vi "cesium_controller.vi"() -> ()   [LabVIEW 2013]
doc: "This is the main code used to run experiments in the Cesium laboratory of Mark Saffman. It was written by Martin Lichtman from 2009 to 2012, with DDS drivers written by Alex Gill and Larry Isenhower.\n\nEach hardware section may be enabled and disabled separately. Experiments will finish when all hardware has completed, or when the \"experiment timeout\" is reached, whichever comes first."
uses:
  <vilib>/Utility/error.llb/DialogType.ctl
  <vilib>/Utility/file.llb/Read From Spreadsheet File (string).vi
  <vilib>/Utility/file.llb/Write To Spreadsheet File (string).vi
  Camera/Hamamatsu_C9100-13/Hamamatsu_C9100-13.lvclass
  Experiment/Experiment.lvclass
  DDS/DDS.lvclass
  gui_refnum.ctl
  Counter/counter_graph_refnums.ctl
  gui_execution_controls.ctl
  ExperimentVariables/Variable_Settings.ctl
  ExperimentVariables/ExperimentVariables.lvclass
  <instrlib>/niHSDIO/niHSDIO.llb/niHSDIO_ctl Trigger Script - trigID Values (Ring).ctl
  <instrlib>/niHSDIO/niHSDIO.llb/niHSDIO_ctl Trigger Source Values (Ring).ctl
  <instrlib>/niHSDIO/niHSDIO.llb/niHSDIO_ctl Trigger DigEdge - Edge Values (Ring).ctl
  <instrlib>/niHSDIO/niHSDIO.llb/niHSDIO_ctl Trigger DigLvl - Level Values (Ring).ctl
  HSDIO/HSDIO_settings.ctl
  HSDIO/HSDIO.lvclass
  DAQmx_pulse_out/settings.ctl
  DAQmx_pulse_out/DAQmx_pulse_out.lvclass
  <vilib>/ni845x/ni845x.llb/ni845xControl.ctl
  DDS drivers v3/DDS_box_device_reference.ctl
  DDS drivers v3/DDS RAM mode.ctl
  DDS drivers v3/DDS_box_cluster.ctl
  DDS drivers v3/Array_of_DDS_Boxes.ctl
  DDS/DDS_Settings_Cluster.ctl
  Camera/Hamamatsu_C9100-13/camera_setup.ctl
  Counter/Counter_Settings_Control.ctl
  Counter/Counter.lvclass
  filters/filters.ctl
  Analog_output/AO_settings.ctl
  Analog_output/Analog_Output.lvclass
  config_file_io/all_settings.ctl
  GPIB/HP83623A_RF_Generator/HP83623A_RF_Generator.lvclass
  GPIB/HP83623A_RF_Generator/HP83623A_array.ctl
  PI_piezo/PI_Piezo.lvclass
  PI_piezo/settings.ctl
  Camera/Andor/Andor_settings.ctl
  <vilib>/gmath/NI_Gmath.lvlib
  gui/measurement_graph.ctl
  GPIB/HP8662A_RF_Generator/HP8662A_RF_Generator.lvclass
  GPIB/RF_Generator_settings.ctl
  GPIB/GPIB.lvclass
  GPIB/RF_Generator_settings_array.ctl
  DDS drivers v3/DDS_profile.ctl
  DDS drivers v3/DDS_channel.ctl
  DDS drivers v3/array_of_DDS_profiles.ctl
  DDS drivers v3/array_of_DDS_channels.ctl
  GPIB/HP83712B_RF_Generator/HP83712B_RF_Generator.lvclass
  TTL_input/TTL_input_settings.ctl
  TTL_input/TTL_input.lvclass
  HSDIO/waveform.ctl
  Experiment/Globals.vi
  <vilib>/Utility/file.llb/Write To Spreadsheet File (DBL).vi
  PI_piezo/piezo_channel.ctl
  PI_piezo/piezo_controller.ctl
  GPIB/HP83623A_RF_Generator/HP83623A.ctl
  histogram.ctl
  PI_piezo/status.ctl
panel:
  out "laser unlocked":bool
  out "Paused after Measurement":bool
  in  "Continue":bool
  in  "Pause after Iteration":bool
  out "Paused after Iteration":bool
  in  "Save Settings":bool
  in  "Load Settings":bool
  out "Background Array":u16[][](array[numeric])
  in  "Pause after Measurement":bool
  in  "Quit Program":bool
  in  "Run Experiment":bool
  in  "Tab Control":T1(tab)
  out "Variables (Indicator)":string[][](table)=[["a", "0.000", "0", "9172.612"], ["b", "0.000", "0", "9192.632"], ["k6", "0.000", "0", "0.100"], ["d", "2.000", "10", "40.000"]]
  out "Total Iterations":u32=11
  out "Current Iteration":u32=10
  out "Current measurement":u32=99
  out "wait loops":u32=42 caption="loops while waiting for \nexperiment to complete"
  in  "Log":string="2013-06-14 18:41:57 Experiment ended\n\n2013-06-14 18:41:38 Saving log.\n\n2013-06-14 18:13:43 Experiment started\n\n2013-06-14 17:57:15 Experiment ended\n\n2013-06-14 17:56:56 Saving log.\n\n2013-06-14 17:43:06 Experiment started\n\n2013-06-14 17:24:56 Experiment ended\n\n2013-06-14 17:24:35 Saving log.\n\n2013-06-14 17:10:22 Experiment started\n\n2013-06-14 17:05:48 Experiment ended\n\n2013-06-14 17:05:28 Experiment started\n\n2013-06-14 16:54:16 Experiment ended\n\n2013-06-14 16:52:09 Experiment started\n\n2013-06-14 16:47:56 Experiment ended\n\n2013-06-14 16:45:44 Experiment started\n\n2013-06-14 16:45:42 Experiment ended\n\n2013-06-14 16:43:02 Experiment started\n\n2013-06-14 16:43:01 Experiment ended\n\n2013-06-14 16:42:47 Saving log.\n\n2013-06-14 16:34:29 Experiment started\n\n2013-06-14 16:31:17 Experiment ended\n\n2013-06-14 16:30:59 Saving log.\n\n2013-06-14 16:17:10 Experiment started\n\n2013-06-14 16:17:09 Experiment ended\n\n2013-06-14 16:17:02 Saving log.\n\n2013-06-14 16:16:34 Experiment started\n\n2013-06-14 16:06:13 Experiment ended\n\n2013-06-14 16:06:06 Saving log.\n\n2013-06-14 15:58:25 Experiment started\n\n2013-06-14 15:48:18 Experiment ended\n\n2013-06-14 15:47:53 Experiment started\n\n2013-06-14 15:47:47 Experiment ended\n\n2013-06-14 15:47:28 Experiment started\n\n2013-06-14 15:47:27 Experiment ended\n\n2013-06-14 15:47:11 Experiment started\n\n2013-06-14 15:47:07 Experiment ended\n\n2013-06-14 15:46:48 Experiment started\n\n2013-06-14 15:46:35 Experiment ended\n\n2013-06-14 15:46:15 Experiment started\n\n2013-06-14 15:46:11 Experiment ended\n\n2013-06-14 15:38:57 Experiment started\n\n2013-06-14 15:37:18 Experiment ended\n\n2013-06-14 15:36:58 Experiment started\n\n2013-06-14 15:36:56 Experiment ended\n\n2013-06-14 15:35:05 Experiment started\n\n2013-06-14 15:35:04 Experiment ended\n\n2013-06-14 15:34:46 Experiment started\n\n2013-06-14 15:30:55 Experiment ended\n\n2013-06-14 15:30:47 Saving log.\n\n2013-06-14 15:29:21 Experiment started\n\n2013-06-14 15:29:20 Experiment ended\n\n2013-06-14 15:28:00 Experiment started\n\n2013-06-14 15:27:15 Experiment ended\n\n2013-06-14 15:26:46 Experiment started\n\n2013-06-14 15:25:16 Experiment ended\n\n2013-06-14 15:24:42 Experiment started\n\n2013-06-14 15:23:44 Experiment ended\n\n2013-06-14 15:23:14 Experiment started\n\n2013-06-14 15:22:27 Experiment ended\n\n2013-06-14 15:22:05 Experiment started\n\n2013-06-14 15:21:52 Error cleared and continued by user\n\n2013-06-14 15:21:49 Error -1074115612 occurred at niHSDIO Write Script.vi\r\n\r\nPossible reason(s):\nDriver Status:  (Hex 0xBFFA4BE4) Keyword was expected, but not found in the script.\n\nLine Number: 54\nPosition in Line: 1\nBad Value: compressredGenerate\nPossible Keywords: end\n\nStatus Code: -200027\nCall chain:\nhandle_errors.vi cesium_controller.vi\r\n\n\n2013-06-14 15:21:49 Experiment ended\n\n2013-06-14 15:21:43 Saving log.\n\n2013-06-14 15:21:22 Experiment started\n\n2013-06-14 15:20:53 Experiment ended\n\n2013-06-14 15:20:29 Experiment started\n\n2013-06-14 15:19:36 Experiment ended\n\n2013-06-14 15:18:32 Experiment started\n\n2013-06-14 15:15:07 Experiment ended\n\n2013-06-14 15:14:57 Saving log.\n\n2013-06-14 15:09:28 Experiment started\n\n2013-06-14 15:08:32 Experiment ended\n\n2013-06-14 15:08:22 Saving log.\n\n2013-06-14 15:03:52 Experiment started\n\n2013-06-14 14:59:10 Experiment ended\n\n2013-06-14 14:58:58 Saving log.\n\n2013-06-14 14:52:07 Experiment started\n\n2013-06-14 14:51:15 Experiment ended\n\n2013-06-14 14:51:04 Saving log.\n\n2013-06-14 14:44:44 Experiment started\n\n2013-06-14 14:44:39 Experiment ended\n\n2013-06-14 14:44:25 Saving log.\n\n2013-06-14 14:33:47 Experiment started\n\n2013-06-14 14:32:54 Error cleared and continued by user\n\n2013-06-14 14:32:53 Error -23091 occurred at Inconsistency in variables or numbers\r\n\r\nPossible reason(s):\n\r\nAnalysis:  Inconsistency in variables or numbers.\nCall chain:\nhandle_errors.vi cesium_controller.vi\r\n\n\n2013-06-14 14:32:38 Error cleared and continued by user\n\n2013-06-14 14:32:32 Error -23091 occurred at Inconsistency in variables or numbers\r\n\r\nPossible reason(s):\n\r\nAnalysis:  Inconsistency in variables or numbers.\nCall chain:\nhandle_errors.vi cesium_controller.vi\r\n\n\n2013-06-14 14:31:17 Error cleared and continued by user\n\n2013-06-14 14:31:16 Error -23091 occurred at Inconsistency in variables or numbers\r\n\r\nPossible reason(s):\n\r\nAnalysis:  Inconsistency in variables or numbers.\nCall chain:\nhandle_errors.vi cesium_controller.vi\r\n\n\n2013-06-14 14:31:16 Error cleared and continued by user\n\n2013-06-14 14:31:12 Error -23091 occurred at Inconsistency in variables or numbers\r\n\r\nPossible reason(s):\n\r\nAnalysis:  Inconsistency in variables or numbers.\nCall chain:\nhandle_errors.vi cesium_controller.vi\r\n\n\n2013-06-14 14:30:06 Error cleared and continued by user\n\n2013-06-14 14:29:53 Error -23091 occurred at Inconsistency in variables or numbers\r\n\r\nPossible reason(s):\n\r\nAnalysis:  Inconsistency in variables or numbers.\nCall chain:\nhandle_errors.vi cesium_controller.vi\r\n\n\n2013-06-14 14:29:53 Experiment ended\n\n2013-06-14 14:29:47 Saving log.\n\n2013-06-14 14:29:43 Experiment started\n\n2013-06-14 14:26:56 Error cleared and continued by user\n\n2013-06-14 14:26:55 Error -23091 occurred at Inconsistency in variables or numbers\r\n\r\nPossible reason(s):\n\r\nAnalysis:  Inconsistency in variables or numbers.\nCall chain:\nhandle_errors.vi cesium_controller.vi\r\n\n\n2013-06-14 14:26:37 Error cleared and continued by user\n\n2013-06-14 14:26:28 Error -23091 occurred at Inconsistency in variables or numbers\r\n\r\nPossible reason(s):\n\r\nAnalysis:  Inconsistency in variables or numbers.\nCall chain:\nhandle_errors.vi cesium_controller.vi\r\n\n\n2013-06-14 14:24:46 Error cleared and continued by user\n\n2013-06-14 14:24:44 Error -23091 occurred at Inconsistency in variables or numbers\r\n\r\nPossible reason(s):\n\r\nAnalysis:  Inconsistency in variables or numbers.\nCall chain:\nhandle_errors.vi cesium_controller.vi\r\n\n\n2013-06-14 14:24:44 Experiment ended\n\n2013-06-14 14:24:38 Saving log.\n\n2013-06-14 14:24:36 Experiment started\n\n2013-06-14 14:24:18 Error cleared and continued by user\n\n2013-06-14 14:24:16 Error -23091 occurred at Inconsistency in variables or numbers\r\n\r\nPossible reason(s):\n\r\nAnalysis:  Inconsistency in variables or numbers.\nCall chain:\nhandle_errors.vi cesium_controller.vi\r\n\n\n2013-06-14 14:24:07 Error cleared and continued by user\n\n2013-06-14 14:24:04 Error -23091 occurred at Inconsistency in variables or numbers\r\n\r\nPossible reason(s):\n\r\nAnalysis:  Inconsistency in variables or numbers.\nCall chain:\nhandle_errors.vi cesium_controller.vi\r\n\n\n2013-06-14 14:14:57 Experiment ended\n\n2013-06-14 14:14:41 Saving log.\n\n2013-06-14 14:01:54 Experiment started\n\n2013-06-14 14:01:45 Experiment ended\n\n2013-06-14 14:01:28 Saving log.\n\n2013-06-14 13:47:44 Experiment started\n\n2013-06-14 13:41:39 Experiment ended\n\n2013-06-14 13:41:31 Saving log.\n\n2013-06-14 13:39:59 Experiment started\n\n2013-06-14 13:39:57 Experiment ended\n\n2013-06-14 13:39:50 Saving log.\n\n2013-06-14 13:38:17 Experiment started\n\n2013-06-14 13:25:54 Experiment ended\n\n2013-06-14 13:25:39 Saving log.\n\n2013-06-14 13:14:23 Experiment started\n\n2013-06-14 13:01:58 Experiment ended\n\n2013-06-14 13:01:39 Saving log.\n\n2013-06-14 12:46:16 Experiment started\n\n2013-06-14 12:36:06 Experiment ended\n\n2013-06-14 12:35:53 Saving log.\n\n2013-06-14 12:28:42 Experiment started\n\n2013-06-14 12:20:45 Experiment ended\n\n2013-06-14 12:20:37 Saving log.\n\n2013-06-14 12:19:04 Experiment started\n\n2013-06-14 12:14:08 Experiment ended\n\n2013-06-14 12:14:00 Saving log.\n\n2013-06-14 12:12:31 Experiment started\n\n2013-06-14 12:12:30 Experiment ended\n\n2013-06-14 12:00:34 Experiment started\n\n2013-06-14 11:57:46 Experiment ended\n\n2013-06-14 11:57:38 Saving log.\n\n2013-06-14 11:56:10 Experiment started\n\n2013-06-14 11:47:52 Experiment ended\n\n2013-06-14 11:47:44 Saving log.\n\n2013-06-14 11:46:18 Experiment started\n\n2013-06-14 10:06:01 Experiment ended\n\n2013-06-14 10:05:53 Saving log.\n\n2013-06-14 10:04:24 Experiment started\n\n2013-06-14 10:01:43 Experiment ended\n\n2013-06-14 10:01:02 Experiment started\n\n2013-06-14 10:00:58 Experiment ended\n\n2013-06-14 10:00:35 Experiment started\n\n2013-06-14 08:10:42 Experiment ended\n\n2013-06-14 08:10:20 Experiment started\n\n2013-06-14 08:09:56 Experiment ended\n\n2013-06-14 08:08:35 Experiment started\n\n2013-06-14 08:08:06 Experiment ended\n\n2013-06-14 08:07:44 Experiment started\n\n2013-06-14 07:58:21 Experiment ended\n\n2013-06-14 07:51:44 Experiment started\n\n2013-06-13 21:30:01 Experiment ended\n\n2013-06-13 21:29:35 Experiment started\n\n2013-06-13 21:29:31 Experiment ended\n\n2013-06-13 21:29:05 Experiment started\n\n2013-06-13 21:28:52 Experiment ended\n\n2013-06-13 21:28:29 Experiment started\n\n2013-06-13 21:28:26 Experiment ended\n\n2013-06-13 21:28:05 Experiment started\n\n2013-06-13 21:26:16 Experiment ended\n\n2013-06-13 21:25:49 Experiment started\n\n2013-06-13 21:25:39 Experiment ended\n\n2013-06-13 21:25:13 Experiment started\n\n2013-06-13 21:25:12 Experiment ended\n\n2013-06-13 21:24:51 Experiment started\n\n2013-06-13 21:24:48 Experiment ended\n\n2013-06-13 21:24:26 Experiment started\n\n2013-06-13 21:24:15 Experiment ended\n\n2013-06-13 21:23:50 Experiment started\n\n2013-06-13 21:23:37 Experiment ended\n\n2013-06-13 21:23:15 Experiment started\n\n2013-06-13 21:23:14 Experiment ended\n\n2013-06-13 21:22:51 Experiment started\n\n2013-06-13 21:22:42 Experiment ended\n\n2013-06-13 21:22:19 Experiment started\n\n2013-06-13 21:22:18 Experiment ended\n\n2013-06-13 21:21:56 Experiment started\n\n2013-06-13 21:21:53 Experiment ended\n\n2013-06-13 21:21:17 Experiment started\n\n2013-06-13 21:21:17 Experiment ended\n\n2013-06-13 21:20:56 Experiment started\n\n2013-06-13 21:20:56 Experiment ended\n\n2013-06-13 21:20:32 Experiment started\n\n2013-06-13 21:20:29 Experiment ended\n\n2013-06-13 21:17:58 Experiment started\n\n2013-06-13 21:17:48 Experiment ended\n\n2013-06-13 21:04:43 Experiment started\n\n2013-06-13 21:04:41 Experiment ended\n\n2013-06-13 20:50:48 Experiment started\n\n2013-06-13 20:50:35 Experiment ended\n\n2013-06-13 20:50:02 Experiment started\n\n2013-06-13 20:49:42 Experiment ended\n\n2013-06-13 20:48:06 Experiment started\n\n2013-06-13 20:47:30 Experiment ended\n\n2013-06-13 20:45:37 Experiment started\n\n2013-06-13 20:45:31 Experiment ended\n\n2013-06-13 20:31:50 Experiment started\n\n2013-06-13 20:29:58 Experiment ended\n\n2013-06-13 20:27:00 Experiment started\n\n2013-06-13 20:26:57 Experiment ended\n\n2013-06-13 20:11:15 Experiment started\n\n2013-06-13 20:11:13 Experiment ended\n\n2013-06-13 20:09:50 Experiment started\n\n2013-06-13 20:09:33 Experiment ended\n\n2013-06-13 20:03:38 Experiment started\n\n2013-06-13 20:03:25 Experiment ended\n\n2013-06-13 20:03:19 Saving log.\n\n2013-06-13 20:01:48 Experiment started\n\n2013-06-13 20:01:48 Experiment ended\n\n2013-06-13 19:57:41 Experiment started\n\n2013-06-13 19:57:40 Experiment ended\n\n2013-06-13 19:53:03 Experiment started\n\n2013-06-13 19:52:47 Experiment ended\n\n2013-06-13 19:52:01 Experiment started\n\n2013-06-13 19:51:26 Experiment ended\n\n2013-06-13 19:51:00 Experiment started\n\n2013-06-13 19:49:32 Experiment ended\n\n2013-06-13 19:46:50 Experiment started\n\n2013-06-13 19:46:42 Experiment ended\n\n2013-06-13 19:46:17 Experiment started\n\n2013-06-13 19:46:11 Experiment ended\n\n2013-06-13 19:45:40 Experiment started\n\n2013-06-13 19:45:39 Experiment ended\n\n2013-06-13 19:45:16 Experiment started\n\n2013-06-13 19:45:04 Experiment ended\n\n2013-06-13 19:44:37 Experiment started\n\n2013-06-13 19:44:36 Experiment ended\n\n2013-06-13 19:44:07 Experiment started\n\n2013-06-13 19:44:02 Experiment ended\n\n2013-06-13 19:43:37 Experiment started\n\n2013-06-13 19:43:33 Experiment ended\n\n2013-06-13 19:39:17 Experiment started\n\n2013-06-13 19:39:07 Experiment ended\n\n2013-06-13 19:38:47 Experiment started\n\n2013-06-13 19:38:45 Experiment ended\n\n2013-06-13 19:38:24 Experiment started\n\n2013-06-13 19:38:23 Experiment ended\n\n2013-06-13 19:37:59 Experiment started\n\n2013-06-13 19:37:26 Experiment ended\n\n2013-06-13 19:36:47 Experiment started\n\n2013-06-13 19:36:39 Experiment ended\n\n2013-06-13 19:36:17 Experiment started\n\n2013-06-13 19:36:13 Experiment ended\n\n2013-06-13 19:35:50 Experiment started\n\n2013-06-13 19:35:47 Experiment ended\n\n2013-06-13 19:35:21 Experiment started\n\n2013-06-13 19:35:18 Experiment ended\n\n2013-06-13 19:34:55 Experiment started\n\n2013-06-13 19:34:50 Experiment ended\n\n2013-06-13 19:34:28 Experiment started\n\n2013-06-13 19:34:20 Experiment ended\n\n2013-06-13 19:33:51 Experiment started\n\n2013-06-13 19:33:46 Experiment ended\n\n2013-06-13 19:33:17 Experiment started\n\n2013-06-13 19:32:33 Experiment ended\n\n2013-06-13 19:32:05 Experiment started\n\n2013-06-13 19:31:47 Experiment ended\n\n2013-06-13 19:29:25 Experiment started\n\n2013-06-13 19:29:24 Experiment ended\n\n2013-06-13 19:28:58 Experiment started\n\n2013-06-13 19:28:56 Experiment ended\n\n2013-06-13 19:11:37 Experiment started\n\n2013-06-13 19:11:28 Experiment ended\n\n2013-06-13 19:10:59 Experiment started\n\n2013-06-13 19:10:58 Experiment ended\n\n2013-06-13 19:10:51 Saving log.\n\n2013-06-13 19:10:42 Experiment started\n\n2013-06-13 19:06:42 Experiment ended\n\n2013-06-13 19:06:12 Experiment started\n\n2013-06-13 19:05:06 Experiment ended\n\n2013-06-13 19:05:00 Saving log.\n\n2013-06-13 19:04:43 Experiment started\n\n2013-06-13 18:59:49 Experiment ended\n\n2013-06-13 18:59:18 Experiment started\n\n2013-06-13 18:58:51 Experiment ended\n\n2013-06-13 18:57:59 Experiment started\n\n2013-06-13 18:57:35 Experiment ended\n\n2013-06-13 18:57:04 Experiment started\n\n2013-06-13 18:53:16 Experiment ended\n\n2013-06-13 18:53:07 Saving log.\n\n2013-06-13 18:51:24 Experiment started\n\n2013-06-13 18:50:48 Experiment ended\n\n2013-06-13 18:48:35 Experiment started\n\n2013-06-13 18:48:30 Experiment ended\n\n2013-06-13 18:48:22 Saving log.\n\n2013-06-13 18:46:48 Experiment started\n\n2013-06-13 17:36:18 Experiment ended\n\n2013-06-13 17:36:11 Saving log.\n\n2013-06-13 17:34:42 Experiment started\n\n2013-06-13 17:21:41 Experiment ended\n\n2013-06-13 17:21:32 Saving log.\n\n2013-06-13 17:18:38 Experiment started\n\n2013-06-13 17:18:06 Experiment ended\n\n2013-06-13 17:17:26 Experiment started\n\n2013-06-13 17:14:33 Experiment ended\n\n2013-06-13 17:12:16 Experiment started\n\n2013-06-13 17:12:03 Experiment ended\n\n2013-06-13 17:05:54 Experiment started\n\n2013-06-13 17:05:34 Experiment ended\n\n2013-06-13 16:56:19 Experiment started\n\n2013-06-13 16:54:33 Experiment ended\n\n2013-06-13 16:52:53 Experiment started\n\n2013-06-13 16:18:42 Experiment ended\n\n2013-06-13 16:16:57 Experiment started\n\n2013-06-13 15:33:32 Experiment ended\n\n2013-06-13 15:28:31 Experiment started\n\n2013-06-13 15:28:05 Experiment ended\n\n2013-06-13 15:27:40 Experiment started\n\n2013-06-13 15:27:21 Experiment ended\n\n2013-06-13 15:26:36 Experiment started\n\n2013-06-13 15:20:15 Experiment ended\n\n2013-06-13 15:19:58 Experiment started\n\n2013-06-13 15:00:57 Experiment ended\n\n2013-06-13 15:00:29 Saving log.\n\n2013-06-13 14:46:45 Experiment started\n\n2013-06-13 14:44:33 Experiment ended\n\n2013-06-13 14:44:04 Saving log.\n\n2013-06-13 14:30:24 Experiment started\n\n2013-06-13 14:26:48 Experiment ended\n\n2013-06-13 14:26:19 Saving log.\n\n2013-06-13 14:11:24 Experiment started\n\n2013-06-13 14:10:02 Experiment ended\n\n2013-06-13 14:09:32 Experiment started\n\n2013-06-13 14:09:07 Experiment ended\n\n2013-06-13 14:08:38 Experiment started\n\n2013-06-13 14:08:16 Experiment ended\n\n2013-06-13 14:05:43 Experiment started\n\n2013-06-13 14:05:28 Experiment ended\n\n2013-06-13 13:44:43 Experiment started\n\n2013-06-13 13:44:40 Experiment ended\n\n2013-06-13 13:33:41 Experiment started\n\n2013-06-13 13:33:36 Experiment ended\n\n2013-06-13 13:20:13 Experiment started\n\n2013-06-13 13:20:07 Experiment ended\n\n2013-06-13 13:18:37 Experiment started\n\n2013-06-13 13:09:49 Experiment ended\n\n2013-06-13 13:09:21 Saving log.\n\n2013-06-13 12:53:17 Experiment started\n\n2013-06-13 12:53:06 Experiment ended\n\n2013-06-13 12:52:59 Saving log.\n\n2013-06-13 12:51:30 Experiment started\n\n2013-06-13 12:45:06 Experiment ended\n\n2013-06-13 12:44:42 Saving log.\n\n2013-06-13 12:28:03 Experiment started\n\n2013-06-13 12:27:00 Experiment ended\n\n2013-06-13 12:26:33 Saving log.\n\n2013-06-13 12:12:01 Experiment started\n\n2013-06-13 11:48:49 Experiment ended\n\n2013-06-13 11:48:23 Saving log.\n\n2013-06-13 11:24:55 Experiment started\n\n2013-06-13 11:24:49 Experiment ended\n\n2013-06-13 11:24:25 Saving log.\n\n2013-06-13 11:04:09 Experiment started\n\n2013-06-13 11:00:29 Experiment ended\n\n2013-06-13 10:58:28 Experiment started\n\n2013-06-13 10:57:29 Experiment ended\n\n2013-06-13 10:57:10 Experiment started\n\n2013-06-13 10:55:38 Experiment ended\n\n2013-06-13 10:55:12 Saving log.\n\n2013-06-13 10:38:00 Experiment started\n\n2013-06-13 10:32:10 Experiment ended\n\n2013-06-13 10:31:44 Saving log.\n\n2013-06-13 10:14:40 Experiment started\n\n2013-06-13 10:13:05 Experiment ended\n\n2013-06-13 10:11:33 Experiment started\n\n2013-06-13 10:09:51 Experiment ended\n\n2013-06-13 10:09:22 Saving log.\n\n2013-06-13 09:50:30 Experiment started\n\n2013-06-13 09:48:31 Experiment ended\n\n2013-06-13 09:48:05 Saving log.\n\n2013-06-13 09:28:50 Experiment started\n\n2013-06-13 09:26:19 Experiment ended\n\n2013-06-13 09:25:52 Saving log.\n\n2013-06-13 09:01:32 Experiment started\n\n2013-06-13 09:01:28 Experiment ended\n\n2013-06-13 09:01:21 Saving log.\n\n2013-06-13 09:01:10 Experiment started\n\n2013-06-13 09:00:30 Experiment ended\n\n2013-06-13 09:00:03 Experiment started\n\n2013-06-13 08:56:26 Experiment ended\n\n2013-06-13 08:56:04 Experiment started\n\n2013-06-13 08:55:34 Experiment ended\n\n2013-06-13 08:55:09 Experiment started\n\n2013-06-13 08:53:19 Experiment ended\n\n2013-06-13 08:52:21 Experiment started\n\n2013-06-13 08:52:07 Experiment ended\n\n2013-06-13 08:50:25 Experiment started\n\n2013-06-13 08:49:44 Experiment ended\n\n2013-06-13 08:49:19 Saving log.\n\n2013-06-13 08:28:57 Experiment started\n\n2013-06-13 08:09:55 Experiment ended\n\n2013-06-13 08:09:36 Saving log.\n\n2013-06-13 07:59:34 Experiment started\n\n2013-06-13 07:57:57 Experiment ended\n\n2013-06-13 07:57:44 Saving log.\n\n2013-06-13 07:50:13 Experiment started\n\n2013-06-13 07:48:57 Experiment ended\n\n2013-06-13 07:48:42 Saving log.\n\n2013-06-13 07:41:10 Experiment started\n\n2013-06-13 07:40:55 Experiment ended\n\n2013-06-13 07:39:57 Experiment started\n\n2013-06-13 07:38:18 Experiment ended\n\n2013-06-13 07:38:05 Saving log.\n\n2013-06-13 07:30:34 Experiment started\n\n2013-06-13 07:30:18 Experiment ended\n\n2013-06-13 07:30:04 Saving log.\n\n2013-06-13 07:22:34 Experiment started\n\n2013-06-13 07:22:24 Experiment ended\n\n2013-06-13 07:22:17 Saving log.\n\n2013-06-13 07:21:33 Experiment started\n\n2013-06-13 07:17:18 Experiment ended\n\n2013-06-13 07:17:12 Saving log.\n\n2013-06-13 07:15:55 Experiment started\n\n2013-06-13 07:14:54 Experiment ended\n\n2013-06-13 07:14:48 Saving log.\n\n2013-06-13 07:13:28 Experiment started\n\n2013-06-13 07:10:19 Experiment ended\n\n2013-06-13 07:10:11 Saving log.\n\n2013-06-13 07:07:40 Experiment started\n\n2013-06-13 07:07:38 Experiment ended\n\n2013-06-13 07:07:31 Saving log.\n\n2013-06-13 07:05:59 Experiment started\n\n2013-06-13 07:02:16 Load settings was cancelled, file did not exist, or error.\n\n2013-06-12 21:24:07 Experiment ended\n\n2013-06-12 21:23:13 Experiment started\n\n2013-06-12 21:22:56 Experiment ended\n\n2013-06-12 21:21:22 Experiment started\n\n2013-06-12 21:21:13 Experiment ended\n\n2013-06-12 21:04:14 Experiment started\n\n2013-06-12 21:03:42 Experiment ended\n\n2013-06-12 21:03:16 Experiment started\n\n2013-06-12 21:03:08 Experiment ended\n\n2013-06-12 21:02:54 Experiment started\n\n2013-06-12 21:02:32 Experiment ended\n\n2013-06-12 21:02:00 Experiment started\n\n2013-06-12 21:00:24 Experiment ended\n\n2013-06-12 20:59:48 Experiment started\n\n2013-06-12 20:57:52 Experiment ended\n\n2013-06-12 20:56:43 Experiment started\n\n2013-06-12 20:55:55 Experiment ended\n\n2013-06-12 20:55:24 Experiment started\n\n2013-06-12 20:55:12 Experiment ended\n\n2013-06-12 20:54:45 Experiment started\n\n2013-06-12 20:46:38 Experiment ended\n\n2013-06-12 20:44:34 Experiment started\n\n2013-06-12 20:41:51 Experiment started\n\n2013-06-12 20:39:43 Experiment ended\n\n2013-06-12 20:39:10 Experiment started\n\n2013-06-12 20:39:06 Experiment ended\n\n2013-06-12 20:38:38 Experiment started\n\n2013-06-12 20:38:35 Experiment ended\n\n2013-06-12 20:38:14 Experiment started\n\n2013-06-12 18:40:17 Experiment ended\n\n2013-06-12 18:40:10 Saving log.\n\n2013-06-12 18:39:04 Experiment started\n\n2013-06-12 18:37:07 Experiment ended\n\n2013-06-12 18:36:36 Saving log.\n\n2013-06-12 18:23:01 Experiment started\n\n2013-06-12 18:17:45 Experiment ended\n\n2013-06-12 18:17:12 Saving log.\n\n2013-06-12 17:52:48 Experiment started\n\n2013-06-12 17:51:07 Experiment ended\n\n2013-06-12 17:50:52 Experiment started\n\n2013-06-12 17:50:07 Experiment ended\n\n2013-06-12 17:49:15 Experiment started\n\n2013-06-12 17:28:45 Experiment ended\n\n2013-06-12 16:56:47 Experiment started\n\n2013-06-12 16:56:01 Experiment ended\n\n2013-06-12 16:55:43 Experiment started\n\n2013-06-12 15:58:27 Experiment ended\n\n2013-06-12 15:58:09 Saving log.\n\n2013-06-12 15:48:07 Experiment started\n\n2013-06-12 15:47:03 Experiment ended\n\n2013-06-12 15:46:44 Experiment started\n\n2013-06-12 15:44:24 Experiment ended\n\n2013-06-12 15:44:06 Saving log.\n\n2013-06-12 15:36:44 Experiment started\n\n2013-06-12 15:36:42 Experiment ended\n\n2013-06-12 15:36:32 Saving log.\n\n2013-06-12 15:33:24 Experiment started\n\n2013-06-12 15:33:21 Experiment ended\n\n2013-06-12 15:33:12 Saving log.\n\n2013-06-12 15:30:30 Experiment started\n\n2013-06-12 15:30:19 Experiment ended\n\n2013-06-12 15:30:09 Saving log.\n\n2013-06-12 15:26:11 Experiment started\n\n2013-06-12 15:25:56 Experiment ended\n\n2013-06-12 15:25:37 Saving log.\n\n2013-06-12 15:14:32 Experiment started\n\n2013-06-12 15:13:58 Experiment ended\n\n2013-06-12 15:13:34 Saving log.\n\n2013-06-12 14:56:25 Experiment started\n\n2013-06-12 14:39:36 Experiment ended\n\n2013-06-12 14:39:03 Saving log.\n\n2013-06-12 14:25:31 Experiment started\n\n2013-06-12 14:20:53 Experiment ended\n\n2013-06-12 14:20:34 Saving log.\n\n2013-06-12 14:13:07 Experiment started\n\n2013-06-12 14:11:20 Experiment ended\n\n2013-06-12 14:11:02 Saving log.\n\n2013-06-12 14:02:48 Experiment started\n\n2013-06-12 13:57:55 Error cleared and continued by user\n\n2013-06-12 13:57:53 Error -2628 occurred at Invoke Node in NI_XML.lvlib:Load XML File.vi->load_settings.vi->cesium_controller.vi\r\n\r\nPossible reason(s):\n\r\nLabVIEW:  An error occurred while parsing the document.\nCall chain:\nhandle_errors.vi load_settings.vi cesium_controller.vi\r\n\n\n2013-06-12 13:51:07 Experiment ended\n\n2013-06-12 13:50:35 Saving log.\n\n2013-06-12 13:35:28 Experiment started\n\n2013-06-12 13:31:33 Experiment ended\n\n2013-06-12 13:30:57 Saving log.\n\n2013-06-12 13:17:26 Experiment started\n\n2013-06-12 13:04:39 Experiment ended\n\n2013-06-12 13:04:05 Saving log.\n\n2013-06-12 12:50:22 Experiment started\n\n2013-06-12 12:49:56 Experiment ended\n\n2013-06-12 12:49:23 Saving log.\n\n2013-06-12 12:33:30 Experiment started\n\n2013-06-12 12:27:18 Experiment ended\n\n2013-06-12 12:27:12 Saving log.\n\n2013-06-12 12:09:24 Experiment started\n\n2013-06-12 12:04:44 Experiment ended\n\n2013-06-12 12:04:37 Saving log.\n\n2013-06-12 11:59:37 Experiment started\n\n2013-06-12 11:58:49 Experiment ended\n\n2013-06-12 11:58:43 Saving log.\n\n2013-06-12 11:58:30 Experiment started\n\n2013-06-12 11:54:23 Experiment ended\n\n2013-06-12 11:53:56 Saving log.\n\n2013-06-12 11:32:26 Experiment started\n\n2013-06-12 11:27:41 Experiment ended\n\n2013-06-12 11:27:10 Saving log.\n\n2013-06-12 10:58:10 Experiment started\n\n2013-06-12 10:54:42 Experiment ended\n\n2013-06-12 10:54:14 Saving log.\n\n2013-06-12 10:33:44 Experiment started\n\n2013-06-12 10:28:48 Experiment ended\n\n2013-06-12 10:28:31 Saving log.\n\n2013-06-12 10:21:01 Experiment started\n\n2013-06-12 10:19:37 Experiment ended\n\n2013-06-12 10:19:18 Saving log.\n\n2013-06-12 10:11:42 Experiment started\n\n2013-06-12 10:10:16 Experiment ended\n\n2013-06-12 10:10:00 Saving log.\n\n2013-06-12 10:02:30 Experiment started\n\n2013-06-12 10:01:00 Experiment ended\n\n2013-06-12 10:00:44 Saving log.\n\n2013-06-12 09:53:15 Experiment started\n\n2013-06-12 09:43:56 Experiment ended\n\n2013-06-12 09:43:32 Saving log.\n\n2013-06-12 09:28:54 Experiment started\n\n2013-06-12 09:26:40 Experiment ended\n\n2013-06-12 09:26:21 Experiment started\n\n2013-06-12 09:26:01 Experiment ended\n\n2013-06-12 09:25:52 Saving log.\n\n2013-06-12 09:12:58 Experiment started\n\n2013-06-12 09:06:39 Experiment ended\n\n2013-06-12 09:06:24 Saving log.\n\n2013-06-12 08:56:46 Experiment started\n\n2013-06-12 08:53:04 Experiment ended\n\n2013-06-12 08:52:53 Saving log.\n\n2013-06-12 08:45:57 Experiment started\n\n2013-06-12 08:45:56 Experiment ended\n\n2013-06-12 08:45:49 Saving log.\n\n2013-06-12 08:45:03 Experiment started\n\n2013-06-12 08:44:08 Experiment ended\n\n2013-06-12 08:43:53 Experiment started\n\n2013-06-12 08:42:06 Experiment ended\n\n2013-06-12 08:41:35 Saving log.\n\n2013-06-12 08:22:35 Experiment started\n\n2013-06-12 08:22:34 Experiment ended\n\n2013-06-12 08:22:27 Saving log.\n\n2013-06-12 08:21:01 Experiment started\n\n2013-06-12 08:20:02 Experiment ended\n\n2013-06-12 08:19:56 Saving log.\n\n2013-06-12 08:17:24 Experiment started\n\n2013-06-12 08:15:35 Experiment ended\n\n2013-06-12 08:15:05 Saving log.\n\n2013-06-12 07:57:52 Experiment started\n\n2013-06-12 07:54:55 Experiment ended\n\n2013-06-12 07:54:40 Saving log.\n\n2013-06-12 07:45:16 Experiment started\n\n2013-06-12 07:41:54 Experiment ended\n\n2013-06-12 07:41:45 Saving log.\n\n2013-06-12 07:40:28 Experiment started\n\n2013-06-12 07:38:54 Experiment ended\n\n2013-06-12 07:38:44 Saving log.\n\n2013-06-12 07:35:24 Experiment started\n\n2013-06-12 07:33:47 Experiment ended\n\n2013-06-12 07:33:40 Saving log.\n\n2013-06-12 07:30:22 Experiment started\n\n2013-06-12 07:27:18 Experiment ended\n\n2013-06-12 07:27:08 Saving log.\n\n2013-06-12 07:22:53 Experiment started\n\n2013-06-12 07:13:35 Experiment ended\n\n2013-06-12 07:13:24 Saving log.\n\n2013-06-12 07:08:21 Experiment started\n\n2013-06-12 07:07:25 Experiment ended\n\n2013-06-12 07:07:18 Saving log.\n\n2013-06-12 07:06:02 Experiment started\n\n2013-06-12 07:05:36 Experiment ended\n\n2013-06-12 07:05:28 Saving log.\n\n2013-06-12 07:03:39 Experiment started\n\n2013-06-12 07:02:58 Error cleared and continued by user\n\n2013-06-12 07:02:56 Error -2628 occurred at Invoke Node in NI_XML.lvlib:Load XML File.vi->load_settings.vi->cesium_controller.vi\r\n\r\nPossible reason(s):\n\r\nLabVIEW:  An error occurred while parsing the document.\nCall chain:\nhandle_errors.vi load_settings.vi cesium_controller.vi\r\n\n\n2013-06-11 18:27:29 Experiment ended\n\n2013-06-11 18:27:20 Saving log.\n\n2013-06-11 18:21:51 Experiment started\n\n2013-06-11 17:15:11 Experiment ended\n\n2013-06-11 17:10:07 Experiment started\n\n2013-06-11 17:09:54 Experiment ended\n\n2013-06-11 17:09:45 Saving log.\n\n2013-06-11 17:06:26 Experiment started\n\n2013-06-11 16:57:53 Experiment ended\n\n2013-06-11 16:57:44 Saving log.\n\n2013-06-11 16:54:29 Experiment started\n\n2013-06-11 16:50:04 Experiment ended\n\n2013-06-11 16:49:34 Saving log.\n\n2013-06-11 16:30:57 Experiment started\n\n2013-06-11 16:30:04 Experiment ended\n\n2013-06-11 16:29:56 Saving log.\n\n2013-06-11 16:28:31 Experiment started\n\n2013-06-11 16:26:03 Experiment ended\n\n2013-06-11 16:25:36 Saving log.\n\n2013-06-11 16:06:48 Experiment started\n\n2013-06-11 15:59:31 Experiment ended\n\n2013-06-11 15:59:09 Experiment started\n\n2013-06-11 15:51:43 Experiment ended\n\n2013-06-11 15:51:24 Experiment started\n\n2013-06-11 15:44:00 Experiment ended\n\n2013-06-11 15:43:34 Saving log.\n\n2013-06-11 15:26:32 Experiment started\n\n2013-06-11 15:24:33 Experiment ended\n\n2013-06-11 15:19:21 Experiment started\n\n2013-06-11 15:17:58 Experiment ended\n\n2013-06-11 15:17:08 Saving log.\n\n2013-06-11 14:38:23 Experiment started\n\n2013-06-11 14:26:45 Experiment ended\n\n2013-06-11 14:25:52 Saving log.\n\n2013-06-11 13:48:31 Experiment started\n\n2013-06-11 13:44:59 Experiment ended\n\n2013-06-11 13:44:19 Saving log.\n\n2013-06-11 12:08:53 Experiment started\n\n2013-06-11 12:03:13 Experiment ended\n\n2013-06-11 12:02:34 Saving log.\n\n2013-06-11 11:16:39 Experiment started\n\n2013-06-11 11:16:15 Experiment ended\n\n2013-06-11 11:15:08 Experiment started\n\n2013-06-11 11:14:30 Experiment ended\n\n2013-06-11 11:12:21 Experiment started\n\n2013-06-11 11:11:55 Experiment ended\n\n2013-06-11 11:09:44 Experiment started\n\n2013-06-11 10:58:37 Experiment ended\n\n2013-06-11 10:57:58 Saving log.\n\n2013-06-11 10:12:05 Experiment started\n\n2013-06-11 10:04:16 Experiment ended\n\n2013-06-11 10:03:58 Experiment started\n\n2013-06-11 09:29:35 Experiment ended\n\n2013-06-11 09:29:09 Saving log.\n\n2013-06-11 09:04:24 Experiment started\n\n2013-06-11 08:59:24 Experiment ended\n\n2013-06-11 08:59:07 Saving log.\n\n2013-06-11 08:45:44 Experiment started\n\n2013-06-11 08:42:05 Experiment ended\n\n2013-06-11 08:41:49 Saving log.\n\n2013-06-11 08:28:21 Experiment started\n\n2013-06-11 08:27:42 Experiment ended\n\n2013-06-11 08:27:34 Saving log.\n\n2013-06-11 08:24:48 Experiment started\n\n2013-06-11 08:20:43 Experiment ended\n\n2013-06-11 08:20:29 Saving log.\n\n2013-06-11 08:09:58 Experiment started\n\n2013-06-11 08:07:56 Experiment ended\n\n2013-06-11 08:07:40 Saving log.\n\n2013-06-11 07:56:15 Experiment started\n\n2013-06-11 07:56:00 Error cleared and continued by user\n\n2013-06-11 07:55:58 Error -7 occurred at Data Receive (DLL) Timeout Error\nGCS Error: Timeout error\r\n\r\nThis error code is undefined. Undefined errors might occur for a number of reasons. For example, no one has provided a description for the code, or you might have wired a number that is not an error code to the error code input. \n\nAdditionally, undefined error codes might occur because the error relates to a third-party object, such as the operating system or ActiveX. For these third-party errors, you might be able to obtain a description of the error by searching the Web for the error code (-7) or for its hexadecimal representation (0xFFFFFFF9).\nCall chain:\nhandle_errors.vi cesium_controller.vi\r\n\n\n2013-06-11 07:55:58 Experiment ended\n\n2013-06-11 07:55:52 Saving log.\n\n2013-06-11 07:49:45 Experiment started\n\n2013-06-11 07:47:51 Experiment ended\n\n2013-06-11 07:47:39 Saving log.\n\n2013-06-11 07:37:38 Experiment started\n\n2013-06-11 07:37:26 Experiment ended\n\n2013-06-11 07:37:04 Saving log.\n\n2013-06-11 07:20:58 Experiment started\n\n2013-06-11 07:15:43 Experiment ended\n\n2013-06-11 07:15:35 Saving log.\n\n2013-06-11 07:11:37 Experiment started\n\n2013-06-11 07:03:16 Experiment ended\n\n2013-06-11 07:02:16 Experiment started\n\n2013-06-10 19:32:46 Experiment ended\n\n2013-06-10 19:32:23 Saving log.\n\n2013-06-10 19:12:39 Experiment started\n\n2013-06-10 19:12:29 Experiment ended\n\n2013-06-10 19:12:02 Saving log.\n\n2013-06-10 18:51:10 Experiment started\n\n2013-06-10 18:50:18 Experiment ended\n\n2013-06-10 18:49:14 Experiment started\n\n2013-06-10 18:48:28 Experiment ended\n\n2013-06-10 18:48:21 Saving log.\n\n2013-06-10 18:47:39 Experiment started\n\n2013-06-10 18:46:22 Experiment ended\n\n2013-06-10 18:45:19 Experiment started\n\n2013-06-10 18:15:25 Experiment ended\n\n2013-06-10 18:14:55 Saving log.\n\n2013-06-10 17:55:30 Experiment started\n\n2013-06-10 17:55:28 Experiment ended\n\n2013-06-10 17:55:07 Saving log.\n\n2013-06-10 17:41:48 Experiment started\n\n2013-06-10 17:41:40 Experiment ended\n\n2013-06-10 17:41:17 Saving log.\n\n2013-06-10 17:27:51 Experiment started\n\n2013-06-10 17:21:51 Experiment ended\n\n2013-06-10 17:21:17 Saving log.\n\n2013-06-10 16:05:28 Experiment started\n\n2013-06-10 16:01:18 Error cleared and continued by user\n\n2013-06-10 16:01:16 Error -2628 occurred at Invoke Node in NI_XML.lvlib:Load XML File.vi->load_settings.vi->cesium_controller.vi\r\n\r\nPossible reason(s):\n\r\nLabVIEW:  An error occurred while parsing the document.\nCall chain:\nhandle_errors.vi load_settings.vi cesium_controller.vi\r\n\n\n2013-06-10 15:59:07 Error cleared and continued by user\n\n2013-06-10 15:59:03 Error -2628 occurred at Invoke Node in NI_XML.lvlib:Load XML File.vi->load_settings.vi->cesium_controller.vi\r\n\r\nPossible reason(s):\n\r\nLabVIEW:  An error occurred while parsing the document.\nCall chain:\nhandle_errors.vi load_settings.vi cesium_controller.vi\r\n\n\n2013-06-10 14:46:29 Experiment ended\n\n2013-06-10 14:45:58 Saving log.\n\n2013-06-10 13:57:13 Experiment started\n\n2013-06-10 13:15:53 Experiment ended\n\n2013-06-10 13:15:37 Saving log.\n\n2013-06-10 13:02:06 Experiment started\n\n2013-06-10 13:01:24 Experiment ended\n\n2013-06-10 12:59:02 Experiment started\n\n2013-06-10 12:57:49 Experiment ended\n\n2013-06-10 12:57:31 Saving log.\n\n2013-06-10 12:44:05 Experiment started\n\n2013-06-10 12:43:16 Experiment ended\n\n2013-06-10 12:43:08 Saving log.\n\n2013-06-10 12:41:21 Experiment started\n\n2013-06-10 12:41:05 Experiment ended\n\n2013-06-10 12:40:53 Saving log.\n\n2013-06-10 12:31:10 Experiment started\n\n2013-06-10 12:31:07 Experiment ended\n\n2013-06-10 12:31:00 Saving log.\n\n2013-06-10 12:29:05 Experiment started\n\n2013-06-10 12:28:42 Experiment ended\n\n2013-06-10 12:26:52 Experiment started\n\n2013-06-10 12:26:51 Experiment ended\n\n2013-06-10 12:24:53 Experiment started\n\n2013-06-10 12:24:15 Experiment ended\n\n2013-06-10 12:21:52 Experiment started\n\n2013-06-10 12:18:07 Experiment ended\n\n2013-06-10 12:15:45 Experiment started\n\n2013-06-10 12:13:06 Experiment ended\n\n2013-06-10 12:10:42 Experiment started\n\n2013-06-10 12:09:49 Experiment ended\n\n2013-06-10 12:09:40 Saving log.\n\n2013-06-10 12:04:37 Experiment started\n\n2013-06-10 12:00:08 Experiment ended\n\n2013-06-10 11:59:50 Saving log.\n\n2013-06-10 11:44:18 Experiment started\n\n2013-06-10 11:34:57 Halted by user.\n\n2013-06-10 11:34:54 Error -2628 occurred at Invoke Node in NI_XML.lvlib:Load XML File.vi->load_settings.vi->cesium_controller.vi\r\n\r\nPossible reason(s):\n\r\nLabVIEW:  An error occurred while parsing the document.\nCall chain:\nhandle_errors.vi load_settings.vi cesium_controller.vi\r\n\n\n2013-06-10 11:30:35 Experiment ended\n\n2013-06-10 11:30:03 Saving log.\n\n2013-06-10 11:00:52 Experiment started\n\n2013-06-10 10:58:13 Experiment ended\n\n2013-06-10 10:57:50 Saving log.\n\n2013-06-10 10:43:02 Experiment started\n\n2013-06-10 10:42:08 Experiment ended\n\n2013-06-10 10:41:46 Saving log.\n\n2013-06-10 10:27:35 Experiment started\n\n2013-06-10 10:26:11 Experiment ended\n\n2013-06-10 10:25:50 Saving log.\n\n2013-06-10 10:13:27 Experiment started\n\n2013-06-10 10:13:15 Error cleared and continued by user\n\n2013-06-10 10:13:13 Error -23091 occurred at Inconsistency in variables or numbers\r\n\r\nPossible reason(s):\n\r\nAnalysis:  Inconsistency in variables or numbers.\nCall chain:\nhandle_errors.vi cesium_controller.vi\r\n\n\n2013-06-10 10:08:28 Experiment ended\n\n2013-06-10 10:08:04 Saving log.\n\n2013-06-10 09:54:00 Experiment started\n\n2013-06-10 09:51:08 Experiment ended\n\n2013-06-10 09:50:49 Saving log.\n\n2013-06-10 09:38:30 Experiment started\n\n2013-06-10 09:34:48 Experiment ended\n\n2013-06-10 09:34:31 Saving log.\n\n2013-06-10 09:21:16 Experiment started\n\n2013-06-10 09:20:32 Experiment ended\n\n2013-06-10 09:20:22 Saving log.\n\n2013-06-10 09:12:40 Experiment started\n\n2013-06-10 09:07:07 Experiment ended\n\n2013-06-10 09:06:39 Saving log.\n\n2013-06-10 08:48:21 Experiment started\n\n2013-06-10 08:42:06 Experiment ended\n\n2013-06-10 08:41:39 Saving log.\n\n2013-06-10 08:22:02 Experiment started\n\n2013-06-10 08:19:04 Experiment ended\n\n2013-06-10 08:18:46 Saving log.\n\n2013-06-10 08:05:02 Experiment started\n\n2013-06-10 08:03:04 Experiment ended\n\n2013-06-10 08:02:32 Saving log.\n\n2013-06-10 07:37:13 Experiment started\n\n2013-06-10 07:34:12 Experiment ended\n\n2013-06-10 07:33:56 Saving log.\n\n2013-06-10 07:22:57 Experiment started\n\n2013-06-10 07:15:47 Experiment ended\n\n2013-06-10 07:15:40 Saving log.\n\n2013-06-10 07:15:25 Experiment started\n\n2013-06-07 18:06:57 Experiment ended\n\n2013-06-07 18:06:02 Saving log.\n\n2013-06-07 16:44:59 Experiment started\n\n2013-06-07 16:44:36 Experiment ended\n\n2013-06-07 16:43:59 Saving log.\n\n2013-06-07 16:05:19 Experiment started\n\n2013-06-07 15:55:37 Experiment ended\n\n2013-06-07 15:55:11 Saving log.\n\n2013-06-07 15:35:43 Experiment started\n\n2013-06-07 15:33:18 Experiment ended\n\n2013-06-07 15:32:51 Saving log.\n\n2013-06-07 15:15:18 Experiment started\n\n2013-06-07 14:57:08 Experiment ended\n\n2013-06-07 14:56:46 Experiment started\n\n2013-06-07 14:56:45 Experiment ended\n\n2013-06-07 14:56:23 Experiment started\n\n2013-06-07 14:54:31 Experiment ended\n\n2013-06-07 14:54:04 Experiment started\n\n2013-06-07 14:54:00 Experiment ended\n\n2013-06-07 14:53:42 Experiment started\n\n2013-06-07 14:49:10 Experiment ended\n\n2013-06-07 14:48:19 Saving log.\n\n2013-06-07 14:03:12 Experiment started\n\n2013-06-07 13:59:27 Experiment ended\n\n2013-06-07 13:58:30 Saving log.\n\n2013-06-07 13:14:59 Experiment started\n\n2013-06-07 13:10:20 Experiment ended\n\n2013-06-07 13:09:50 Saving log.\n\n2013-06-07 12:50:29 Experiment started\n\n2013-06-07 12:45:10 Experiment ended\n\n2013-06-07 12:44:38 Saving log.\n\n2013-06-07 12:14:24 Experiment started\n\n2013-06-07 12:14:02 Experiment ended\n\n2013-06-07 12:11:07 Experiment started\n\n2013-06-07 12:02:24 Experiment ended\n\n2013-06-07 12:01:32 Saving log.\n\n2013-06-07 11:17:57 Experiment started\n\n2013-06-07 11:16:03 Experiment ended\n\n2013-06-07 11:15:44 Experiment started\n\n2013-06-07 11:04:03 Experiment ended\n\n2013-06-07 11:03:56 Saving log.\n\n2013-06-07 11:03:45 Experiment started\n\n2013-06-07 11:01:34 Experiment ended\n\n2013-06-07 11:01:17 Saving log.\n\n2013-06-07 10:47:31 Experiment started\n\n2013-06-07 10:41:22 Experiment ended\n\n2013-06-07 10:41:14 Saving log.\n\n2013-06-07 10:39:28 Experiment started\n\n2013-06-07 10:39:19 Experiment ended\n\n2013-06-07 10:38:53 Saving log.\n\n2013-06-07 10:14:28 Experiment started\n\n2013-06-07 10:11:24 Experiment ended\n\n2013-06-07 10:10:54 Saving log.\n\n2013-06-07 09:45:59 Experiment started\n\n2013-06-07 09:38:25 Experiment ended\n\n2013-06-07 09:37:55 Saving log.\n\n2013-06-07 09:14:13 Experiment started\n\n2013-06-07 09:02:14 Experiment ended\n\n2013-06-07 09:01:44 Saving log.\n\n2013-06-07 08:39:32 Experiment started\n\n2013-06-07 08:36:55 Experiment ended\n\n2013-06-07 08:36:28 Saving log.\n\n2013-06-07 08:16:57 Experiment started\n\n2013-06-07 08:14:30 Experiment ended\n\n2013-06-07 08:14:13 Saving log.\n\n2013-06-07 08:02:58 Experiment started\n\n2013-06-07 08:02:18 Experiment ended\n\n2013-06-07 08:00:56 Experiment started\n\n2013-06-07 08:00:50 Experiment ended\n\n2013-06-07 07:58:54 Experiment started\n\n2013-06-07 07:57:13 Experiment ended\n\n2013-06-07 07:57:00 Saving log.\n\n2013-06-07 07:47:56 Experiment started\n\n2013-06-07 07:47:30 Experiment ended\n\n2013-06-07 07:47:20 Saving log.\n\n2013-06-07 07:41:56 Experiment started\n\n2013-06-07 07:40:08 Experiment ended\n\n2013-06-07 07:39:57 Saving log.\n\n2013-06-07 07:31:04 Experiment started\n\n2013-06-07 07:29:26 Experiment ended\n\n2013-06-07 07:28:56 Saving log.\n\n2013-06-07 07:08:55 Experiment started\n\n2013-06-07 07:05:22 Experiment ended\n\n2013-06-07 07:04:48 Experiment started\n\n2013-06-06 18:29:00 Experiment ended\n\n2013-06-06 18:28:27 Saving log.\n\n2013-06-06 18:09:12 Experiment started\n\n2013-06-06 18:08:54 Experiment ended\n\n2013-06-06 18:08:30 Experiment started\n\n2013-06-06 18:07:55 Experiment ended\n\n2013-06-06 18:06:54 Experiment started\n\n2013-06-06 18:06:30 Experiment ended\n\n2013-06-06 18:06:02 Saving log.\n\n2013-06-06 17:47:44 Experiment started\n\n2013-06-06 17:44:41 Experiment ended\n\n2013-06-06 17:44:10 Saving log.\n\n2013-06-06 17:02:31 Experiment started\n\n2013-06-06 17:02:30 Experiment ended\n\n2013-06-06 17:02:10 Experiment started\n\n2013-06-06 16:43:26 Experiment ended\n\n2013-06-06 16:42:51 Experiment started\n\n2013-06-06 16:39:49 Experiment ended\n\n2013-06-06 16:39:17 Saving log.\n\n2013-06-06 16:09:29 Experiment started\n\n2013-06-06 16:09:03 Experiment ended\n\n2013-06-06 16:08:54 Saving log.\n\n2013-06-06 16:07:11 Experiment started\n\n2013-06-06 14:52:12 Experiment ended\n\n2013-06-06 14:51:40 Saving log.\n\n2013-06-06 14:31:02 Experiment started\n\n2013-06-06 14:27:57 Experiment ended\n\n2013-06-06 14:27:29 Saving log.\n\n2013-06-06 14:06:37 Experiment started\n\n2013-06-06 14:05:04 Experiment ended\n\n2013-06-06 14:04:33 Saving log.\n\n2013-06-06 13:43:19 Experiment started\n\n2013-06-06 13:37:37 Experiment ended\n\n2013-06-06 13:35:47 Saving log.\n\n2013-06-06 12:04:00 Experiment started\n\n2013-06-06 12:03:53 Experiment ended\n\n2013-06-06 12:03:37 Saving log.\n\n2013-06-06 11:49:26 Experiment started\n\n2013-06-06 11:49:03 Experiment ended\n\n2013-06-06 11:48:54 Saving log.\n\n2013-06-06 11:44:51 Experiment started\n\n2013-06-06 11:44:43 Experiment ended\n\n2013-06-06 11:44:35 Saving log.\n\n2013-06-06 11:44:11 Experiment started\n\n2013-06-06 11:42:13 Experiment ended\n\n2013-06-06 11:41:44 Experiment started\n\n2013-06-06 11:40:21 Experiment ended\n\n2013-06-06 11:40:12 Saving log.\n\n2013-06-06 11:38:30 Experiment started\n\n2013-06-06 11:35:16 Experiment ended\n\n2013-06-06 11:33:21 Experiment started\n\n2013-06-06 11:31:51 Experiment ended\n\n2013-06-06 11:31:26 Experiment started\n\n2013-06-06 10:55:13 Experiment ended\n\n2013-06-06 10:55:05 Saving log.\n\n2013-06-06 10:53:12 Experiment started\n\n2013-06-06 10:52:49 Experiment ended\n\n2013-06-06 10:52:41 Saving log.\n\n2013-06-06 10:50:52 Experiment started\n\n2013-06-06 10:50:43 Experiment ended\n\n2013-06-06 10:50:34 Saving log.\n\n2013-06-06 10:48:00 Experiment started\n\n2013-06-06 10:47:33 Experiment ended\n\n2013-06-06 10:47:25 Saving log.\n\n2013-06-06 10:45:17 Experiment started\n\n2013-06-06 10:41:43 Experiment ended\n\n2013-06-06 10:41:18 Saving log.\n\n2013-06-06 10:27:19 Experiment started\n\n2013-06-06 10:25:29 Experiment ended\n\n2013-06-06 10:25:21 Saving log.\n\n2013-06-06 10:24:46 Experiment started\n\n2013-06-06 10:24:11 Experiment ended\n\n2013-06-06 10:23:59 Saving log.\n\n2013-06-06 10:16:33 Experiment started\n\n2013-06-06 10:16:07 Experiment ended\n\n2013-06-06 10:15:55 Saving log.\n\n2013-06-06 10:04:04 Experiment started\n\n2013-06-06 10:03:55 Experiment ended\n\n2013-06-06 10:03:37 Saving log.\n\n2013-06-06 09:50:59 Experiment started\n\n2013-06-06 09:49:33 Experiment ended\n\n2013-06-06 09:49:14 Saving log.\n\n2013-06-06 09:39:21 Experiment started\n\n2013-06-06 09:37:22 Experiment ended\n\n2013-06-06 09:37:04 Saving log.\n\n2013-06-06 09:27:05 Experiment started\n\n2013-06-06 09:27:03 Experiment ended\n\n2013-06-06 09:26:53 Saving log.\n\n2013-06-06 09:23:01 Experiment started\n\n2013-06-06 09:22:31 Experiment ended\n\n2013-06-06 09:21:50 Experiment started\n\n2013-06-06 09:16:03 Experiment ended\n\n2013-06-06 09:15:39 Experiment started\n\n2013-06-06 09:15:29 Experiment ended\n\n2013-06-06 09:15:11 Saving log.\n\n2013-06-06 09:05:36 Experiment started\n\n2013-06-06 09:05:21 Experiment ended\n\n2013-06-06 09:05:09 Saving log.\n\n2013-06-06 08:59:46 Experiment started\n\n2013-06-06 08:59:31 Experiment ended\n\n2013-06-06 08:59:20 Saving log.\n\n2013-06-06 08:53:30 Experiment started\n\n2013-06-06 08:53:29 Experiment ended\n\n2013-06-06 08:53:12 Saving log.\n\n2013-06-06 08:43:19 Experiment started\n\n2013-06-06 08:42:49 Experiment ended\n\n2013-06-06 08:42:16 Experiment started\n\n2013-06-06 08:42:15 Experiment ended\n\n2013-06-06 08:41:56 Experiment started\n\n2013-06-06 08:41:38 Experiment ended\n\n2013-06-06 08:41:11 Experiment started\n\n2013-06-06 08:38:39 Experiment ended\n\n2013-06-06 08:38:19 Experiment started\n\n2013-06-06 08:37:43 Experiment ended\n\n2013-06-06 08:37:18 Experiment started\n\n2013-06-06 08:20:36 Experiment ended\n\n2013-06-06 08:12:50 Experiment started\n\n2013-06-06 08:04:51 Experiment ended\n\n2013-06-06 08:04:42 Saving log.\n\n2013-06-06 08:03:14 Experiment started\n\n2013-06-06 07:54:32 Experiment ended\n\n2013-06-06 07:54:25 Saving log.\n\n2013-06-06 07:53:00 Experiment started\n\n2013-06-06 07:48:05 Experiment ended\n\n2013-06-06 07:47:58 Saving log.\n\n2013-06-06 07:46:30 Experiment started\n\n2013-06-06 07:45:50 Error parsing <Variables><IndependentVariables>.  Line may be incomplete:\n\td\t20.000000\t34.000000\t8\n\n2013-06-05 19:36:49 Experiment ended\n\n2013-06-05 19:36:16 Saving log.\n\n2013-06-05 19:15:00 Experiment started\n\n2013-06-05 19:14:55 Experiment ended\n\n2013-06-05 19:14:24 Saving log.\n\n2013-06-05 18:51:37 Experiment started\n\n2013-06-05 18:49:35 Experiment ended\n\n2013-06-05 18:49:06 Saving log.\n\n2013-06-05 18:30:53 Experiment started\n\n2013-06-05 18:17:48 Experiment ended\n\n2013-06-05 18:17:18 Experiment started\n\n2013-06-05 18:10:15 Experiment ended\n\n2013-06-05 18:09:58 Experiment started\n\n2013-06-05 16:33:49 Experiment ended\n\n2013-06-05 16:32:52 Saving log.\n\n2013-06-05 15:50:04 Experiment started\n\n2013-06-05 15:34:59 Experiment ended\n\n2013-06-05 15:34:00 Saving log.\n\n2013-06-05 14:54:03 Experiment started\n\n2013-06-05 14:47:54 Experiment ended\n\n2013-06-05 14:46:08 Saving log.\n\n2013-06-05 13:12:38 Experiment started\n\n2013-06-05 13:12:36 Experiment ended\n\n2013-06-05 13:12:28 Saving log.\n\n2013-06-05 13:11:51 Experiment started\n\n2013-06-05 12:10:10 Experiment ended\n\n2013-06-05 12:09:41 Saving log.\n\n2013-06-05 11:53:31 Experiment started\n\n2013-06-05 11:45:16 Experiment ended\n\n2013-06-05 11:44:57 Experiment started\n\n2013-06-05 11:44:49 Experiment ended\n\n2013-06-05 11:44:30 Experiment started\n\n2013-06-05 11:44:29 Experiment ended\n\n2013-06-05 11:44:08 Experiment started\n\n2013-06-05 11:43:47 Experiment ended\n\n2013-06-05 11:42:00 Experiment started\n\n2013-06-05 11:35:40 Experiment ended\n\n2013-06-05 11:35:09 Saving log.\n\n2013-06-05 11:16:25 Experiment started\n\n2013-06-05 11:16:20 Experiment ended\n\n2013-06-05 11:16:13 Saving log.\n\n2013-06-05 11:15:43 Experiment started\n\n2013-06-05 11:13:39 Experiment ended\n\n2013-06-05 11:13:13 Experiment started\n\n2013-06-05 11:08:07 Experiment ended\n\n2013-06-05 11:07:49 Saving log.\n\n2013-06-05 10:57:49 Experiment started\n\n2013-06-05 10:52:26 Experiment ended\n\n2013-06-05 10:49:19 Experiment started\n\n2013-06-05 10:48:51 Experiment ended\n\n2013-06-05 10:48:24 Experiment started\n\n2013-06-05 10:47:52 Experiment ended\n\n2013-06-05 10:47:18 Experiment started\n\n2013-06-05 10:47:06 Experiment ended\n\n2013-06-05 10:46:08 Experiment started\n\n2013-06-05 10:39:49 Experiment ended\n\n2013-06-05 10:38:16 Experiment started\n\n2013-06-05 10:36:32 Experiment ended\n\n2013-06-05 10:36:14 Saving log.\n\n2013-06-05 10:26:10 Experiment started\n\n2013-06-05 10:23:22 Experiment ended\n\n2013-06-05 10:22:38 Experiment started\n\n2013-06-05 10:17:10 Experiment ended\n\n2013-06-05 10:16:53 Saving log.\n\n2013-06-05 10:06:07 Experiment started\n\n2013-06-05 09:53:52 Experiment ended\n\n2013-06-05 09:53:01 Experiment started\n\n2013-06-05 09:52:49 Experiment ended\n\n2013-06-05 09:42:44 Experiment started\n\n2013-06-05 09:41:04 Experiment ended\n\n2013-06-05 09:40:23 Experiment started\n\n2013-06-05 09:39:38 Experiment ended\n\n2013-06-05 09:39:20 Saving log.\n\n2013-06-05 09:29:12 Experiment started\n\n2013-06-05 09:24:20 Experiment ended\n\n2013-06-05 09:24:13 Saving log.\n\n2013-06-05 09:22:00 Experiment started\n\n2013-06-05 09:10:33 Experiment ended\n\n2013-06-05 09:09:54 Experiment started\n\n2013-06-05 09:02:41 Experiment ended\n\n2013-06-05 09:02:23 Saving log.\n\n2013-06-05 08:52:18 Experiment started\n\n2013-06-05 08:52:12 Experiment ended\n\n2013-06-05 08:51:57 Saving log.\n\n2013-06-05 08:43:05 Experiment started\n\n2013-06-05 08:36:10 Experiment ended\n\n2013-06-05 08:35:52 Saving log.\n\n2013-06-05 08:25:51 Experiment started\n\n2013-06-05 08:16:42 Experiment ended\n\n2013-06-05 08:16:18 Saving log.\n\n2013-06-05 08:05:48 Experiment started\n\n2013-06-05 08:04:56 Experiment ended\n\n2013-06-05 08:04:31 Saving log.\n\n2013-06-05 07:52:59 Experiment started\n\n2013-06-05 07:52:49 Experiment ended\n\n2013-06-05 07:52:41 Saving log.\n\n2013-06-05 07:52:09 Experiment started\n\n2013-06-05 07:50:41 Experiment ended\n\n2013-06-05 07:50:11 Experiment started\n\n2013-06-05 07:50:11 Experiment ended\n\n2013-06-05 07:47:43 Experiment started\n\n2013-06-05 07:47:29 Experiment ended\n\n2013-06-05 07:47:17 Saving log.\n\n2013-06-05 07:44:34 Experiment started\n\n2013-06-05 07:42:27 Experiment ended\n\n2013-06-05 07:42:17 Saving log.\n\n2013-06-05 07:39:21 Experiment started\n\n2013-06-05 07:38:12 Experiment ended\n\n2013-06-05 07:38:03 Saving log.\n\n2013-06-05 07:34:57 Experiment started\n\n2013-06-05 07:33:36 Experiment ended\n\n2013-06-05 07:33:29 Saving log.\n\n2013-06-05 07:30:50 Experiment started\n\n2013-06-05 07:30:46 Experiment ended\n\n2013-06-05 07:30:39 Saving log.\n\n2013-06-05 07:30:26 Experiment started\n\n2013-06-05 07:26:18 Experiment ended\n\n2013-06-05 07:25:18 Experiment started\n\n2013-06-05 07:24:54 Experiment ended\n\n2013-06-05 07:23:35 Experiment started\n\n2013-06-05 07:23:17 Experiment ended\n\n2013-06-05 07:22:42 Experiment started\n\n2013-06-05 07:22:40 Experiment ended\n\n2013-06-05 07:22:14 Experiment started\n\n2013-06-05 07:21:37 Experiment ended\n\n2013-06-05 07:21:09 Experiment started\n\n2013-06-05 07:21:08 Experiment ended\n\n2013-06-05 07:20:41 Experiment started\n\n2013-06-05 07:20:32 Experiment ended\n\n2013-06-05 07:19:58 Experiment started\n\n2013-06-05 07:19:53 Experiment ended\n\n2013-06-05 07:19:33 Experiment started\n\n2013-06-05 07:17:06 Experiment ended\n\n2013-06-05 07:16:47 Experiment started\n\n2013-06-04 17:03:18 Experiment ended\n\n2013-06-04 17:01:28 Saving log.\n\n2013-06-04 15:53:14 Experiment started\n\n2013-06-04 15:47:59 Experiment ended\n\n2013-06-04 15:47:06 Experiment started\n\n2013-06-04 15:46:36 Experiment ended\n\n2013-06-04 15:45:31 Experiment started\n\n2013-06-04 15:45:29 Experiment ended\n\n2013-06-04 15:40:17 Experiment started\n\n2013-06-04 15:35:43 Experiment started\n\n2013-06-04 15:35:42 Experiment ended\n\n2013-06-04 15:34:03 Experiment started\n\n2013-06-04 15:33:16 Experiment ended\n\n2013-06-04 15:32:40 Experiment started\n\n2013-06-04 15:32:24 Experiment ended\n\n2013-06-04 15:30:10 Experiment started\n\n2013-06-04 15:25:13 Experiment ended\n\n2013-06-04 15:23:32 Experiment started\n\n2013-06-04 15:05:09 Experiment ended\n\n2013-06-04 15:04:30 Experiment started\n\n2013-06-04 14:54:43 Experiment ended\n\n2013-06-04 14:52:41 Saving log.\n\n2013-06-04 13:45:30 Experiment started\n\n2013-06-04 13:45:10 Experiment ended\n\n2013-06-04 13:45:03 Saving log.\n\n2013-06-04 13:43:58 Experiment started\n\n2013-06-04 13:22:06 Experiment ended\n\n2013-06-04 13:21:49 Experiment started\n\n2013-06-04 12:55:49 Experiment ended\n\n2013-06-04 12:55:30 Experiment started\n\n2013-06-04 12:11:43 Experiment ended\n\n2013-06-04 12:11:21 Experiment started\n\n2013-06-04 12:11:19 Experiment ended\n\n2013-06-04 12:11:00 Experiment started\n\n2013-06-04 12:10:51 Experiment ended\n\n2013-06-04 12:10:29 Experiment started\n\n2013-06-04 12:10:22 Experiment ended\n\n2013-06-04 12:07:22 Experiment started\n\n2013-06-04 12:06:36 Experiment ended\n\n2013-06-04 12:04:35 Experiment started\n\n2013-06-04 12:00:30 Experiment ended\n\n2013-06-04 12:00:07 Experiment started\n\n2013-06-04 12:00:06 Experiment ended\n\n2013-06-04 11:59:42 Experiment started\n\n2013-06-04 11:59:41 Experiment ended\n\n2013-06-04 11:59:21 Experiment started\n\n2013-06-04 11:59:21 Experiment ended\n\n2013-06-04 11:58:57 Experiment started\n\n2013-06-04 11:58:55 Experiment ended\n\n2013-06-04 11:58:37 Experiment started\n\n2013-06-04 11:58:35 Experiment ended\n\n2013-06-04 11:58:16 Experiment started\n\n2013-06-04 11:58:15 Experiment ended\n\n2013-06-04 11:57:05 Experiment started\n\n2013-06-04 11:57:02 Experiment ended\n\n2013-06-04 11:56:45 Experiment started\n\n2013-06-04 11:56:29 Experiment ended\n\n2013-06-04 11:56:07 Experiment started\n\n2013-06-04 11:50:40 Experiment ended\n\n2013-06-04 11:50:08 Saving log.\n\n2013-06-04 11:31:23 Experiment started\n\n2013-06-04 11:30:27 Experiment ended\n\n2013-06-04 11:30:12 Saving log.\n\n2013-06-04 11:21:38 Experiment started\n\n2013-06-04 11:20:53 Experiment ended\n\n2013-06-04 11:20:39 Saving log.\n\n2013-06-04 11:12:04 Experiment started\n\n2013-06-04 11:08:57 Experiment ended\n\n2013-06-04 11:08:24 Saving log.\n\n2013-06-04 10:54:02 Experiment started\n\n2013-06-04 10:51:59 Experiment ended\n\n2013-06-04 10:51:36 Saving log.\n\n2013-06-04 10:38:04 Experiment started\n\n2013-06-04 10:37:59 Experiment ended\n\n2013-06-04 10:37:48 Saving log.\n\n2013-06-04 10:33:17 Experiment started\n\n2013-06-04 10:24:45 Experiment ended\n\n2013-06-04 10:24:12 Saving log.\n\n2013-06-04 10:05:49 Experiment started\n\n2013-06-04 09:52:07 Experiment ended\n\n2013-06-04 09:51:48 Saving log.\n\n2013-06-04 09:41:34 Experiment started\n\n2013-06-04 09:21:53 Experiment ended\n\n2013-06-04 09:21:35 Saving log.\n\n2013-06-04 09:13:43 Experiment started\n\n2013-06-04 09:13:21 Experiment ended\n\n2013-06-04 09:13:03 Saving log.\n\n2013-06-04 09:05:14 Experiment started\n\n2013-06-04 09:04:51 Experiment ended\n\n2013-06-04 09:02:06 Experiment started\n\n2013-06-04 08:54:32 Experiment ended\n\n2013-06-04 08:54:13 Experiment started\n\n2013-06-04 08:46:19 Experiment ended\n\n2013-06-04 08:45:03 Experiment started\n\n2013-06-04 08:44:57 Experiment ended\n\n2013-06-04 08:43:28 Experiment started\n\n2013-06-04 08:41:55 Experiment ended\n\n2013-06-04 08:41:37 Saving log.\n\n2013-06-04 08:33:22 Experiment started\n\n2013-06-04 08:27:57 Experiment ended\n\n2013-06-04 08:27:39 Saving log.\n\n2013-06-04 08:19:45 Experiment started\n\n2013-06-04 08:19:44 Experiment ended\n\n2013-06-04 08:18:49 Experiment started\n\n2013-06-04 08:18:29 Experiment ended\n\n2013-06-04 08:17:40 Experiment started\n\n2013-06-04 08:17:15 Experiment ended\n\n2013-06-04 08:16:43 Saving log.\n\n2013-06-04 08:01:51 Experiment started\n\n2013-06-04 08:01:11 Experiment ended\n\n2013-06-04 08:00:58 Saving log.\n\n2013-06-04 07:55:22 Experiment started\n\n2013-06-04 07:54:37 Error cleared and continued by user\n\n2013-06-04 07:54:34 Error -7 occurred at Data Receive (DLL) Timeout Error\nGCS Error: Timeout error\r\n\r\nThis error code is undefined. Undefined errors might occur for a number of reasons. For example, no one has provided a description for the code, or you might have wired a number that is not an error code to the error code input. \n\nAdditionally, undefined error codes might occur because the error relates to a third-party object, such as the operating system or ActiveX. For these third-party errors, you might be able to obtain a description of the error by searching the Web for the error code (-7) or for its hexadecimal representation (0xFFFFFFF9).\nCall chain:\nhandle_errors.vi cesium_controller.vi\r\n\n\n2013-06-04 07:54:34 Experiment ended\n\n2013-06-04 07:54:28 Saving log.\n\n2013-06-04 07:47:31 Experiment started\n\n2013-06-04 07:37:31 Experiment ended\n\n2013-06-04 07:37:22 Saving log.\n\n2013-06-04 07:36:00 Experiment started\n\n2013-06-04 07:34:45 Experiment ended\n\n2013-06-04 07:34:36 Saving log.\n\n2013-06-04 07:32:37 Experiment started\n\n2013-06-03 17:45:39 Experiment ended\n\n2013-06-03 17:45:05 Saving log.\n\n2013-06-03 15:56:07 Experiment started\n\n2013-06-03 15:55:36 Experiment ended\n\n2013-06-03 15:55:13 Saving log.\n\n2013-06-03 15:42:27 Experiment started\n\n2013-06-03 15:41:47 Experiment ended\n\n2013-06-03 15:41:28 Saving log.\n\n2013-06-03 15:30:19 Experiment started\n\n2013-06-03 15:29:54 Experiment ended\n\n2013-06-03 15:29:42 Saving log.\n\n2013-06-03 15:23:27 Experiment started\n\n2013-06-03 15:23:26 Experiment ended\n\n2013-06-03 15:23:17 Saving log.\n\n2013-06-03 15:22:25 Experiment started\n\n2013-06-03 15:22:25 Experiment ended\n\n2013-06-03 15:22:17 Saving log.\n\n2013-06-03 15:20:15 Experiment started\n\n2013-06-03 15:18:39 Experiment ended\n\n2013-06-03 15:18:13 Saving log.\n\n2013-06-03 15:02:15 Experiment started\n\n2013-06-03 15:02:09 Experiment ended\n\n2013-06-03 15:01:43 Saving log.\n\n2013-06-03 14:46:04 Experiment started\n\n2013-06-03 14:45:32 Experiment ended\n\n2013-06-03 14:45:08 Saving log.\n\n2013-06-03 14:30:18 Experiment started\n\n2013-06-03 14:30:07 Experiment ended\n\n2013-06-03 14:29:59 Saving log.\n\n2013-06-03 14:29:46 Experiment started\n\n2013-06-03 14:23:22 Experiment ended\n\n2013-06-03 14:23:00 Experiment started\n\n2013-06-03 14:22:21 Experiment ended\n\n2013-06-03 14:20:35 Experiment started\n\n2013-06-03 14:04:57 Experiment ended\n\n2013-06-03 13:52:56 Experiment started\n\n2013-06-03 13:43:36 Experiment ended\n\n2013-06-03 13:43:06 Saving log.\n\n2013-06-03 13:24:29 Experiment started\n\n2013-06-03 13:21:21 Experiment ended\n\n2013-06-03 13:21:02 Saving log.\n\n2013-06-03 13:07:51 Experiment started\n\n2013-06-03 13:04:58 Experiment ended\n\n2013-06-03 13:04:40 Experiment started\n\n2013-06-03 13:03:55 Experiment ended\n\n2013-06-03 13:03:48 Saving log.\n\n2013-06-03 13:03:34 Experiment started\n\n2013-06-03 12:52:41 Experiment ended\n\n2013-06-03 12:52:09 Saving log.\n\n2013-06-03 12:30:30 Experiment started\n\n2013-06-03 12:23:48 Experiment ended\n\n2013-06-03 12:23:38 Saving log.\n\n2013-06-03 12:14:12 Experiment started\n\n2013-06-03 12:14:12 Experiment ended\n\n2013-06-03 12:13:59 Saving log.\n\n2013-06-03 12:03:35 Experiment started\n\n2013-06-03 11:45:06 Experiment ended\n\n2013-06-03 11:44:48 Experiment started\n\n2013-06-03 11:40:26 Experiment ended\n\n2013-06-03 11:40:11 Experiment started\n\n2013-06-03 10:45:48 Experiment ended\n\n2013-06-03 10:45:40 Saving log.\n\n2013-06-03 10:43:05 Experiment started\n\n2013-06-03 10:05:04 Experiment ended\n\n2013-06-03 10:04:57 Saving log.\n\n2013-06-03 10:02:03 Experiment started\n\n2013-06-03 09:58:34 Experiment ended\n\n2013-06-03 09:58:26 Saving log.\n\n2013-06-03 09:56:30 Experiment started\n\n2013-06-03 09:56:28 Experiment ended\n\n2013-06-03 09:56:21 Saving log.\n\n2013-06-03 09:54:26 Experiment started\n\n2013-06-03 09:45:56 Experiment ended\n\n2013-06-03 09:45:34 Saving log.\n\n2013-06-03 09:33:06 Experiment started\n\n2013-06-03 09:27:26 Experiment ended\n\n2013-06-03 09:27:06 Saving log.\n\n2013-06-03 09:15:58 Experiment started\n\n2013-06-03 09:15:28 Experiment ended\n\n2013-06-03 09:15:16 Saving log.\n\n2013-06-03 09:08:07 Experiment started\n\n2013-06-03 09:06:43 Experiment ended\n\n2013-06-03 09:06:26 Saving log.\n\n2013-06-03 08:56:05 Experiment started\n\n2013-06-03 08:44:17 Experiment ended\n\n2013-06-03 08:43:58 Saving log.\n\n2013-06-03 08:31:52 Experiment started\n\n2013-06-03 08:31:36 Experiment ended\n\n2013-06-03 08:31:25 Saving log.\n\n2013-06-03 08:25:37 Experiment started\n\n2013-06-03 08:17:38 Experiment ended\n\n2013-06-03 08:17:20 Saving log.\n\n2013-06-03 08:05:29 Experiment started\n\n2013-06-03 08:03:15 Experiment ended\n\n2013-06-03 08:03:07 Saving log.\n\n2013-06-03 08:01:12 Experiment started\n\n2013-06-03 07:53:59 Experiment ended\n\n2013-06-03 07:53:51 Saving log.\n\n2013-06-03 07:52:08 Experiment started\n\n2013-06-03 07:46:58 Experiment ended\n\n2013-06-03 07:46:51 Saving log.\n\n2013-06-03 07:45:05 Experiment started\n\n2013-06-03 07:45:01 Experiment ended\n\n2013-06-03 07:44:36 Experiment started\n\n2013-06-03 07:44:18 Experiment ended\n\n2013-06-03 07:43:55 Experiment started\n\n2013-06-03 07:43:28 Experiment ended\n\n2013-06-03 07:26:21 Experiment started\n\n2013-06-03 07:25:05 Experiment ended\n\n2013-06-03 07:22:39 Experiment started\n\n2013-06-03 07:19:59 Experiment ended\n\n2013-06-03 07:18:03 Experiment started\n\n2013-06-02 16:42:12 Experiment ended\n\n2013-06-02 16:40:28 Experiment started\n\n2013-06-02 16:37:53 Experiment ended\n\n2013-06-02 16:37:35 Saving log.\n\n2013-06-02 16:27:19 Experiment started\n\n2013-06-02 16:27:13 Experiment ended\n\n2013-06-02 16:26:56 Saving log.\n\n2013-06-02 16:16:37 Experiment started\n\n2013-06-02 16:11:11 Experiment ended\n\n2013-06-02 16:10:52 Saving log.\n\n2013-06-02 16:00:40 Experiment started\n\n2013-06-02 15:55:28 Experiment ended\n\n2013-06-02 15:55:10 Saving log.\n\n2013-06-02 15:44:46 Experiment started\n\n2013-06-02 15:39:21 Experiment ended\n\n2013-06-02 15:39:03 Saving log.\n\n2013-06-02 15:28:39 Experiment started\n\n2013-06-02 15:21:29 Experiment ended\n\n2013-06-02 15:21:11 Saving log.\n\n2013-06-02 15:09:48 Experiment started\n\n2013-06-02 15:09:46 Experiment ended\n\n2013-06-02 15:09:35 Saving log.\n\n2013-06-02 15:05:12 Experiment started\n\n2013-06-02 15:01:42 Experiment ended\n\n2013-06-02 15:01:23 Saving log.\n\n2013-06-02 14:51:03 Experiment started\n\n2013-06-02 14:50:29 Experiment ended\n\n2013-06-02 14:50:15 Saving log.\n\n2013-06-02 14:41:39 Experiment started\n\n2013-06-02 14:31:24 Experiment ended\n\n2013-06-02 14:30:51 Saving log.\n\n2013-06-02 14:12:06 Experiment started\n\n2013-06-02 14:08:35 Experiment ended\n\n2013-06-02 14:08:02 Saving log.\n\n2013-06-02 13:49:08 Experiment started\n\n2013-06-02 13:48:46 Experiment ended\n\n2013-06-02 13:48:24 Experiment started\n\n2013-06-02 13:47:53 Experiment ended\n\n2013-06-02 13:47:31 Experiment started\n\n2013-06-02 13:45:47 Experiment ended\n\n2013-06-02 13:45:12 Saving log.\n\n2013-06-02 13:27:00 Experiment started\n\n2013-06-02 13:26:34 Experiment ended\n\n2013-06-02 13:22:56 Experiment started\n\n2013-06-02 13:21:43 Experiment ended\n\n2013-06-02 13:21:36 Saving log.\n\n2013-06-02 13:21:06 Experiment started\n\n2013-06-02 13:20:36 Experiment ended\n\n2013-06-02 13:20:21 Saving log.\n\n2013-06-02 13:11:27 Experiment started\n\n2013-06-02 13:10:58 Experiment ended\n\n2013-06-02 13:10:38 Saving log.\n\n2013-06-02 12:58:09 Experiment started\n\n2013-06-02 12:56:35 Experiment ended\n\n2013-06-02 12:56:27 Saving log.\n\n2013-06-02 12:54:39 Experiment started\n\n2013-06-02 12:50:05 Experiment ended\n\n2013-06-02 12:49:58 Saving log.\n\n2013-06-02 12:49:03 Experiment started\n\n2013-06-02 12:48:54 Experiment ended\n\n2013-06-02 12:48:46 Saving log.\n\n2013-06-02 12:48:26 Experiment started\n\n2013-06-02 12:33:23 Experiment ended\n\n2013-06-02 12:33:14 Saving log.\n\n2013-06-02 12:31:32 Experiment started\n\n2013-06-02 12:26:35 Experiment ended\n\n2013-06-02 12:26:28 Saving log.\n\n2013-06-02 12:24:35 Experiment started\n\n2013-06-02 12:24:05 Experiment ended\n\n2013-06-02 12:23:25 Experiment started\n\n2013-06-02 11:55:01 Experiment ended\n\n2013-05-31 18:01:01 Experiment started\n\n2013-05-31 18:01:00 Experiment ended\n\n2013-05-31 17:52:35 Experiment started\n\n2013-05-31 17:52:19 Experiment ended\n\n2013-05-31 17:44:01 Experiment started\n\n2013-05-31 17:42:22 Experiment ended\n\n2013-05-31 17:34:12 Experiment started\n\n2013-05-31 17:34:12 Experiment ended\n\n2013-05-31 17:33:06 Experiment started\n\n2013-05-31 17:30:49 Experiment ended\n\n2013-05-31 17:29:29 Experiment started\n\n2013-05-31 17:29:27 Experiment ended\n\n2013-05-31 17:28:49 Experiment started\n\n2013-05-31 17:28:21 Experiment ended\n\n2013-05-31 17:27:56 Experiment started\n\n2013-05-31 17:27:36 Experiment ended\n\n2013-05-31 17:27:12 Experiment started\n\n2013-05-31 17:26:38 Experiment ended\n\n2013-05-31 17:25:38 Experiment started\n\n2013-05-31 17:23:11 Experiment ended\n\n2013-05-31 17:22:04 Experiment started\n\n2013-05-31 17:21:59 Halted by user.\n\n2013-05-31 17:21:57 Error -1074397163 occurred at IMAQ Serial Write.vi\r\n\r\nPossible reason(s):\n\r\nNI-IMAQ:  The passed in interface or session is invalid.\nCall chain:\nhandle_errors.vi Hamamatsu_serial.vi Hamamatsu_C9100-13.lvclass:initialize.vi run_experiment.vi cesium_controller.vi\r\n\n\n2013-05-31 17:21:56 Experiment started\n\n2013-05-31 17:19:42 Experiment ended\n\n2013-05-31 17:19:30 Experiment started\n\n2013-05-31 17:19:22 Experiment ended\n\n2013-05-31 17:19:08 Experiment started\n\n2013-05-31 17:09:26 Experiment ended\n\n2013-05-31 17:09:25 Saving log.\n\n2013-05-31 17:09:09 Experiment started\n\n"
  in  "Variable Actions":T2
  in  "Variable Settings":T3={"Measurements per Iteration"=100, "Local Data Path"=path "C:/Users/QC/Documents/Cesium_project/LabVIEW Projects/data", "Experiment description suffix for filename (no spaces please)"="_blue_align_ROI32_roughscan_axis2", "Network Data Path"=path "Z:/", "Copy data to network"=TRUE, "Measurement Timeout (ms)"=60000, "Independent Variables"=[{"Description"="raman frequency", "Name (a,a0...a9)"="a", "min"=9172.612, "max"=9172.612, "# steps"=1}, {"Description"="microwave frequency", "Name (a,a0...a9)"="b", "min"=9192.6319, "max"=9192.6319, "# steps"=1}, {"Description"="459 single site OP time", "Name (a,a0...a9)"="k6", "min"=0.1, "max"=0.1, "# steps"=1}, {"Description"="piezo axis 1", "Name (a,a0...a9)"="d", "min"=0.0, "max"=100.0, "# steps"=11}], "Dependent Variables"=[{"Description"="MOT loading time", "Name (a,a0...a9)"="d0", "Equation"="200", "Result"=200.0}, {"Description"="MOT frequency", "Name (a,a0...a9)"="d1", "Equation"="108", "Result"=108.0}, {"Description"="MOT power", "Name (a,a0...a9)"="d2", "Equation"="0", "Result"=0.0}, {"Description"="Hyperfine time", "Name (a,a0...a9)"="d3", "Equation"="d0", "Result"=200.0}, {"Description"="hyperfine frequency", "Name (a,a0...a9)"="d4", "Equation"="278.5", "Result"=278.5}, {"Description"="hyperfine power", "Name (a,a0...a9)"="d5", "Equation"="0", "Result"=0.0}, {"Description"="Trap drop time before loading", "Name (a,a0...a9)"="d6", "Equation"="10", "Result"=10.0}, {"Description"="2D Mot Time", "Name (a,a0...a9)"="d7", "Equation"="d0-12.5", "Result"=187.5}, {"Description"="Trap Off Time", "Name (a,a0...a9)"="d8", "Equation"="d0-50", "Result"=150.0}, {"Description"="trap on time during loading", "Name (a,a0...a9)"="d9", "Equation"="d0-d8-d6-10", "Result"=30.0}, {"Description"="MOT Gradient field setting", "Name (a,a0...a9)"="e0", "Equation"="4.5", "Result"=4.5}, {"Description"="MOT x2/5 shim setting", "Name (a,a0...a9)"="e1", "Equation"=".35", "Result"=0.35}, {"Description"="MOT x3/6 shim setting", "Name (a,a0...a9)"="e2", "Equation"=".55", "Result"=0.55}, {"Description"="MOT vertical shim setting", "Name (a,a0...a9)"="e3", "Equation"="-1.6", "Result"=-1.6}, {"Description"="MOT bias field setting", "Name (a,a0...a9)"="e4", "Equation"="1.3", "Result"=1.3}, {"Description"="PGC 1 time", "Name (a,a0...a9)"="f0", "Equation"="5", "Result"=5.0}, {"Description"="PGC 1 frequency", "Name (a,a0...a9)"="f1", "Equation"="87", "Result"=87.0}, {"Description"="PGC 1 power", "Name (a,a0...a9)"="f2", "Equation"="-2", "Result"=-2.0}, {"Description"="PGC hyperfine time", "Name (a,a0...a9)"="f3", "Equation"="f0", "Result"=5.0}, {"Description"="PGC 1 hyperfine frequency", "Name (a,a0...a9)"="f4", "Equation"="278.5", "Result"=278.5}, {"Description"="PGC 1 hyperfine power", "Name (a,a0...a9)"="f5", "Equation"="0", "Result"=0.0}, {"Description"="MOT to PGC B field delay", "Name (a,a0...a9)"="f6", "Equation"=".6", "Result"=0.6}, {"Description"="780 trap delay for PGC 1", "Name (a,a0...a9)"="f7", "Equation"="4", "Result"=4.0}, {"Description"="PGC 1 gradient field", "Name (a,a0...a9)"="g0", "Equation"="0", "Result"=0.0}, {"Description"="PGC 1 x2/5 shim setting", "Name (a,a0...a9)"="g1", "Equation"="e1", "Result"=0.35}, {"Description"="PGC 1 x3/6 shim setting", "Name (a,a0...a9)"="g2", "Equation"="e2", "Result"=0.55}, {"Description"="PGC 1 vertical shim setting", "Name (a,a0...a9)"="g3", "Equation"="1.6", "Result"=1.6}, {"Description"="PGC 1 bias field setting", "Name (a,a0...a9)"="g4", "Equation"="1.3", "Result"=1.3}, {"Description"="MOT drop time", "Name (a,a0...a9)"="f8", "Equation"="100", "Result"=100.0}, {"Description"="Readout time", "Name (a,a0...a9)"="i0", "Equation"="50", "Result"=50.0}, {"Description"="Readout frequency", "Name (a,a0...a9)"="i1", "Equation"="91", "Result"=91.0}, {"Description"="Readout Power", "Name (a,a0...a9)"="i2", "Equation"="-5", "Result"=-5.0}, {"Description"="Readout hyperfine frequency", "Name (a,a0...a9)"="i4", "Equation"="278.5", "Result"=278.5}, {"Description"="Readout hyperfine power", "Name (a,a0...a9)"="i5", "Equation"="0", "Result"=0.0}, {"Description"="Pre Readout Time", "Name (a,a0...a9)"="i6", "Equation"="0", "Result"=0.0}, {"Description"="Readout gradient field", "Name (a,a0...a9)"="h0", "Equation"="0", "Result"=0.0}, {"Description"="Readout x2/5 shim setting", "Name (a,a0...a9)"="h1", "Equation"="0", "Result"=0.0}, {"Description"="Readout x3/6 shim setting", "Name (a,a0...a9)"="h2", "Equation"="-.45", "Result"=-0.45}, {"Description"="Readout vertical shim setting", "Name (a,a0...a9)"="h3", "Equation"="-1.7138", "Result"=-1.7138}, {"Description"="Readout bias field setting", "Name (a,a0...a9)"="h4", "Equation"="1.3", "Result"=1.3}, {"Description"="PGC 2 time", "Name (a,a0...a9)"="j0", "Equation"="10", "Result"=10.0}, {"Description"="PGC 2 frequency", "Name (a,a0...a9)"="j1", "Equation"="81", "Result"=81.0}, {"Description"="PGC 2 power", "Name (a,a0...a9)"="j2", "Equation"="-6", "Result"=-6.0}, {"Description"="PGC 2 hyperfine frequency", "Name (a,a0...a9)"="j4", "Equation"="278.5", "Result"=278.5}, {"Description"="PGC 2 hyperfine power", "Name (a,a0...a9)"="j5", "Equation"="0", "Result"=0.0}, {"Description"="Readout to PGC 2 B field delay", "Name (a,a0...a9)"="j6", "Equation"=".001", "Result"=0.001}, {"Description"="Optical Pumping time", "Name (a,a0...a9)"="k0", "Equation"="0", "Result"=0.0}, {"Description"="Optical pumping frequency", "Name (a,a0...a9)"="k1", "Equation"="81", "Result"=81.0}, {"Description"="OP hyperfine time", "Name (a,a0...a9)"="k2", "Equation"="k0", "Result"=0.0}, {"Description"="2nd OP time", "Name (a,a0...a9)"="o4", "Equation"="0", "Result"=0.0}, {"Description"="OP hyperfine frequency", "Name (a,a0...a9)"="k3", "Equation"="278.5", "Result"=278.5}, {"Description"="OP hyperfine Power", "Name (a,a0...a9)"="k4", "Equation"="0", "Result"=0.0}, {"Description"="894 Depumping time", "Name (a,a0...a9)"="k5", "Equation"="10", "Result"=10.0}, {"Description"="459 single site OP time", "Name (a,a0...a9)"="k6", "Equation"="0", "Result"=0.0}, {"Description"="PGC to bias B field delay", "Name (a,a0...a9)"="k7", "Equation"=".1", "Result"=0.1}, {"Description"="delay before excitation pulse", "Name (a,a0...a9)"="k8", "Equation"=".5", "Result"=0.5}, {"Description"="delay before blowaway", "Name (a,a0...a9)"="k9", "Equation"=".5", "Result"=0.5}, {"Description"="459 Raman pulse time", "Name (a,a0...a9)"="l0", "Equation"="0", "Result"=0.0}, {"Description"="Rydberg A 459 time", "Name (a,a0...a9)"="l1", "Equation"="0", "Result"=0.0}, {"Description"="Rydberg B 459 time", "Name (a,a0...a9)"="l2", "Equation"="0", "Result"=0.0}, {"Description"="Rydberg A 1038 time", "Name (a,a0...a9)"="l3", "Equation"="l1", "Result"=0.0}, {"Description"="Rydberg B 1038 time", "Name (a,a0...a9)"="l4", "Equation"="l2", "Result"=0.0}, {"Description"="Rydberg B Frequency", "Name (a,a0...a9)"="f", "Equation"="756.2", "Result"=756.2}, {"Description"="Microwave Raman time", "Name (a,a0...a9)"="l5", "Equation"="0", "Result"=0.0}, {"Description"="459 scanner 1 frequency 1", "Name (a,a0...a9)"="m0", "Equation"="150", "Result"=150.0}, {"Description"="459 scanner 2 frequency 2", "Name (a,a0...a9)"="m1", "Equation"="150", "Result"=150.0}, {"Description"="1038 scanner frequency 1", "Name (a,a0...a9)"="m2", "Equation"="144", "Result"=144.0}, {"Description"="1038 scanner frequency 2", "Name (a,a0...a9)"="m3", "Equation"="153", "Result"=153.0}, {"Description"="459 scanner delay/extra time", "Name (a,a0...a9)"="m4", "Equation"=".001", "Result"=0.001}, {"Description"="1038 scanner delay/extra time", "Name (a,a0...a9)"="m5", "Equation"=".001", "Result"=0.001}, {"Description"="459 scanner 1 freq 2", "Name (a,a0...a9)"="m6", "Equation"="157.3", "Result"=157.3}, {"Description"="459 scanner 2 freq 2", "Name (a,a0...a9)"="m7", "Equation"="155.7", "Result"=155.7}, {"Description"="Raman pulse at freq 2", "Name (a,a0...a9)"="m8", "Equation"="0", "Result"=0.0}, {"Description"="Ramsey gap time", "Name (a,a0...a9)"="n9", "Equation"="0", "Result"=0.0}, {"Description"="Ramsey Total Time", "Name (a,a0...a9)"="m9", "Equation"="k8+2*m4+2*l0+n9", "Result"=0.502}, {"Description"="Raman waveform total time", "Name (a,a0...a9)"="l6", "Equation"="k8+2*m4+2*l0+2*m4+m4+m8+m4", "Result"=0.506}, {"Description"="Microwave waveform total time", "Name (a,a0...a9)"="l7", "Equation"="k8+l5", "Result"=0.5}, {"Description"="Rydberg A waveform total time", "Name (a,a0...a9)"="l8", "Equation"="k8+(2*m4+l1+l2)+o4", "Result"=0.502}, {"Description"="Rydberg B waveform total time", "Name (a,a0...a9)"="l9", "Equation"="k8+(m5+l4+m5)*step(-((m4+l2+m4)/(m5+l4+m5))+1)+(m4+l2+m4)*step(((m4+l2+m4)/(m5+l4+m5))-1)", "Result"=0.504}, {"Description"="Exp gradient setting", "Name (a,a0...a9)"="n0", "Equation"="0", "Result"=0.0}, {"Description"="Exp x2/5 shim setting", "Name (a,a0...a9)"="n1", "Equation"="-.2-.15", "Result"=-0.35}, {"Description"="Exp x3/6 shim setting", "Name (a,a0...a9)"="n2", "Equation"="-.2-.13", "Result"=-0.33}, {"Description"="Exp vertical shim setting", "Name (a,a0...a9)"="n3", "Equation"="-1.75", "Result"=-1.75}, {"Description"="Exp bias shim setting", "Name (a,a0...a9)"="n4", "Equation"="-5.65", "Result"=-5.65}, {"Description"="Raman X pi/2 time", "Name (a,a0...a9)"="q1", "Equation"="0", "Result"=0.0}, {"Description"="Raman X 3pi/2 time", "Name (a,a0...a9)"="q2", "Equation"="0", "Result"=0.0}, {"Description"="Raman Z pi/2 time", "Name (a,a0...a9)"="q3", "Equation"="0", "Result"=0.0}, {"Description"="Raman Z 3pi/2 time", "Name (a,a0...a9)"="q4", "Equation"="0", "Result"=0.0}, {"Description"="Raman X pi time", "Name (a,a0...a9)"="q5", "Equation"="0", "Result"=0.0}, {"Description"="Raman Z pi time", "Name (a,a0...a9)"="q6", "Equation"="0", "Result"=0.0}, {"Description"="Random Benchmark total time", "Name (a,a0...a9)"="q7", "Equation"="0", "Result"=0.0}, {"Description"="Blowaway time", "Name (a,a0...a9)"="o0", "Equation"="0", "Result"=0.0}, {"Description"="Blowaway frequency", "Name (a,a0...a9)"="o1", "Equation"="220", "Result"=220.0}, {"Description"="trap realease time", "Name (a,a0...a9)"="o3", "Equation"="0", "Result"=0.0}, {"Description"="max of Raman pulses", "Name (a,a0...a9)"="n6", "Equation"="(l6)*step(-((l7)/(l6))+1)+(l7)*step(((l7)/(l6))-1)", "Result"=0.506}, {"Description"="max of Raman or Ramsey", "Name (a,a0...a9)"="n8", "Equation"="(n6)*step(-((m9)/(n6))+1)+(m9)*step(((m9)/(n6))-1)", "Result"=0.506}, {"Description"="max of Raman or randomized Benchmark", "Name (a,a0...a9)"="q8", "Equation"="(n8)*step(-((q7)/(n8))+1)+(q7)*step(((q7)/(n8))-1)", "Result"=0.506}, {"Description"="max of Rydberg pulses", "Name (a,a0...a9)"="n7", "Equation"="(l9)*step(-((l8)/(l9))+1)+(l8)*step(((l8)/(l9))-1)", "Result"=0.504}, {"Description"="Bias field on time", "Name (a,a0...a9)"="n5", "Equation"="k7+k0+k5+o0+k6+((n7)*step(-((q8)/(n7))+1)+(q8)*step(((q8)/(n7))-1))", "Result"=10.706}, {"Description"="delay between camera shots", "Name (a,a0...a9)"="o2", "Equation"="35", "Result"=35.0}, {"Description"="DDS profile delay", "Name (a,a0...a9)"="t1", "Equation"=".00005", "Result"=5e-05}, {"Description"="685 gradient field", "Name (a,a0...a9)"="p0", "Equation"="0", "Result"=0.0}, {"Description"="685 x2/5 shim setting", "Name (a,a0...a9)"="p1", "Equation"="-.45-.1", "Result"=-0.55}, {"Description"="685 x3/6 shim setting", "Name (a,a0...a9)"="p2", "Equation"=".45+.1", "Result"=0.55}, {"Description"="685 vertical shim setting", "Name (a,a0...a9)"="p3", "Equation"="-1.55", "Result"=-1.55}, {"Description"="685 bias shim setting", "Name (a,a0...a9)"="p4", "Equation"="1.65", "Result"=1.65}, {"Description"="685 time", "Name (a,a0...a9)"="p5", "Equation"="0", "Result"=0.0}, {"Description"="685 frequency", "Name (a,a0...a9)"="p6", "Equation"="194", "Result"=194.0}, {"Description"="685 power", "Name (a,a0...a9)"="p7", "Equation"="0", "Result"=0.0}, {"Description"="speed of light", "Name (a,a0...a9)"="c0", "Equation"="299792458", "Result"=299792458.0}, {"Description"="pi", "Name (a,a0...a9)"="c1", "Equation"="3.141592654", "Result"=3.141592654}, {"Description"="epsilon0", "Name (a,a0...a9)"="c2", "Equation"="1/(4*c1*10^(-7)*c0^2)", "Result"=8.854187816464273e-12}, {"Description"="kB (SI)", "Name (a,a0...a9)"="c3", "Equation"="1.38065*10^(-23)", "Result"=1.3806499999999997e-23}, {"Description"="6s1/2 hyperfine splitting", "Name (a,a0...a9)"="c4", "Equation"="9.19263*10^9", "Result"=9192630000.0}, {"Description"="7p1/2 hyperfine splitting", "Name (a,a0...a9)"="c5", "Equation"="377.4*10^6", "Result"=377400000.0}, {"Description"="6p3/2 gamma", "Name (a,a0...a9)"="c6", "Equation"="2*c1*5.1*10^6", "Result"=32044245.070799995}, {"Description"="7p1/2 gamma", "Name (a,a0...a9)"="c7", "Equation"="2*c1*1*10^6", "Result"=6283185.308}, {"Description"="alpha780 (cgs)", "Name (a,a0...a9)"="c8", "Equation"="-247. * 10^(-24)", "Result"=-2.4699999999999998e-22}, {"Description"="alpha 780 (SI)", "Name (a,a0...a9)"="c9", "Equation"="c8*4*c1*c2*10^(-6)", "Result"=-2.748245638452437e-38}, {"Description"="saturation intensity (W/m^2)", "Name (a,a0...a9)"="a0", "Equation"="27", "Result"=27.0}, {"Description"="mot beam waist 1 (mm)", "Name (a,a0...a9)"="a1", "Equation"="2.5", "Result"=2.5}, {"Description"="mot beam waist 2 (mm)", "Name (a,a0...a9)"="a2", "Equation"="2.5", "Result"=2.5}, {"Description"="mot beam waist 3 (mm)", "Name (a,a0...a9)"="a3", "Equation"="1.54", "Result"=1.54}, {"Description"="readout beam power 1 (uW)*", "Name (a,a0...a9)"="a4", "Equation"="1600", "Result"=1600.0}, {"Description"="readout  beam power 2 (uW)*", "Name (a,a0...a9)"="a5", "Equation"="1600", "Result"=1600.0}, {"Description"="readout beam power 3 (uW)*", "Name (a,a0...a9)"="a6", "Equation"="714", "Result"=714.0}, {"Description"="readout detuning (MHz)*", "Name (a,a0...a9)"="a7", "Equation"="10", "Result"=10.0}, {"Description"="numerical aperture of jenoptiq", "Name (a,a0...a9)"="a9", "Equation"=".4", "Result"=0.4}, {"Description"="transmission efficiency", "Name (a,a0...a9)"="b0", "Equation"=".8", "Result"=0.8}, {"Description"="quantum efficiency", "Name (a,a0...a9)"="b1", "Equation"=".7", "Result"=0.7}, {"Description"="conversion factor for camera (electrons/count)", "Name (a,a0...a9)"="b2", "Equation"="5.8", "Result"=5.8}, {"Description"="analog gain*", "Name (a,a0...a9)"="b3", "Equation"="4", "Result"=4.0}, {"Description"="EM sensitivity (as entered on camera page)*", "Name (a,a0...a9)"="b4", "Equation"="175", "Result"=175.0}, {"Description"="EM gain", "Name (a,a0...a9)"="b5", "Equation"="10^(((log(1000)-log(4))/250)*b4+log(4))", "Result"=190.8174102657344}, {"Description"="average background pixel value", "Name (a,a0...a9)"="b6", "Equation"="10914*(i0/.100)", "Result"=5457000.0}, {"Description"="roi area*", "Name (a,a0...a9)"="b7", "Equation"="9", "Result"=9.0}, {"Description"="imaging system mag", "Name (a,a0...a9)"="b8", "Equation"="25.5", "Result"=25.5}, {"Description"="camera pixel size (um)", "Name (a,a0...a9)"="b9", "Equation"="16", "Result"=16.0}, {"Description"="number of array spots (n)", "Name (a,a0...a9)"="z0", "Equation"="64", "Result"=64.0}, {"Description"="array trap spacing (d microns)", "Name (a,a0...a9)"="z1", "Equation"="3.8", "Result"=3.8}, {"Description"="array beam waist (w0 microns)", "Name (a,a0...a9)"="z2", "Equation"="1.73", "Result"=1.73}, {"Description"="780 power out of the fiber (W)*", "Name (a,a0...a9)"="z3", "Equation"="5", "Result"=5.0}, {"Description"="780 transmission to atoms", "Name (a,a0...a9)"="z4", "Equation"=".6", "Result"=0.6}, {"Description"="459 horizontal waist", "Name (a,a0...a9)"="v0", "Equation"="2*10^(-6)", "Result"=2e-06}, {"Description"="459 vertical waist", "Name (a,a0...a9)"="v1", "Equation"="2*10^(-6)", "Result"=2e-06}, {"Description"="459 scanner transmission", "Name (a,a0...a9)"="v2", "Equation"=".10", "Result"=0.1}, {"Description"="Total Raman Power at fiber", "Name (a,a0...a9)"="v3", "Equation"=".77*10^(-3)", "Result"=0.0007700000000000001}, {"Description"="Raman Detuning (Hz)", "Name (a,a0...a9)"="v4", "Equation"="20*10^9", "Result"=20000000000.0}, {"Description"="1038 horizontal waist", "Name (a,a0...a9)"="w0", "Equation"="2.0*10^(-6)", "Result"=2e-06}, {"Description"="1038 vertical waist", "Name (a,a0...a9)"="w1", "Equation"="2.4*10^(-6)", "Result"=2.4e-06}, {"Description"="1038 scanner transmission", "Name (a,a0...a9)"="w2", "Equation"=".3", "Result"=0.3}, {"Description"="Rydberg A 459 Power at fiber", "Name (a,a0...a9)"="w3", "Equation"="22*10^(-6)", "Result"=2.2e-05}, {"Description"="Rydberg B 459 Power at fiber", "Name (a,a0...a9)"="w4", "Equation"="40*10^(-6)", "Result"=3.9999999999999996e-05}, {"Description"="Rydberg 1038 Power at fiber", "Name (a,a0...a9)"="w5", "Equation"="75*10^(-3)", "Result"=0.075}, {"Description"="Rydberg level", "Name (a,a0...a9)"="w6", "Equation"="61", "Result"=61.0}, {"Description"="Rydberg detuning (Hz)", "Name (a,a0...a9)"="w7", "Equation"="3*10^9", "Result"=3000000000.0}, {"Description"="readout detuning", "Name (a,a0...a9)"="x0", "Equation"="a7*2*c1*10^6", "Result"=62831853.08}, {"Description"="readout beam intensity 1", "Name (a,a0...a9)"="x1", "Equation"="2*a4*10^(-6)/(c1*a1^2*10^(-6))", "Result"=162.97466170482073}, {"Description"="readout beam intensity 2", "Name (a,a0...a9)"="x2", "Equation"="2*a5*10^(-6)/(c1*a2^2*10^(-6))", "Result"=162.97466170482073}, {"Description"="readout beam intensity 3", "Name (a,a0...a9)"="x3", "Equation"="2*a6*10^(-6)/(c1*a3^2*10^(-6))", "Result"=191.66238716946435}, {"Description"="total intensity", "Name (a,a0...a9)"="x4", "Equation"="2*x1+2*x2+2*x3", "Result"=1035.2234211582117}, {"Description"="total saturation parameter", "Name (a,a0...a9)"="x5", "Equation"="x4/a0", "Result"=38.34160819104488}, {"Description"="fractional solid angle", "Name (a,a0...a9)"="y0", "Equation"=".5*(1-sqrt(1-a9^2))", "Result"=0.041742430504416006}, {"Description"="scattering rate", "Name (a,a0...a9)"="y1", "Equation"="(c6/2)*x5/(1+(4*x0^2)/(c6^2)+x5)", "Result"=11226434.194877073}, {"Description"="detected scattering rate for single atom", "Name (a,a0...a9)"="y2", "Equation"="y1*y0*b0*b1", "Result"=262426.44354755123}, {"Description"="detected photon number during exposure time", "Name (a,a0...a9)"="y3", "Equation"="y2*i0", "Result"=13121322.177377561}, {"Description"="Expected Output Signal - Dark Signal", "Name (a,a0...a9)"="y4", "Equation"="y3*b3*b5*b1/b2", "Result"=1208719794.4859817}, {"Description"="Expected Output Signal", "Name (a,a0...a9)"="y5", "Equation"="y4+b6*b7", "Result"=1257832794.4859817}, {"Description"="pixel size after mag (um)", "Name (a,a0...a9)"="y6", "Equation"="b9/b8", "Result"=0.6274509803921569}, {"Description"="lattice period (in pixels)", "Name (a,a0...a9)"="y7", "Equation"="z1/y6", "Result"=6.0562499999999995}, {"Description"="array ratio (s=d/w)", "Name (a,a0...a9)"="z5", "Equation"="z1/z2", "Result"=2.1965317919075145}, {"Description"="total power at atoms (W) ", "Name (a,a0...a9)"="z6", "Equation"="z3*z4", "Result"=3.0}, {"Description"="peak intensity in one spot (P0)", "Name (a,a0...a9)"="z7", "Equation"="(2.*z6/z0)/(c1*z2^2 * 10^(-12))", "Result"=9970781458.062038}, {"Description"="trap depth (mK)", "Name (a,a0...a9)"="z8", "Equation"="-(0.001*2*c1*c8/(c3*c0))*z7*2*exp(-z5^2/2)*(1-2*exp(-z5^2/2))", "Result"=0.5499019000745253}, {"Description"="Raman Rabi Freq (Hz)", "Name (a,a0...a9)"="v5", "Equation"="v3/2*v2/(2*c1*v0*v1)*((-1.305*10^9)/(v4-c5)-7.83*10^8/v4)", "Result"=-161849.25770417508}, {"Description"="Raman Stark Shift (Hz)", "Name (a,a0...a9)"="v6", "Equation"="v3/2*v2/(2*c1*v0*v1)*(4.1*10^9/(2*c1*(v4-c5-c4))-4.1*10^9/(2*c1*(v4-c5+c4)+2.46*10^9/(2*c1*(v4-c4))-2.46*10^9/(2*c1*(v4+c4))))", "Result"=61149.01761903057}, {"Description"="Rydberg A flopping to nD3/2 (Hz)", "Name (a,a0...a9)"="w8", "Equation"="1/(2*c1*w6^(3/2))*sqrt(w3*w2*w5*w2/(v0*v1*w0*w1))*(9.692*10^10/(w7)+5.815*10^10/(w7+c5))", "Result"=1454970.4388004513}, {"Description"="Rydberg B flopping to nD3/2 (Hz)", "Name (a,a0...a9)"="w9", "Equation"="1/(2*c1*w6^(3/2))*sqrt(w4*w2*w5*w2/(v0*v1*w0*w1))*(9.692*10^10/(w7)+5.815*10^10/(w7+c5))", "Result"=1961881.7394546943}, {"Description"="Trap modulation time", "Name (a,a0...a9)"="o5", "Equation"="0", "Result"=0.0}], "Run Test Mode"=FALSE} {"Independent Variables"."# steps" min=1 step=1; "Measurements per Iteration" min=1 step=1}
  in  "HSDIO Settings":T4={"Enable HSDIO Pulses"=FALSE, "Resource Name"="PXI1Slot6", "Clock Rate"=20000000.0, "Array of Script Triggers"=[], "Channels Control"=[["Hex 3D MOT b0", "1", "0", "", "", "", "", "", "", "", "", "", "", "", "", "", "", "", "", ""], ["Hex 3D MOT b0", "1", "0", "", "", "", "", "", "", "", "", "", "", "", "", "", "", "", "", ""], ["repumper bit0", "1", "0", "", "", "", "", "", "", "", "", "", "", "", "", "", "", "", "", ""], ["Trap Array beam switch", "1", "0", "", "", "", "", "", "", "", "", "", "", "", "", "", "", "", "", ""], ["2D MOT switch", "1", "0", "", "", "", "", "", "", "", "", "", "", "", "", "", "", "", "", ""], ["Hamamatsu CCD trigger", "1", "0", "", "", "", "", "", "", "", "", "", "", "", "", "", "", "", "", ""], ["Luca CCD trigger", "1", "0", "", "", "", "", "", "", "", "", "", "", "", "", "", "", "", "", ""], ["broken", "", "", "", "", "", "", "", "", "", "", "", "", "", "", "", "", "", "", ""], ["repumper bit1", "1", "0", "", "", "", "", "", "", "", "", "", "", "", "", "", "", "", "", ""], ["blow away", "1", "0", "", "", "", "", "", "", "", "", "", "", "", "", "", "", "", "", ""], ["trap shutter", "1", "0", "", "", "", "", "", "", "", "", "", "", "", "", "", "", "", "", ""], ["1038 switch", "1", "0", "", "", "", "", "", "", "", "", "", "", "", "", "", "", "", "", ""], ["", "", "", "", "", "", "", "", "", "", "", "", "", "", "", "", "", "", "", ""], ["", "", "", "", "", "", "", "", "", "", "", "", "", "", "", "", "", "", "", ""], ["", "", "", "", "", "", "", "", "", "", "", "", "", "", "", "", "", "", "", ""], ["", "", "", "", "", "", "", "", "", "", "", "", "", "", "", "", "", "", "", ""], ["", "", "", "", "", "", "", "", "", "", "", "", "", "", "", "", "", "", "", ""], ["", "", "", "", "", "", "", "", "", "", "", "", "", "", "", "", "", "", "", ""], ["", "", "", "", "", "", "", "", "", "", "", "", "", "", "", "", "", "", "", ""], ["", "", "", "", "", "", "", "", "", "", "", "", "", "", "", "", "", "", "", ""], ["", "", "", "", "", "", "", "", "", "", "", "", "", "", "", "", "", "", "", ""], ["", "", "", "", "", "", "", "", "", "", "", "", "", "", "", "", "", "", "", ""], ["", "", "", "", "", "", "", "", "", "", "", "", "", "", "", "", "", "", "", ""], ["", "", "", "", "", "", "", "", "", "", "", "", "", "", "", "", "", "", "", ""], ["", "", "", "", "", "", "", "", "", "", "", "", "", "", "", "", "", "", "", ""], ["", "", "", "", "", "", "", "", "", "", "", "", "", "", "", "", "", "", "", ""], ["", "", "", "", "", "", "", "", "", "", "", "", "", "", "", "", "", "", "", ""], ["", "", "", "", "", "", "", "", "", "", "", "", "", "", "", "", "", "", "", ""], ["", "", "", "", "", "", "", "", "", "", "", "", "", "", "", "", "", "", "", ""], ["", "", "", "", "", "", "", "", "", "", "", "", "", "", "", "", "", "", "", ""], ["", "", "", "", "", "", "", "", "", "", "", "", "", "", "", "", "", "", "", ""]], "Pulse Generation Script"="script script1\n     Generate RedTrap_compress_temp\nend script", "Start Trigger"={"Wait for start trigger?"=FALSE, "source (PFI 0)"="PFI0", "edge (rising)"=12}, "Hardware alignment quantum\n(in samples)"=1, "Inital State"="", "Idle State"="", "Active Channels"="", "Array of Waveforms"=[]} {"Hardware alignment quantum\n(in samples)" min=1 step=1; "Array of Script Triggers"."level" items=["High Level"=34, "Low Level"=35]; "Array of Script Triggers"."edge" items=["Rising Edge"=12, "Falling Edge"=13]; "Start Trigger"."edge (rising)" items=["Rising Edge"=12, "Falling Edge"=13]; "Clock Rate" min=0.0 max=200000000.0 format="%.2p"}
  out "HSDIO Status":T10={"Channel List"="0,1,2,3,4,5,6,8,9,10,11,12,14,15,16,17,18,19,20,21,22,23,24,25,26,27,28,29", "Loaded Waveforms"=["w00000002", "w00000000", "w00000008", "w00000010", "w00000018", "w00000019", "w00000011", "w00000014", "w00000016", "w00000031", "w00000033", "w00040014", "w00040016", "w00000012", "w00040010", "w00000214", "w00000216", "w02000216", "w10090A16"], "A waveform was padded"=FALSE, "final script this iteration"="script script1\r\nGenerate w00000002\r\nGenerate w00000000\r\nWait 599998\nGenerate w00000008\r\nWait 2999999\nGenerate w00000000\r\nWait 149999\nGenerate w00000010\r\nWait 49999\nGenerate w00000018\r\nWait 199998\nGenerate w00000018\r\n\r\nGenerate w00000019\r\nGenerate w00000019\r\nWait 79998\nGenerate w00000011\r\nWait 19998\nGenerate w00000011\r\n\r\nGenerate w00000014\r\nGenerate w00000016\r\nWait 1999997\nGenerate w00000016\r\n\r\nGenerate w00000000\r\n\r\nGenerate w00000031\r\nGenerate w00000033\r\nWait 999997\nGenerate w00000033\r\n\r\nGenerate w00040014\r\nGenerate w00040016\r\nGenerate w00000016\r\nWait 17\nGenerate w00000012\r\nGenerate w00000010\r\nGenerate w00040010\r\nWait 199996\nGenerate w00040010\r\n\r\nGenerate w00000014\r\nGenerate w00040014\r\nWait 199997\nGenerate w00040014\r\n\r\nGenerate w00000214\r\nGenerate w00000216\r\nWait 94998\nGenerate w00000016\r\nWait 119998\nGenerate w00000016\r\n\r\nGenerate w00000216\r\nWait 1998\nGenerate w00000216\r\n\r\nGenerate w02000216\r\nWait 179998\nGenerate w02000216\r\n\r\nGenerate w10090A16\r\nWait 1998\nGenerate w10090A16\r\n\r\nGenerate w00000016\r\nWait 699998\nGenerate w00000016\r\n\r\nGenerate w00000031\r\nGenerate w00000033\r\nWait 999997\nGenerate w00000033\r\n\r\ngenerate w00000000\r\nend script\r\n"}
  in  "HSDIO Actions":T11
  in  "DAQmx Pulse Actions":T12
  in  "DAQmx Pulse Settings":T13={"Enable DAQmx Pulses"=FALSE, "DAQmx Physical Channels"="PXI1Slot2/port0", "Clock Rate"=10000000.0, "units/sec (ms=1000)"=1000.0, "Start Trigger"={"Wait for start trigger?"=FALSE, "source"="/Dev1/PFI0", "edge"=10280}, "Timing Sequence Control"=[["camera/repump", "1", "0", "", "", "", "", "", "", "", "", "", "", "", "", "", "", "", "", "", "1000", "1000", "1000", "1000"], ["probe", "1", "0", "", "", "", "", "", "", "", "", "", "", "", "", "", "", "", "", "", "", "", "", ""], ["bias field", "1", "0", "", "", "", "", "", "", "", "", "", "", "", "", "", "", "", "", "", "", "", "", ""], ["switch 1 MOT to PGC freq shift", "1", "0", "", "", "", "", "", "", "", "", "", "", "", "", "", "", "", "", "", "", "", "", ""], ["B field", "1", "0", "", "", "", "", "", "", "", "", "", "", "", "", "", "", "", "", "", "", "", "", ""], ["trigger PD1", "1", "0", "", "", "", "", "", "", "", "", "", "", "", "", "", "", "", "", "", "", "", "", ""], ["rf switch 2 cooling laser on/off", "1", "0", "", "", "", "", "", "", "", "", "", "", "", "", "", "", "", "", "", "", "", "", ""], ["Bob switch", "1", "0", "", "", "", "", "", "", "", "", "", "", "", "", "", "", "", "", "", "", "", "", ""], ["switch 3 894nm", "1", "0", "", "", "", "", "", "", "", "", "", "", "", "", "", "", "", "", "", "", "", "", ""], ["clock trigger", "1", "0", "", "", "", "", "", "", "", "", "", "", "", "", "", "", "", "", "", "", "", "", ""], ["Raman", "1", "0", "", "", "", "", "", "", "", "", "", "", "", "", "", "", "", "", "", "", "", "", ""], ["684 shutter", "1", "0", "", "", "", "", "", "", "", "", "", "", "", "", "", "", "", "", "", "", "", "", ""], ["repumper switch 2", "1", "0", "", "", "", "", "", "", "", "", "", "", "", "", "", "", "", "", "", "", "", "", ""], ["further PGC", "1", "0", "", "", "", "", "", "", "", "", "", "", "", "", "", "", "", "", "", "", "", "", ""], ["pumping laser switch 2", "1", "0", "", "", "", "", "", "", "", "", "", "", "", "", "", "", "", "", "", "", "", "", ""], ["Raman 2", "1", "0", "", "", "", "", "", "", "", "", "", "", "", "", "", "", "", "", "", "", "", "", ""], ["MOT beam on/off switch 2", "1", "0", "", "", "", "", "", "", "", "", "", "", "", "", "", "", "", "", "", "", "", "", ""], ["push beam switch 2", "1", "0", "", "", "", "", "", "", "", "", "", "", "", "", "", "", "", "", "", "", "", "", ""], ["532 AOM", "1", "0", "", "", "", "", "", "", "", "", "", "", "", "", "", "", "", "", "", "", "", "", ""], ["Andor Luca Trigger", "1", "0", "", "", "", "", "", "", "", "", "", "", "", "", "", "", "", "", "", "", "", "", ""], ["trigger PD2", "1", "0", "", "", "", "", "", "", "", "", "", "", "", "", "", "", "", "", "", "", "", "", ""], ["1038 switch", "1", "0", "", "", "", "", "", "", "", "", "", "", "", "", "", "", "", "", "", "", "", "", ""], ["459 switch", "1", "0", "", "", "", "", "", "", "", "", "", "", "", "", "", "", "", "", "", "", "", "", ""], ["", "", "", "", "", "", "", "", "", "", "", "", "", "", "", "", "", "", "", "", "", "", "", ""], ["", "", "", "", "", "", "", "", "", "", "", "", "", "", "", "", "", "", "", "", "", "", "", ""], ["", "", "", "", "", "", "", "", "", "", "", "", "", "", "", "", "", "", "", "", "", "", "", ""], ["", "", "", "", "", "", "", "", "", "", "", "", "", "", "", "", "", "", "", "", "", "", "", ""], ["", "", "", "", "", "", "", "", "", "", "", "", "", "", "", "", "", "", "", "", "", "", "", ""], ["", "", "", "", "", "", "", "", "", "", "", "", "", "", "", "", "", "", "", "", "", "", "", ""], ["", "", "", "", "", "", "", "", "", "", "", "", "", "", "", "", "", "", "", "", "", "", "", ""], ["", "", "", "", "", "", "", "", "", "", "", "", "", "", "", "", "", "", "", "", "", "", "", ""], ["0", "", "", "", "", "", "", "", "", "", "", "", "", "", "", "", "", "", "", "", "", "", "", ""]]} {"Start Trigger"."edge" items=["Rising"=10280, "Falling"=10171]; "Clock Rate" min=0.0 max=200000000.0 format="%.2p"}
  in  "DDS Actions":T14
  out "DDS Initialized":bool
  in  "DDS Settings":T15={"Enable DDS"=TRUE, "Array of DDS Boxes"=[]} {"Array of DDS Boxes"."Array of DDS Channels (4)"."Channel Parameters"."Ref Clock Rate [kHz]" min=0.0}
  in  "box #":i32=2 min=0 step=1
  out "CFR3":u8[][](array[numeric])=[[31, 63, 192, 0], [31, 63, 192, 0], [31, 63, 192, 0], [31, 63, 192, 0]]
  out "CFR2":u8[][](array[numeric])=[[1, 64, 8, 32], [1, 64, 8, 32], [1, 64, 8, 32], [1, 64, 8, 32]]
  out "CFR1":u8[][](array[numeric])=[[0, 0, 0, 2], [0, 0, 0, 2], [0, 0, 0, 2], [0, 0, 0, 242]]
  in  "Check DDS":bool
  in  "HP83712B Synthesized Signal Generator Array":T25
  in  "Load HP83712B Settings":bool
  in  "Load HP83623A Settings":bool
  in  "Load HP8662A Settings":bool
  in  "HP8662A Synthesized Signal Generator Array":T25
  in  "HP83623A Generator Settings Array":T27
  in  "Andor setup":T29={"Andor Path"=path "C:/Users/QC/Documents/Cesium_project/Andor_picutres_temp", "Copy any Andor files"=FALSE, "Wait time before copying Andor files (ms)"=0}
  in  "Recent Image Display Maximum":u16=9000 caption="Display Maximum"
  in  "Recent Image Display Minimum":u16=2000 caption="Display Minimum"
  in  "Recent Image Dynamic scaling":bool=TRUE caption="Dynamic scaling"
  in  "Image Display Maximum":u16=9000 caption="Display Maximum"
  in  "Image Display Minimum":u16=4000 caption="Display Minimum"
  in  "Image Dynamic scaling":bool=TRUE caption="Dynamic scaling"
  out "Set?":bool
  in  "Set Current Average Image as Background":bool
  out "Image Array for whole experiment":T30[][][](array[plugin-control]) caption="(Iterations, Measurements, Shots. Scaling above.)"
  in  "Hamamatsu Setup":T31={"Analog Gain (0-5)"=4, "Exposure Time"=0.01, "EM Gain (0-255)"=0, "Trigger Polarity"="ATP P", "External Trigger Mode"="EMD E", "Scan Speed"="SSP H", "External Trigger Source"="ESC B", "Scan Mode"="SMD N", "Super Pixel Binning\n(if enabled in Scan Mode)"="SPX 1", "Camera Sub-array acquisition region\n(if enabled in scan mode)"={"Left"=0, "Top"=0, "Width"=0, "Height"=0}, "Use camera?"=FALSE, "# image buffers"=100, "shots per measurement"=100, "Force images to U16"=FALSE, "Low Light Sensitivity"="LLS 0", "cooling"="CSW F", "fan"="FAN F", "Frame Grabber acquisition region"={"Left"=0, "Top"=0, "Right"=0, "Bottom"=0}} {"Frame Grabber acquisition region"."Bottom" max=512 step=1; "Frame Grabber acquisition region"."Right" max=512 step=1; "Frame Grabber acquisition region"."Top" max=512 step=1; "Frame Grabber acquisition region"."Left" max=512 step=1; "shots per measurement" min=0 step=1; "# image buffers" min=0 step=1; "Camera Sub-array acquisition region\n(if enabled in scan mode)"."Height" min=16 max=512 step=16; "Camera Sub-array acquisition region\n(if enabled in scan mode)"."Width" min=16 max=512 step=16; "Camera Sub-array acquisition region\n(if enabled in scan mode)"."Top" max=496 step=16; "Camera Sub-array acquisition region\n(if enabled in scan mode)"."Left" max=496 step=16; "Analog Gain (0-5)" max=5 step=1}
  out "Average of All Images from experiment":T30(plugin-control) caption="Average of All Images (dynamically scaled)"
  out "Histogram of ROI Sum over All Images for last ROI":T32
  in  "# intervals (mutli-shot)":i32=50
  out "Camera Temperature":dbl=-80.0 format="%_5g"
  out "Image Array for most recent measurement":T30[](array[plugin-control])=["LL Ring num 98", "LL Ring num 99"] caption="(By shot.  Scaling above.)"
  out "Array of ROI sums":dbl[][][][](array[numeric])
  out "Image 3":T30(plugin-control)
  out "Large Image Viewer":T30(plugin-control)
  in  "Background image Dynamic scaling":bool caption="Dynamic scaling"
  in  "Background Image Display Maximum":u16 caption="Display Maximum"
  in  "Background Image Display Minimum":u16 caption="Display Minimum"
  out "Backgound Subtracted Average Image":T30(plugin-control) caption="(dynamic scaling)"
  out "Background Subtracted Image Array":T30[][][](array[plugin-control])=[[["tmp %d0 0 0 0"], ["tmp %d0 0 1 0"]], [["tmp %d0 1 0 0"], ["tmp %d0 1 1 0"]]] caption="(Cycles, Iterations, Measurements, Shots, scaling above)"
  in  "Run Background Subtraction":bool
  out "Background Image":T30(plugin-control) caption="(dynamic scaling)"
  in  "Iteration Graph Settings":T33={"Plot Regions"="32", "Plot Shots"="0,1"}
  out "Iteration Graph":dbl[][](graph)
  out "Counters Chart 3":u32[][](graph)
  out "counter data":u32[][](array[numeric])
  out "Counters Chart":u32[][](graph)
  in  "Counter Settings":T34 {"Array of Counter Settings"."Binwidth (ms)" format="%0.2f"}
  out "current counter totals":u32[](array[numeric])
  out "Counters Chart 2":u32[](graph)
  out "Counters Chart 4":u32[][](graph)
  in  "Filter Cluster":T35
  out "AO Equations are valid":bool=TRUE
  in  "Analog Output Actions":cluster{"Graph Analog Output":bool}
  in  "Analog Output Parameters":T36={"Enable Analog Out?"=FALSE, "Physical Channel"="PXI1Slot2/ao0:2", "Minimum Value"=-10.0, "Maximum Value"=10.0, "Samples per second"=0.0, "Total AO Time (seconds)"=0.0, "Start Trigger"={"Wait for start trigger?"=FALSE, "source"="/Dev1/PFI0", "edge"=10280}, "Analog Output Waveforms (channel, time)"=[]} {"Start Trigger"."edge" items=["Rising"=10280, "Falling"=10171]; "Maximum Value" format="%0.2f"; "Minimum Value" format="%0.2f"}
  out "Waveform Graph":waveform(dbl)[](graph)=[{"t0"=timestamp(0 s since 1904-01-01), "dt"=5e-06, "Y"=array[132542 elements]}, {"t0"=timestamp(0 s since 1904-01-01), "dt"=5e-06, "Y"=array[132542 elements]}, {"t0"=timestamp(0 s since 1904-01-01), "dt"=5e-06, "Y"=array[132542 elements]}, {"t0"=timestamp(0 s since 1904-01-01), "dt"=5e-06, "Y"=array[132542 elements]}, {"t0"=timestamp(0 s since 1904-01-01), "dt"=5e-06, "Y"=array[132542 elements]}, {"t0"=timestamp(0 s since 1904-01-01), "dt"=5e-06, "Y"=array[132542 elements]}, {"t0"=timestamp(0 s since 1904-01-01), "dt"=5e-06, "Y"=array[132542 elements]}, {"t0"=timestamp(0 s since 1904-01-01), "dt"=5e-06, "Y"=array[132542 elements]}]
  in  "PI Piezo Settings":T37
  in  "Pi Piezo Actions":cluster{"Connect":bool, "Set Position":bool}
  out "PI Piezo Status":T40=[{"Identification"="PI-E816 V3.25", "SN out"="", [{"Axis"="B", "Servo"=TRUE, "Position"=45.4887}, {"Axis"="C", "Servo"=TRUE, "Position"=43.7483}, {"Axis"="D", "Servo"=TRUE, "Position"=50.868}, {"Axis"="E", "Servo"=FALSE, "Position"=1.7353}, {"Axis"="F", "Servo"=FALSE, "Position"=1.1544}, {"Axis"="G", "Servo"=FALSE, "Position"=7.6067}, {"Axis"="H", "Servo"=TRUE, "Position"=25.0983}, {"Axis"="I", "Servo"=TRUE, "Position"=70.0382}, {"Axis"="J", "Servo"=TRUE, "Position"=28.3592}]}]
  in  "Notes":string="The retention problem was with the 2d shutter turning on between shots which was messing up the retention. i fixed this and we are back to perfect retention, or nearly.\n\nAligned the 1038 to ROI 32.\n\nGetting the blue aligned to ROI32 by scanning the piezo axes and blowing away using the single site pumper.    doing a rough scan first since i have no idea where the alignment might be currently ( the array was moved around quite a lot to get it working again)" caption="(please no &)"
  in  "Save Notes to File":bool
  in  "Load Notes from File":bool
  out "Measurement Chart":dbl[][](graph)
  in  "Measurement Chart Settings":T41
  out "TTL inputs":bool[](array[boolean])
  in  "TTL input":T42
  out "Experiment is Running":bool
  out "Error LED":bool caption="Error"
  in  "stop":bool
  # "Parameters will be evaluated once at the beginning of the experiment from top to bottom, \nso any parameter may depend on all those above it.\nVariables will be evaluated each iteration.\nParameters and Variables may be used in various other experiment settings, as noted.\nSee LabView Help -> Formula Node and Expression Node Functions for a list of available functions."
  # "Regions of Interest -->"
  # "Shots\n   |\n  V"
  # "Counters -->"
  # "Counter\n    bins\n       |\n      V"
  # "TTL low = locked, TTL high = unlocked"
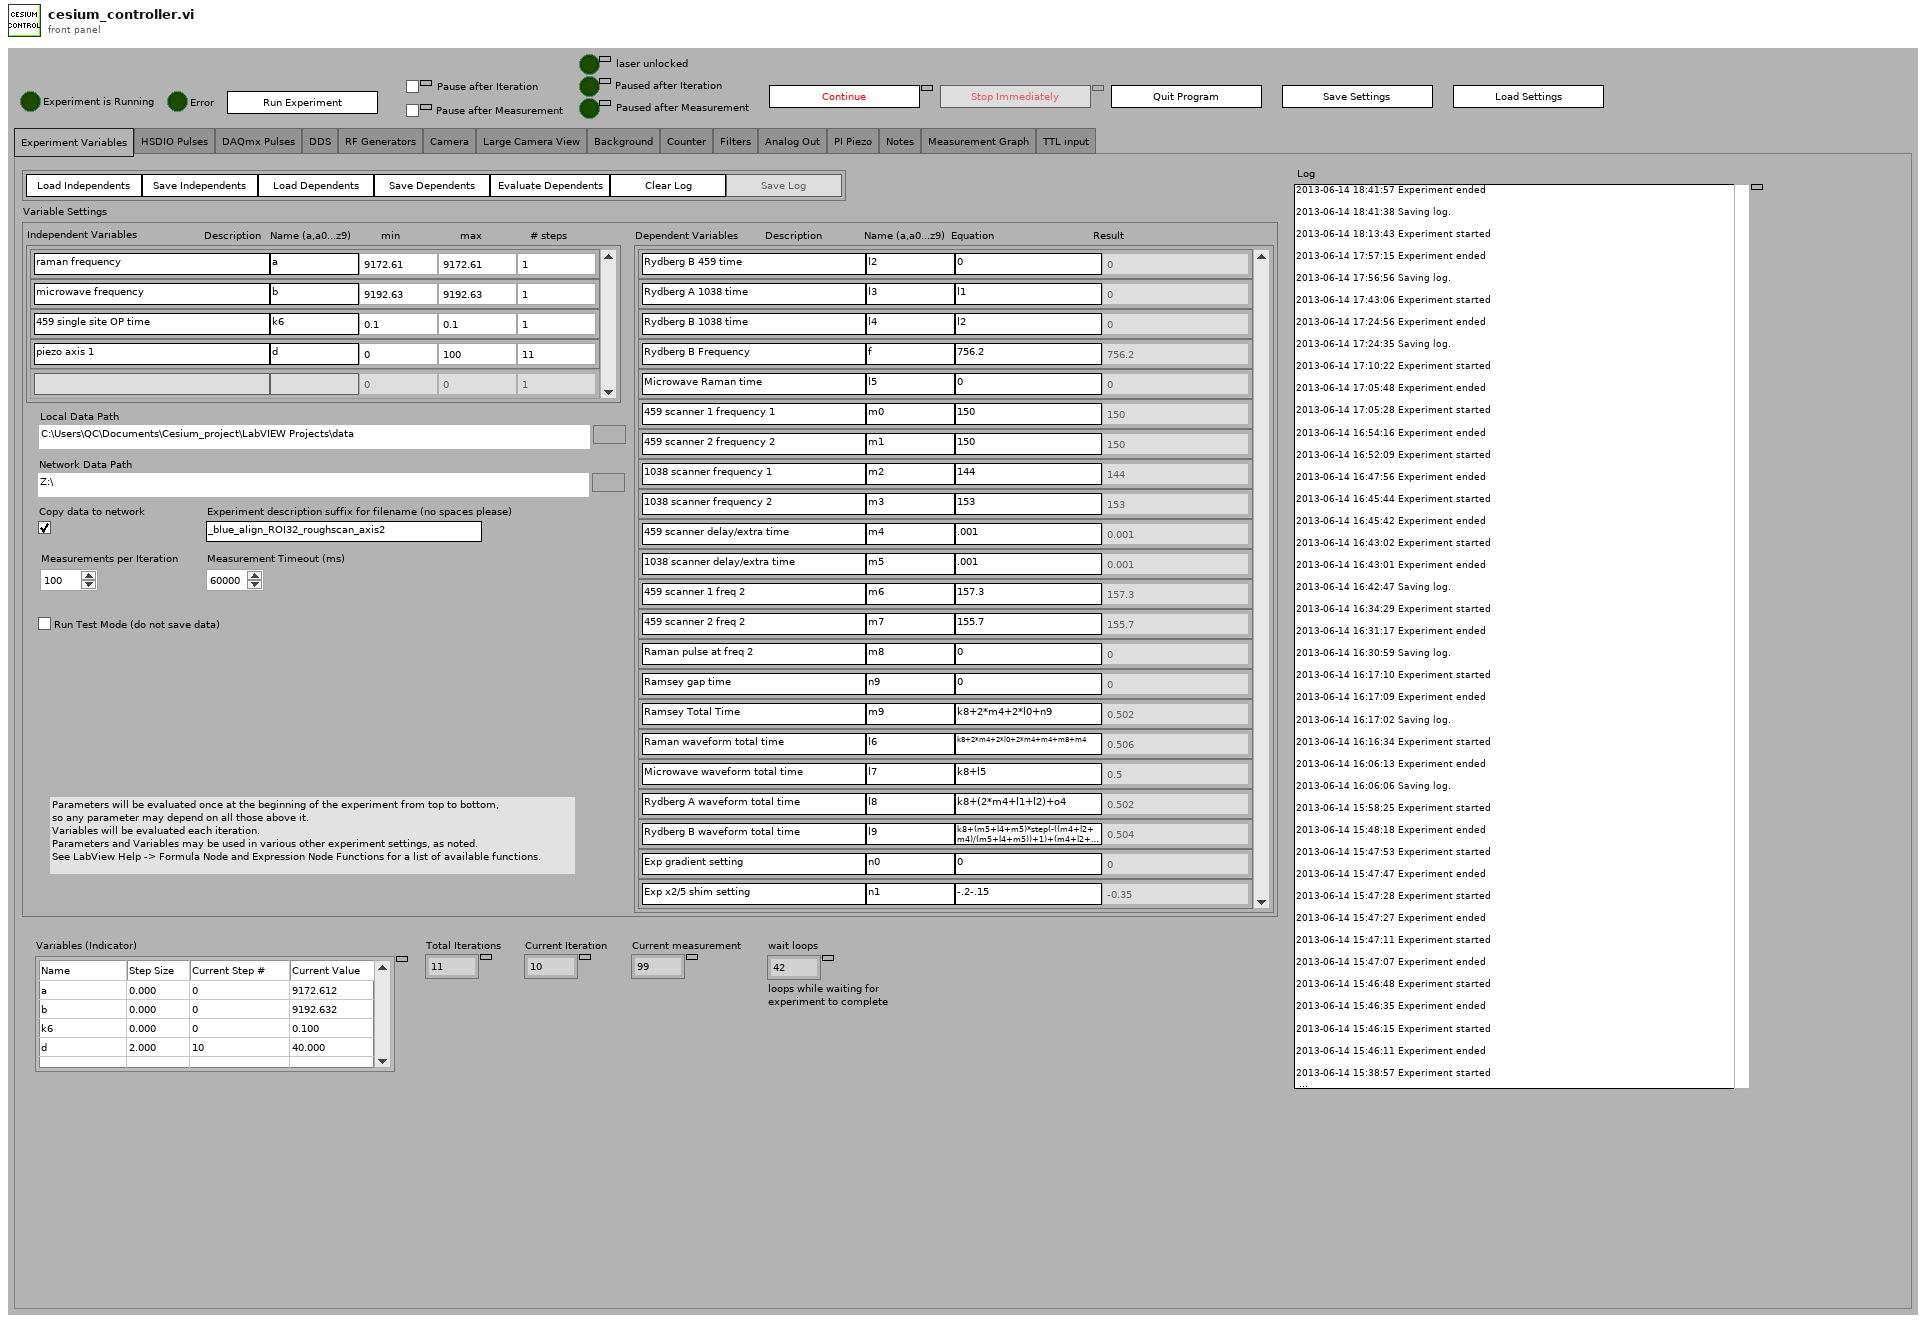
[diagram p1: front panel]
types:
  T1 = enum32{"Experiment Variables", "HSDIO Pulses", "DAQmx Pulses", "DDS", "RF Generators", "Camera", "Large Camera View", "Background", "Counter", "Filters", "Analog Out", "PI Piezo", "Notes", "Measurement Graph", "TTL input"}
  T2 = cluster{"Load Independents":bool, "Save Independents":bool, "Load Dependents":bool, "Save Dependents":bool, "Evaluate Dependents":bool, "Clear Log":bool, "Save Log":bool}
  T3 = typedef "ExperimentVariables.lvclass/Variable_Settings.ctl" = cluster{"Measurements per Iteration":i32, "Local Data Path":path, "Experiment description suffix for filename (no spaces please)":string, "Network Data Path":path, "Copy data to network":bool, "Measurement Timeout (ms)":u32, "Independent Variables":cluster{"Description":string, "Name (a,a0...a9)":string, "min":dbl, "max":dbl, "# steps":u32}[], "Dependent Variables":cluster{"Description":string, "Name (a,a0...a9)":string, "Equation":string, "Result":dbl}[], "Run Test Mode":bool}
  T4 = typedef "HSDIO.lvclass/HSDIO_settings.ctl" = cluster{"Enable HSDIO Pulses":bool, "Resource Name":refnum<k15>, "Clock Rate":dbl, "Array of Script Triggers":cluster{"trigger id (script trigger 0)":T5, "source (PFI 0)":T6, "Trigger Type":enum32{"Edge", "Level"}, "edge":T7, "level":T8}[], "Channels Control":string[][], "Pulse Generation Script":string, "Start Trigger":cluster{"Wait for start trigger?":bool, "source (PFI 0)":T6, "edge (rising)":T7}, "Hardware alignment quantum\n(in samples)":u16, "Inital State":string, "Idle State":string, "Active Channels":string, "Array of Waveforms":T9[]}
  T5 = typedef "niHSDIO_ctl Trigger Script - trigID Values (Ring).ctl" = string
  T6 = typedef "niHSDIO_ctl Trigger Source Values (Ring).ctl" = string
  T7 = typedef "niHSDIO_ctl Trigger DigEdge - Edge Values (Ring).ctl" = i32
  T8 = typedef "niHSDIO_ctl Trigger DigLvl - Level Values (Ring).ctl" = i32
  T9 = typedef "HSDIO.lvclass/waveform.ctl" = cluster{"name":string, "transitions":u32[], "states":u8[][]}
  T10 = cluster{"Channel List":string, "Loaded Waveforms":string[], "A waveform was padded":bool, "final script this iteration":string}
  T11 = cluster{"Load Channels Control":bool, "Save Channels Control":bool, "Load Script":bool, "Save Script":bool, "Open NI Script Editor":bool, "Edit a Waveform":bool}
  T12 = cluster{"Load Waveform from File":bool, "Save Waveform to File":bool, "Load Channels from File":bool, "Save Channels to File":bool}
  T13 = typedef "DAQmx_pulse_out.lvclass/settings.ctl" = cluster{"Enable DAQmx Pulses":bool, "DAQmx Physical Channels":tag, "Clock Rate":dbl, "units/sec (ms=1000)":dbl, "Start Trigger":cluster{"Wait for start trigger?":bool, "source":tag, "edge":i32}, "Timing Sequence Control":string[][]}
  T14 = cluster{"Initialize DDS Boxes":bool, "Load DDS":bool}
  T15 = typedef "DDS_Settings_Cluster.ctl" = cluster{"Enable DDS":bool, "Array of DDS Boxes":T16}
  T16 = typedef "Array_of_DDS_Boxes.ctl" = T17[]
  T17 = typedef "DDS_box_cluster.ctl" = cluster{"DDS box device reference":T18, "Array of DDS Channels (4)":T20, "Enable":bool, "Description":string}
  T18 = typedef "DDS_box_device_reference.ctl" = cluster{"NI USB-8451 device reference":T19, "DIO port":u8, "Serial Clock Rate [kHz]":u16}
  T19 = typedef "ni845xControl.ctl" = refnum<k21>
  T20 = typedef "DDS.lvclass/array_of_DDS_channels.ctl" = T21[]
  T21 = typedef "DDS.lvclass/DDS_channel.ctl" = cluster{"Power":bool, "Channel Parameters":cluster{"Ref Clock Rate [kHz]":dbl, "Full Scale Output\nPower [dBm]":dbl}, "RAM Enable":bool, "RAM Dest Type":u8, "RAM Default":cluster{"Frequency [MHz]":dbl, "Amplitude [dBm]":dbl, "Phase Offset [rad]":dbl}, "Array of DDS Profiles (8)":T22, "Description":string}
  T22 = typedef "DDS.lvclass/array_of_DDS_profiles.ctl" = T23[]
  T23 = typedef "DDS_profile.ctl" = cluster{"Single Tone":cluster{"Frequency [MHz]":dbl, "Amplitude [dBm]":dbl, "Phase Offset [rad]":dbl}, "RAM Mode ":T24, "Zero-crossing":bool, "No Dwell High":bool, "Function/Static":bool, "RAM Function Settings":string[], "RAM Static Array":dbl[], "Description":string}
  T24 = typedef "DDS RAM mode.ctl" = enum16{"Direct Switch", "Ramp Up", "Bidirectional Ramp", "Continuous Bidirectional Ramp", "Continuous Recirculate", "Direct Switch 2", "Direct Switch 3", "Direct Switch 4"}
  T25 = typedef "GPIB.lvclass/RF_Generator_settings_array.ctl" = T26[]
  T26 = typedef "GPIB.lvclass/RF_Generator_settings.ctl" = cluster{"Enable":bool, "Description":string, "GPIB channel #":u8, "Frequency (MHz)":dbl, "Power (dBm)":dbl}
  T27 = typedef "HP83623A_RF_Generator.lvclass/HP83623A_array.ctl" = T28[]
  T28 = typedef "HP83623A.ctl" = cluster{"Frequency (Hz)":dbl, "Power (dBm)":dbl, "Enabled":bool, "initialized":bool, "RF Output On/Off":bool, "External Trigger?":bool, "VISA Session":refnum<visa-resource-name>, "Generator Name":string}
  T29 = typedef "Andor_settings.ctl" = cluster{"Andor Path":path, "Copy any Andor files":bool, "Wait time before copying Andor files (ms)":u16}
  T30 = typedef "IMAQ Image.ctl" = refnum<image>
  T31 = typedef "Hamamatsu_C9100-13.lvclass/camera_setup.ctl" = cluster{"Analog Gain (0-5)":u8, "Exposure Time":dbl, "EM Gain (0-255)":u8, "Trigger Polarity":string, "External Trigger Mode":string, "Scan Speed":string, "External Trigger Source":string, "Scan Mode":string, "Super Pixel Binning\n(if enabled in Scan Mode)":string, "Camera Sub-array acquisition region\n(if enabled in scan mode)":cluster{"Left":u16, "Top":u16, "Width":u16, "Height":u16}, "Use camera?":bool, "# image buffers":i32, "shots per measurement":i32, "Force images to U16":bool, "Low Light Sensitivity":string, "cooling":string, "fan":string, "Frame Grabber acquisition region":cluster{"Left":i32, "Top":i32, "Right":i32, "Bottom":i32}}
  T32 = typedef "histogram.ctl" = cluster{"X Values":dbl[], "Histogram: h(x)":i32[]}[]
  T33 = cluster{"Plot Regions":string, "Plot Shots":string}
  T34 = typedef "Counter.lvclass/Counter_Settings_Control.ctl" = cluster{"Enable Counters":bool, "Array of Counter Settings":cluster{"Counter Channel":tag, "Time-Bin Clock Channel":tag, "Binwidth (ms)":dbl}[]}
  T35 = typedef "filters.ctl" = cluster{"Counter Filter thresholds":u32[][], "Data Filters\nROI Minimum Thresholds":u64[][]}
  T36 = typedef "Analog_Output.lvclass/AO_settings.ctl" = cluster{"Enable Analog Out?":bool, "Physical Channel":tag, "Minimum Value":dbl, "Maximum Value":dbl, "Samples per second":dbl, "Total AO Time (seconds)":dbl, "Start Trigger":cluster{"Wait for start trigger?":bool, "source":tag, "edge":i32}, "Analog Output Waveforms (channel, time)":dbl[][]}
  T37 = typedef "PI_Piezo.lvclass/settings.ctl" = cluster{"Enable":bool, "Array of Piezo Controllers":T38[]}
  T38 = typedef "PI_Piezo.lvclass/piezo_controller.ctl" = cluster{"Enable":bool, "Serial No.":string, "Array of Piezo Channels":T39[]}
  T39 = typedef "PI_Piezo.lvclass/piezo_channel.ctl" = cluster{"Servo":bool, "Set Position":dbl}
  T40 = typedef "PI_Piezo.lvclass/status.ctl" = cluster{"Identification":string, "SN out":string, cluster{"Axis":string, "Servo":bool, "Position":dbl}[]}[]
  T41 = typedef "measurement_graph.ctl" = cluster{"Which regions to plot (comma separated)":string, "Which shot to plot":u8}
  T42 = typedef "TTL_input.lvclass/TTL_input_settings.ctl" = cluster{"Enable":bool, "lines":tag}
  T43 = typedef "gui_execution_controls.ctl" = cluster{"stop":refnum<vi>, "Pause after Measurement":refnum<vi>, "Paused":refnum<vi>, "Pause after Iteration":refnum<vi>}
  T44 = typedef "counter_graph_refnums.ctl" = cluster{"Counter Data Refnum":refnum<vi>, "Counters Chart 3 Refnum":refnum<vi>, "Counters Chart Refnum":refnum<vi>, "current counter totals Refnum":refnum<vi>, "Counters Chart 2 Refnum":refnum<vi>, "Counters Chart 4 Refnum":refnum<vi>}
  T45 = typedef "gui_refnum.ctl" = cluster{"current counter totals":refnum<vi>, "Initialize DDS Boxes":refnum<vi>, "Array of DDS Boxes":refnum<vi>, "Error LED":refnum<vi>, "Experiment is Running":refnum<vi>, "DDS Initialized":refnum<vi>, "Run Experiment":refnum<vi>, "Quit Program":refnum<vi>, "Histogram of ROI Sum over All Images for last ROI":refnum<vi>, "Counters Chart":refnum<vi>, "Image Array for whole experiment":refnum<vi>, "Counter Refnums":T44, "Stop/Pause refnum cluster":T43, "Image Array for most recent measurement":refnum<vi>, "Iteration Graph":refnum<vi>, "PI Piezo Status":refnum<vi>, "Measurement Chart ref":refnum<vi>}
  T46 = enum16{"reset", "experiment start", "experiment end", "quit"}
  T47 = typedef "DialogType.ctl" = u16
  T48 = enum8{"Enabled", "Disabled", "Disabled and Grayed Out"}
  T49 = cluster{"Description":string, "Name (a,a0...a9)":string, "min":dbl, "max":dbl, "# steps":u32}
  T50 = cluster{"Description":string, "Name (a,a0...a9)":string, "Equation":string, "Result":dbl}
  T51 = typedef "all_settings.ctl" = cluster{"Variable Settings":T3, "HSDIO Settings":T4, "DAQmx Pulse Settings":T13, "DDS Settings":T15, "Camera settings":T31, "Counter Settings":T34, "Filter Cluster":T35, "Analog Output Parameters":T36, "Notes":string, "HP83623A Generator Settings Array":T27, "Iteration Graph Settings":cluster{"Plot Regions":string, "Plot Shots":string}, "PI Piezo Settings":T37, "Andor settings":T29, "Measurement Chart Settings":T41, "HP8662A Synthesized Signal Generator Array":T25, "HP83712B Synthesized CW Generator Array":T25, "TTL input":T42}
  T52 = cluster{"Wait for start trigger?":bool, "source (PFI 0)":T6, "edge (rising)":T7}
  T53 = cluster{"Description":string, "Name (a,a0...a9)":string, "min":dbl, "max":dbl, "# steps":u32}[]
  T54 = cluster{"Description":string, "Name (a,a0...a9)":string, "Equation":string, "Result":dbl}[]
  T55 = cluster{"Wait for start trigger?":bool, "source":tag, "edge":i32}
  T56 = typedef "Image Type" = u32
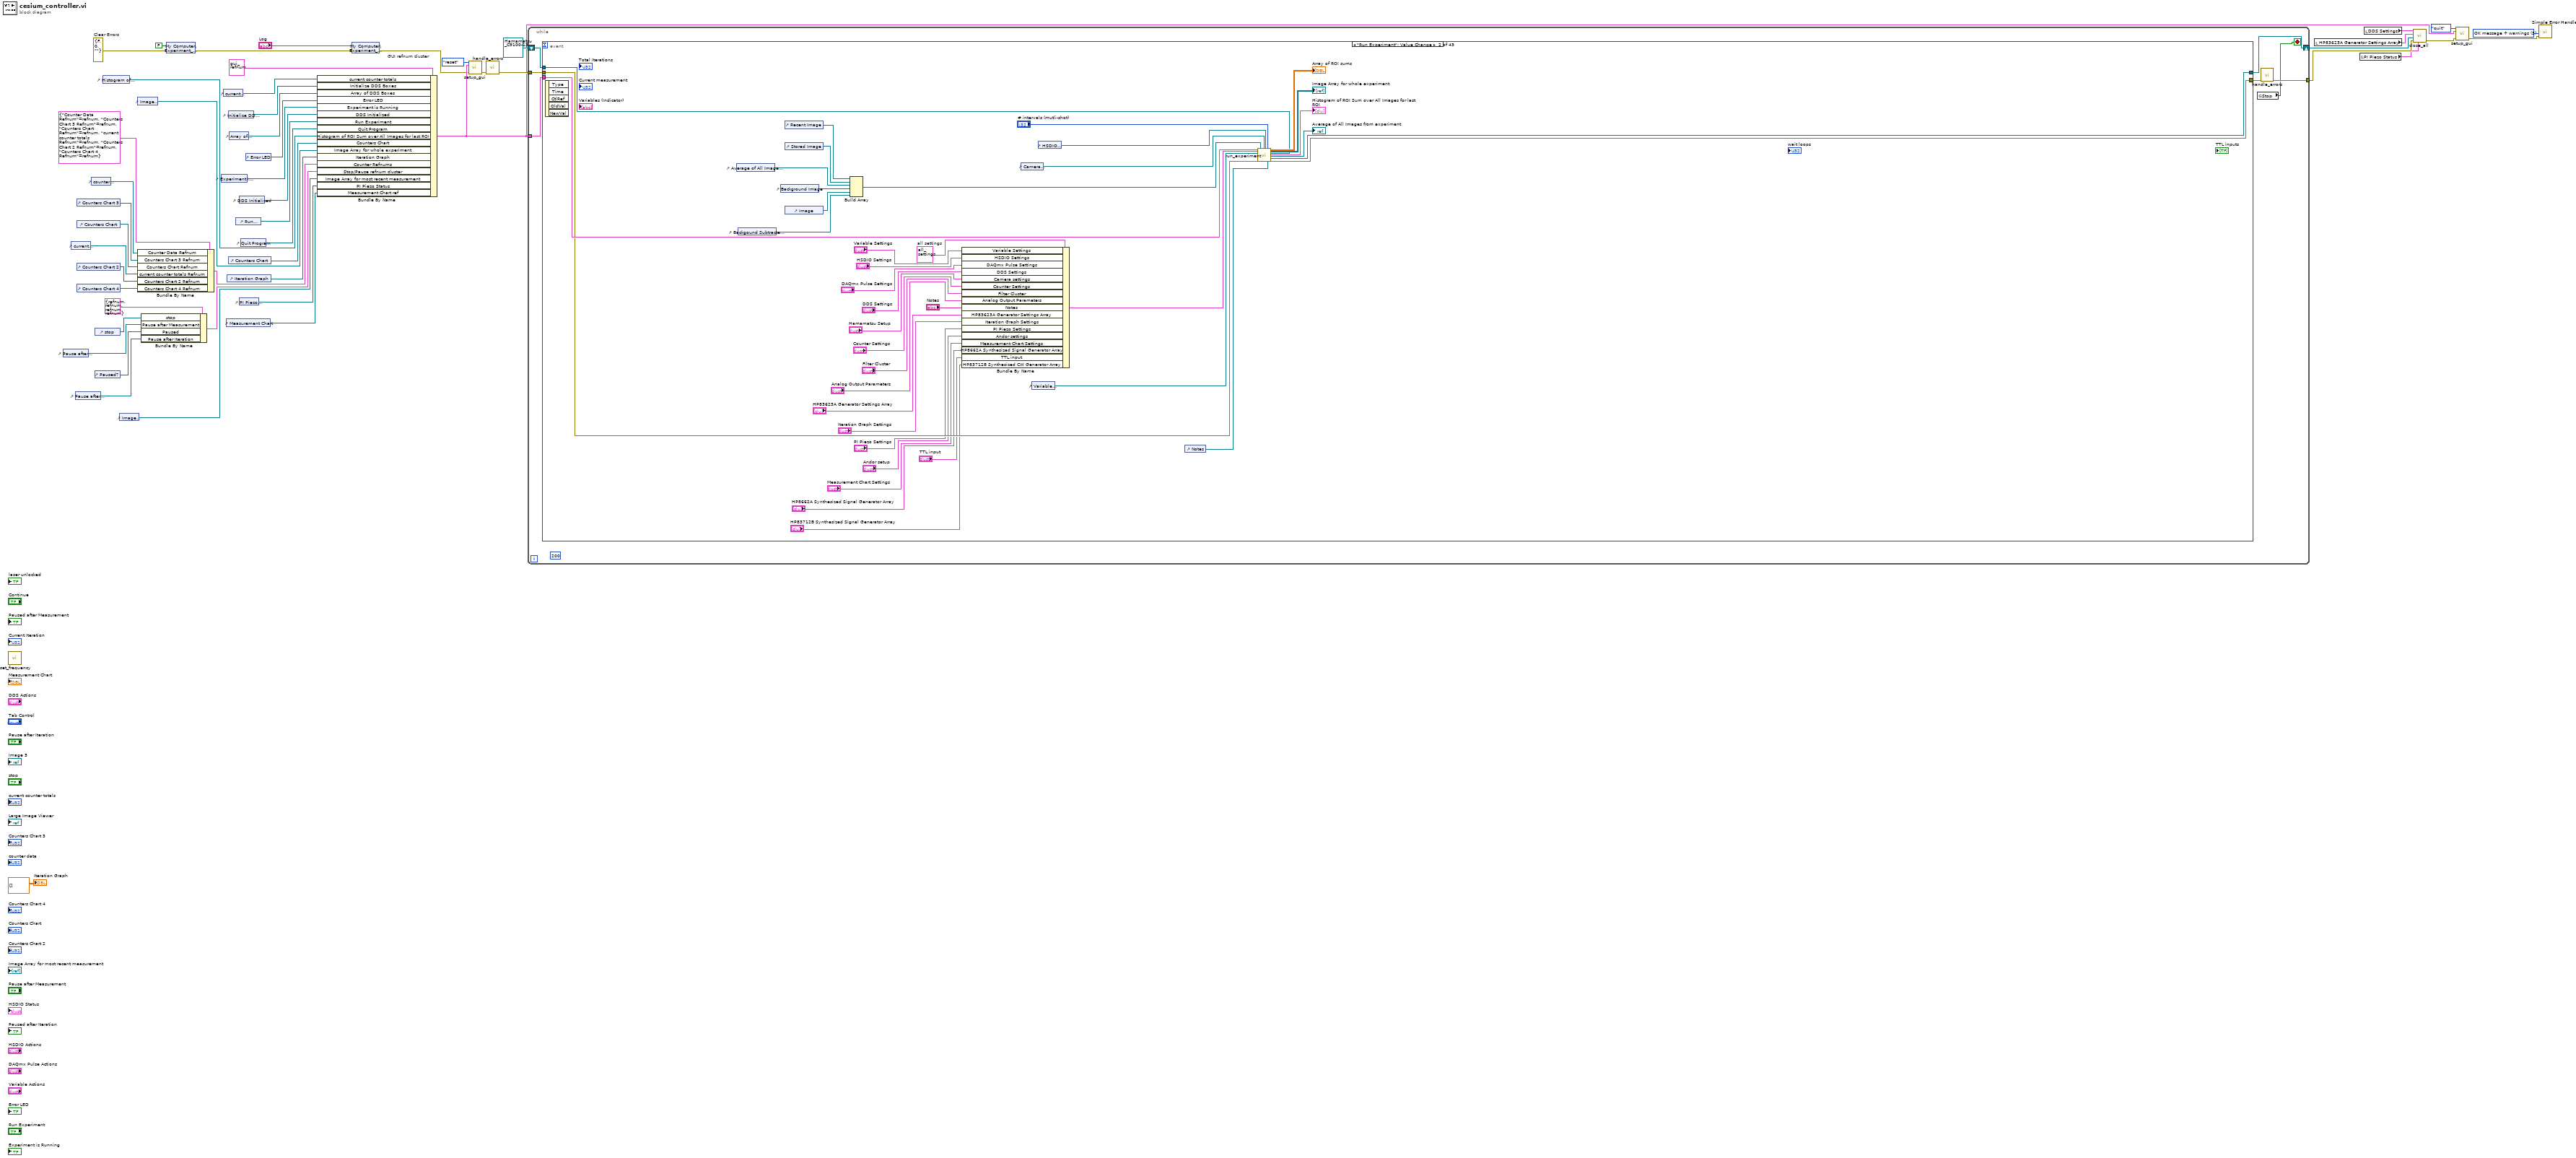
[diagram p0: block diagram]
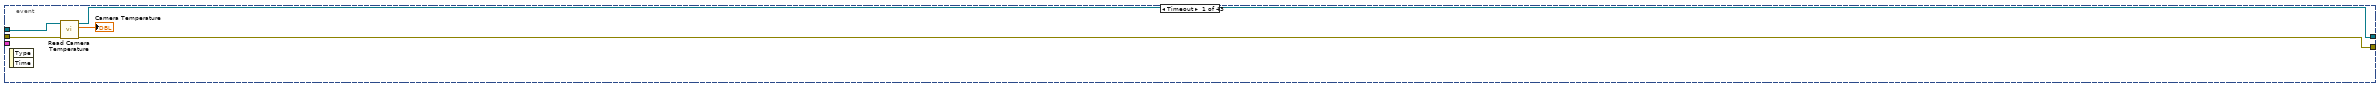
[diagram p2: hidden frame]
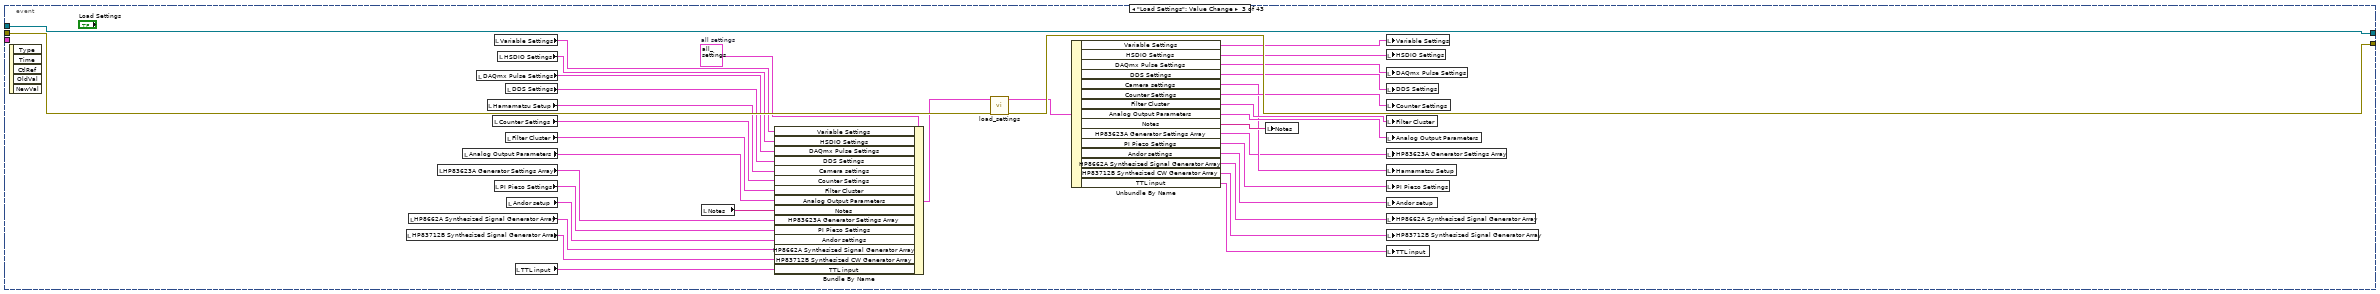
[diagram p3: hidden frame]
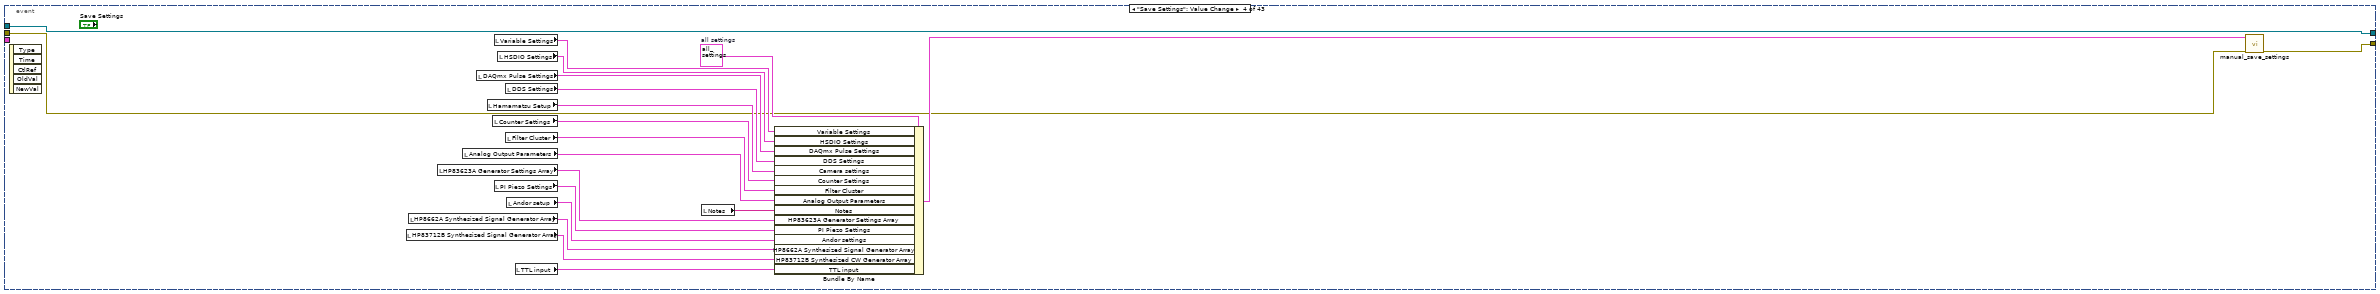
[diagram p4: hidden frame]
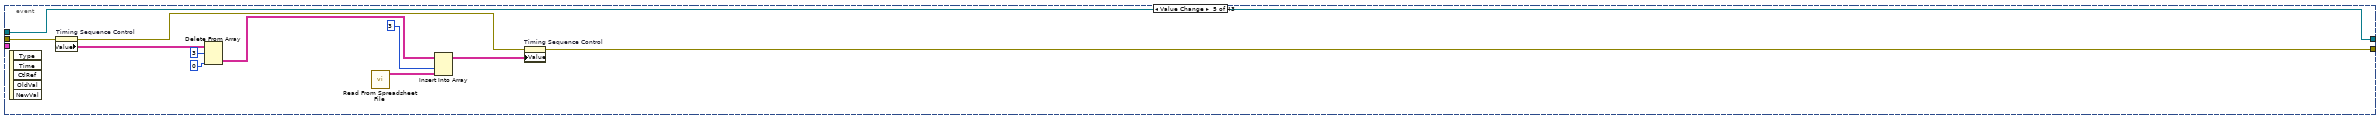
[diagram p5: hidden frame]
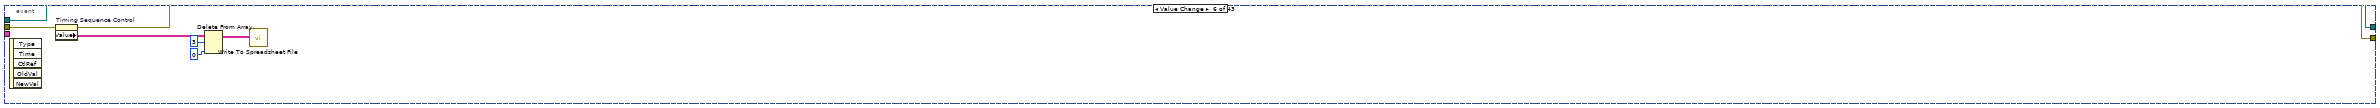
[diagram p6: hidden frame]
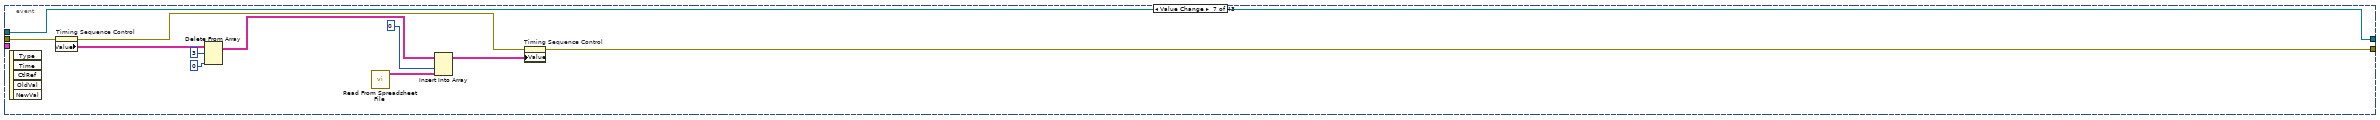
[diagram p7: hidden frame]
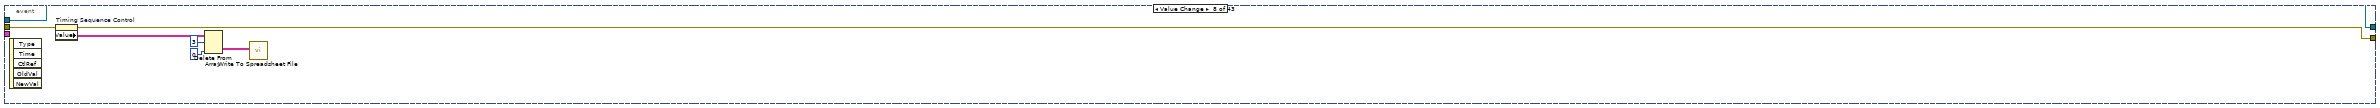
[diagram p8: hidden frame]
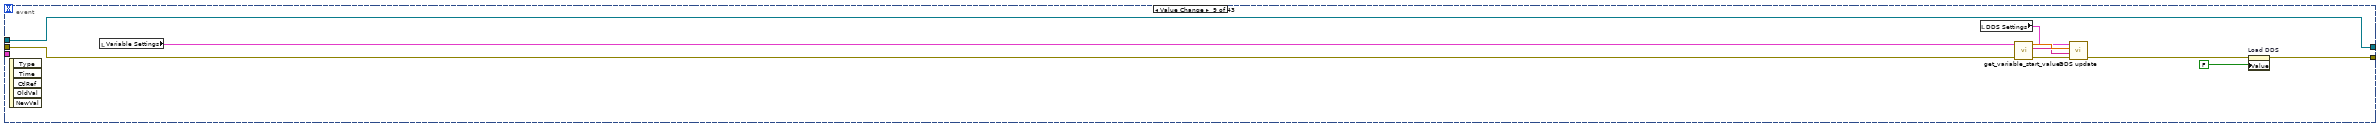
[diagram p9: hidden frame]
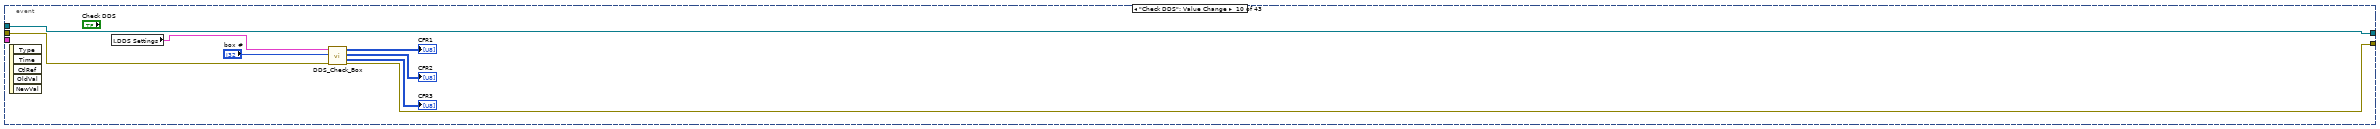
[diagram p10: hidden frame]
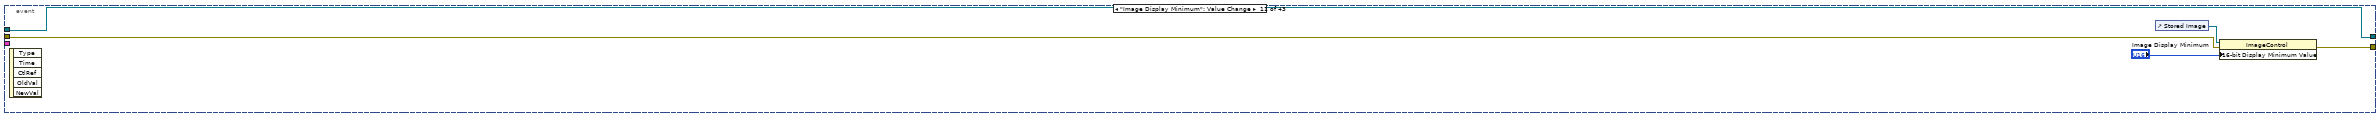
[diagram p11: hidden frame]
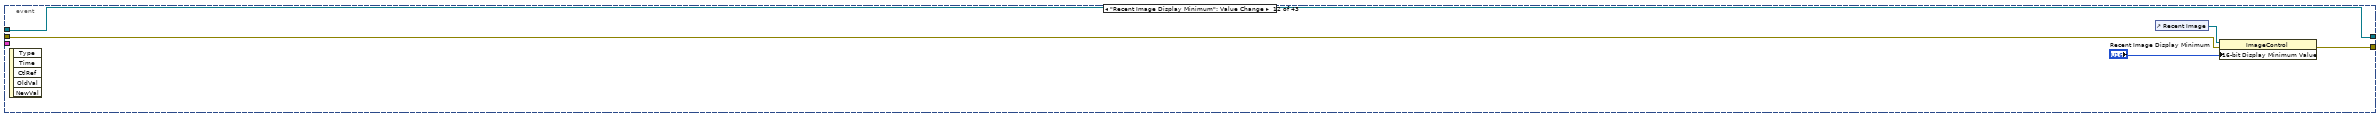
[diagram p12: hidden frame]
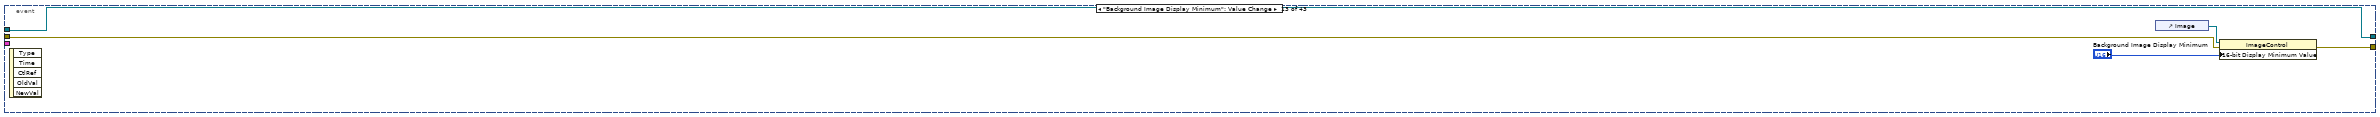
[diagram p13: hidden frame]
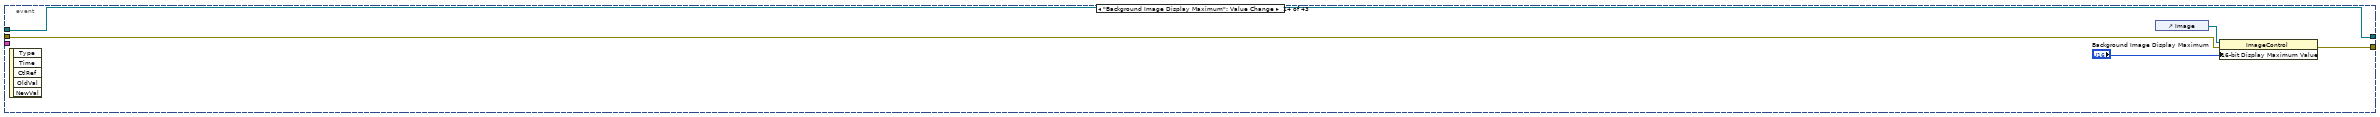
[diagram p14: hidden frame]
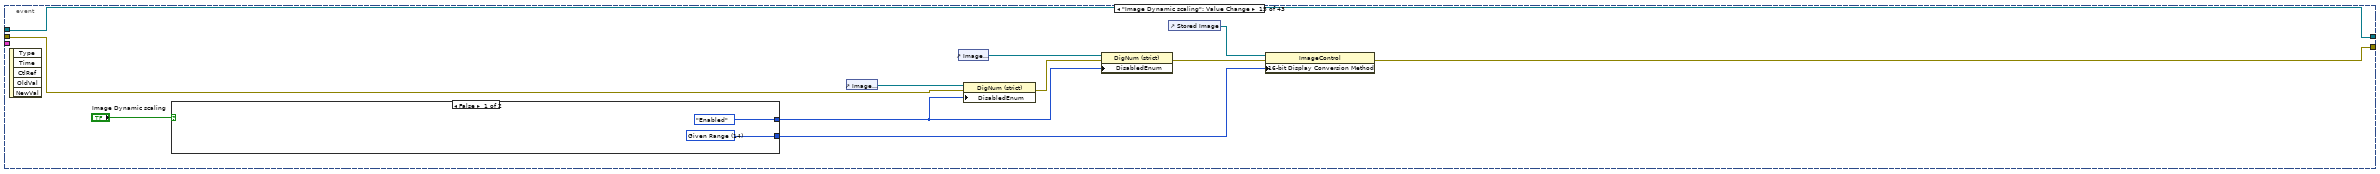
[diagram p15: hidden frame]
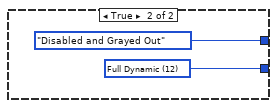
[diagram p16: hidden frame]
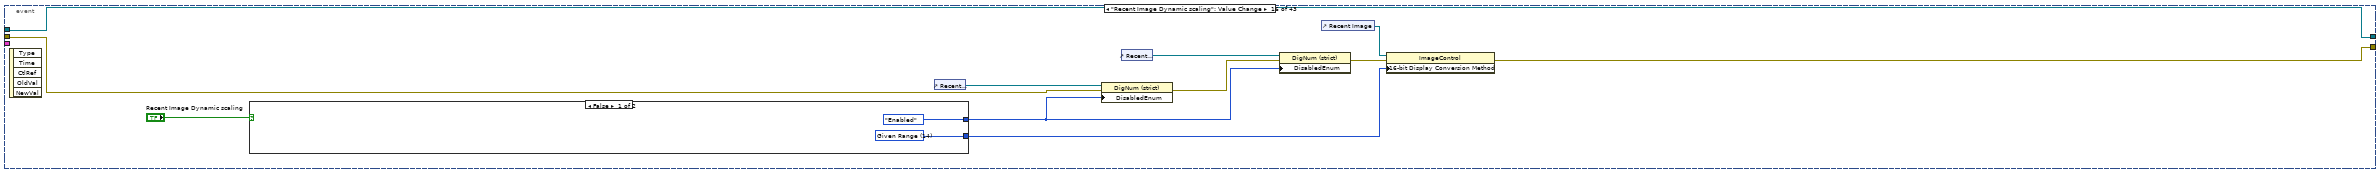
[diagram p17: hidden frame]
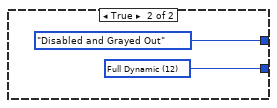
[diagram p18: hidden frame]
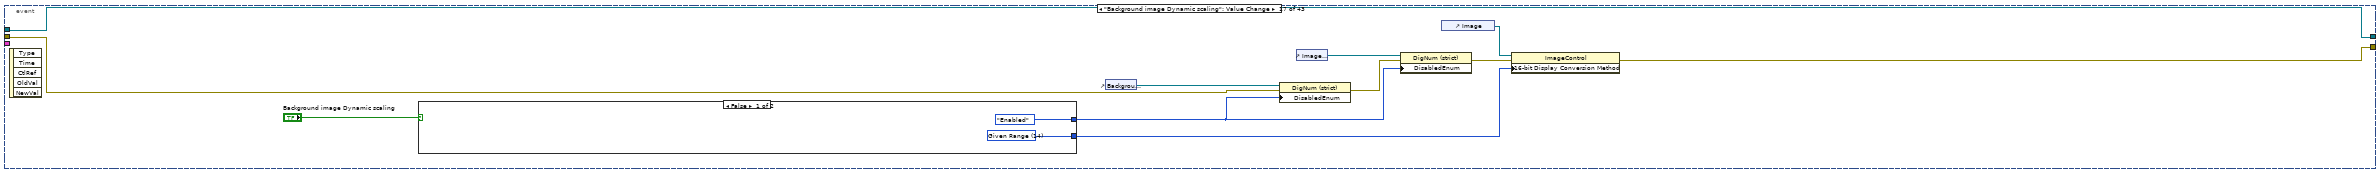
[diagram p19: hidden frame]
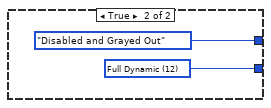
[diagram p20: hidden frame]
diagram:
  w44 = T45 {"current counter totals"=refnum, "Initialize DDS Boxes"=refnum, "Array of DDS Boxes"=refnum, "Error LED"=refnum, "Experiment is Running"=refnum, "DDS Initialized"=refnum, "Run Experiment"=refnum, "Quit Program"=refnum, "Histogram of ROI Sum over All Images for last ROI"=refnum, "Counters Chart"=refnum, "Image Array for whole experiment"=refnum, "Counter Refnums"={"Counter Data Refnum"=refnum, "Counters Chart 3 Refnum"=refnum, "Counters Chart Refnum"=refnum, "current counter totals Refnum"=refnum, "Counters Chart 2 Refnum"=refnum, "Counters Chart 4 Refnum"=refnum}, "Stop/Pause refnum cluster"={"stop"=refnum, "Pause after Measurement"=refnum, "Paused"=refnum, "Pause after Iteration"=refnum}, "Image Array for most recent measurement"=refnum, "Iteration Graph"=refnum, "PI Piezo Status"=refnum, "Measurement Chart ref"=refnum}  # GUI refnum cluster
  w50 = T47 3 items=["no dialog", "OK message", "continue or stop message", "OK message + warnings", "continue/stop + warnings"] ("type of dialog (OK msg:1)")
  w4 = errorcluster {"status"=FALSE, "code"=0, "source"=""}  # Clear Errors
  n1 = call "set_frequency.vi"() -> ()  [unwired: 11 in, 1 out]
  n2 = control-ref of="Pause after Measurement"() -> (w22:refnum<vi>)
  n3 = control-ref of="current counter totals"() -> (w28:refnum<vi>)
  n4 = control-ref of="Pause after Iteration"() -> (w16:refnum<vi>)
  n5 = control-ref of="Counters Chart 3"() -> (w26:refnum<vi>)
  n6 = control-ref of="Counters Chart"() -> (w27:refnum<vi>)
  n7 = control-ref of="Counters Chart 2"() -> (w29:refnum<vi>)
  n8 = control-ref of="Counters Chart 4"() -> (w30:refnum<vi>)
  n9 = control-ref of="counter data"() -> (w25:refnum<vi>)
  n10 = control-ref of="stop"() -> (w21:refnum<vi>)
  n11 = control-ref of="Paused?"() -> (w23:refnum<vi>)
  n12 = control-ref of="Histogram of ROI Sum over All Images for last ROI"() -> (w36:refnum<vi>)
  n13 = control-ref of="Image Array for most recent measurement"() -> (w18:refnum<vi>)
  n14 = control-ref of="Image Array for whole experiment"() -> (w35:refnum<vi>)
  n15 = Bundle By Name(cluster=T44 {"Counter Data Refnum"=refnum, "Counters Chart 3 Refnum"=refnum, "Counters Chart Refnum"=refnum, "current counter totals Refnum"=refnum, "Counters Chart 2 Refnum"=refnum, "Counters Chart 4 Refnum"=refnum} ("Counter Refnums"), "Counter Data Refnum"=w25, "Counters Chart 3 Refnum"=w26, "Counters Chart Refnum"=w27, "current counter totals Refnum"=w28, "Counters Chart 2 Refnum"=w29, "Counters Chart 4 Refnum"=w30) -> (w24:T44)
  n16 = Bundle By Name(cluster=T43 {"stop"=refnum, "Pause after Measurement"=refnum, "Paused"=refnum, "Pause after Iteration"=refnum} ("Stop/Pause refnum cluster"), "stop"=w21, "Pause after Measurement"=w22, "Paused"=w23, "Pause after Iteration"=w16) -> (w19:T43)
  n17 = shared-variable "My Computer\\Experiment_network_vars.lvlib\\Stop"(FALSE ("Stop"), error in=w4) -> (error out=w3:errorcluster)
  n18 = control-ref of="Experiment is Running"() -> (w40:refnum<vi>)
  n19 = control-ref of="current counter totals"() -> (w43:refnum<vi>)
  n20 = control-ref of="Measurement Chart"() -> (w7:refnum<vi>)
  n21 = control-ref of="Iteration Graph"() -> (w33:refnum<vi>)
  n22 = control-ref of="Initialize DDS Boxes"() -> (w42:refnum<vi>)
  n23 = control-ref of="Counters Chart"() -> (w34:refnum<vi>)
  n24 = control-ref of="Array of DDS Boxes"() -> (w17:refnum<vi>)
  n25 = control-ref of="Run Experiment"() -> (w38:refnum<vi>)
  n26 = control-ref of="DDS Initialized"() -> (w39:refnum<vi>)
  n27 = control-ref of="PI Piezo Status"() -> (w9:refnum<vi>)
  n28 = control-ref of="Quit Program"() -> (w37:refnum<vi>)
  n29 = control-ref of="Error LED"() -> (w41:refnum<vi>)
  n30 = Bundle By Name(cluster=w44, "current counter totals"=w43, "Initialize DDS Boxes"=w42, "Array of DDS Boxes"=w17, "Error LED"=w41, "Experiment is Running"=w40, "DDS Initialized"=w39, "Run Experiment"=w38, "Quit Program"=w37, "Histogram of ROI Sum over All Images for last ROI"=w36, "Counters Chart"=w34, "Image Array for whole experiment"=w35, "Iteration Graph"=w33, "Counter Refnums"=w24, "Stop/Pause refnum cluster"=w19, "Image Array for most recent measurement"=w18, "PI Piezo Status"=w9, "Measurement Chart ref"=w7) -> (w32:T45)
  n31 = shared-variable "My Computer\\Experiment_network_vars.lvlib\\Log"("Log", error in=w3) -> (error out=w1:errorcluster)
  n32 = call "setup_gui.vi"("Enum"=T46."reset", "GUI refnum cluster"=w32, "error in (no error)"=w1) -> ("error out"=w6:errorcluster)  [unwired: 12 in]
  n33 = call "handle_errors.vi"("error in (no error)"=w6) -> ("error out"=w45:errorcluster)  [unwired: 10 in]
  n34 = while {
    tunnel: w45 -> [w57]
    tunnel: [w52] -> w10
    shift-right: [w55] -> w12
    shift-left: refnum<class "Hamamatsu_C9100-13.lvclass"> refnum ("Hamamatsu_C9100-13.lvclass") -> [w56]
    tunnel: w32 -> [w54]
    stop <- w51 stop-if-true
    (unwired) 200
    n35 = event shown="[1] \"Run Experiment\": Value Change" {
      selector: _ -> [_ _ _ _ _ _ _ _ _ _ _ _ _ _ _ _ _ _ _ _ _ _ _ _ _ _ _ _ _ _ _ _ _ _ _ _ _ _ _ _ _ _ _]
      dyn-events: _ -> [_ _ _ _ _ _ _ _ _ _ _ _ _ _ _ _ _ _ _ _ _ _ _ _ _ _ _ _ _ _ _ _ _ _ _ _ _ _ _ _ _ _ _]
      timeout: _ -> [_ _ _ _ _ _ _ _ _ _ _ _ _ _ _ _ _ _ _ _ _ _ _ _ _ _ _ _ _ _ _ _ _ _ _ _ _ _ _ _ _ _ _]
      tunnel: w57 -> [w62 w93 w137 w146 w164 w172 w179 w191 w196 w211 w216 w222 w226 w230 w235 w252 w270 w281 w287 w291 w295 w300 w304 w312 w318 w328 w359 w379 w386 w391 w398 w415 w429 w445 w460 w485 w496 w507 w517 w540 w582 w587 w592]
      tunnel: [w58 w92 w136 w145 w169 w171 w178 w190 w199 w210 w215 w221 w225 w231 w234 w251 w269 w280 w286 w290 w294 w297 w305 w311 w314 w333 w361 w380 w388 w392 w404 w411 w435 w448 w463 w485 w497 w508 w513 w531 w581 w586 w591] -> w53
      tunnel: w56 -> [w61 w94 w138 w158 w159 w170 w177 w188 w204 w212 w213 w219 w223 w228 w233 w250 w263 w278 w284 w289 w292 w296 w301 w306 w319 w334 w362 w382 w389 w394 w405 w414 w436 w446 w461 w489 w498 w510 w511 w529 w584 w588 w590]
      tunnel: [w60 w96 w138 w158 w159 w170 w177 w188 w204 w212 w213 w219 w223 w228 w233 w250 w263 w278 w284 w289 w292 w296 w301 w306 w319 w334 w362 w382 w389 w394 w405 w414 w436 w446 w461 w489 w498 w510 w511 w529 w584 w588 w590] -> w55
      tunnel: w54 -> [_ w102 _ _ _ _ _ _ _ _ _ _ _ _ _ _ _ _ _ _ _ _ _ _ _ _ _ _ _ _ _ _ _ _ _ _ _ _ _ _ _ _ _]
      event Timeout {
        n36 = event-data() -> ()  [unwired: 1 in, 2 out]
        n37 = call-dynamic "Read Camera Temperature.vi"("error in (no error)"=w62, "Hamamatsu_C9100-13 in"=w61) -> ("error out"=w58:errorcluster, "Camera Temperature"=→"Camera Temperature":dbl, "Hamamatsu_C9100-13 out"=w60:refnum<class "Hamamatsu_C9100-13.lvclass">)  [unwired: 7 in]
      }
      event "Run Experiment": Value Change {
        w71 = T51 {"Variable Settings"={"Measurements per Iteration"=0, "Local Data Path"=path "", "Experiment description suffix for filename (no spaces please)"="", "Network Data Path"=path "", "Copy data to network"=FALSE, "Measurement Timeout (ms)"=0, "Independent Variables"=[], "Dependent Variables"=[], "Run Test Mode"=FALSE}, "HSDIO Settings"={"Enable HSDIO Pulses"=FALSE, "Resource Name"="", "Clock Rate"=0.0, "Array of Script Triggers"=[], "Channels Control"=[], "Pulse Generation Script"="", "Start Trigger"={"Wait for start trigger?"=FALSE, "source (PFI 0)"="", "edge (rising)"=0}, "Hardware alignment quantum\n(in samples)"=0, "Inital State"="", "Idle State"="", "Active Channels"="", "Array of Waveforms"=[]}, "DAQmx Pulse Settings"={"Enable DAQmx Pulses"=FALSE, "DAQmx Physical Channels"="", "Clock Rate"=0.0, "units/sec (ms=1000)"=0.0, "Start Trigger"={"Wait for start trigger?"=FALSE, "source"="", "edge"=0}, "Timing Sequence Control"=[]}, "DDS Settings"={"Enable DDS"=FALSE, "Array of DDS Boxes"=[]}, "Camera settings"={"Analog Gain (0-5)"=0, "Exposure Time"=0.0, "EM Gain (0-255)"=0, "Trigger Polarity"="", "External Trigger Mode"="", "Scan Speed"="", "External Trigger Source"="", "Scan Mode"="", "Super Pixel Binning\n(if enabled in Scan Mode)"="", "Camera Sub-array acquisition region\n(if enabled in scan mode)"={"Left"=0, "Top"=0, "Width"=0, "Height"=0}, "Use camera?"=FALSE, "# image buffers"=0, "shots per measurement"=0, "Force images to U16"=FALSE, "Low Light Sensitivity"="", "cooling"="", "fan"="", "Frame Grabber acquisition region"={"Left"=0, "Top"=0, "Right"=0, "Bottom"=0}}, "Counter Settings"={"Enable Counters"=FALSE, "Array of Counter Settings"=[]}, "Filter Cluster"={"Counter Filter thresholds"=[], "Data Filters\nROI Minimum Thresholds"=[]}, "Analog Output Parameters"={"Enable Analog Out?"=FALSE, "Physical Channel"="", "Minimum Value"=0.0, "Maximum Value"=0.0, "Samples per second"=0.0, "Total AO Time (seconds)"=0.0, "Start Trigger"={"Wait for start trigger?"=FALSE, "source"="", "edge"=0}, "Analog Output Waveforms (channel, time)"=[]}, "Notes"="", "HP83623A Generator Settings Array"=[], "Iteration Graph Settings"={"Plot Regions"="", "Plot Shots"=""}, "PI Piezo Settings"={"Enable"=FALSE, "Array of Piezo Controllers"=[]}, "Andor settings"={"Andor Path"=path "", "Copy any Andor files"=FALSE, "Wait time before copying Andor files (ms)"=0}, "Measurement Chart Settings"={"Which regions to plot (comma separated)"="", "Which shot to plot"=0}, "HP8662A Synthesized Signal Generator Array"=[], "HP83712B Synthesized CW Generator Array"=[], "TTL input"={"Enable"=FALSE, "lines"=""}}  # all settings
        n38 = event-data() -> ()  [unwired: 1 in, 5 out]
        n39 = control-ref of="Average of All Images from experiment"() -> (w86:refnum<vi>)
        n40 = control-ref of="Backgound Subtracted Average Image"() -> (w89:refnum<vi>)
        n41 = control-ref of="Background Image"() -> (w88:refnum<vi>)
        n42 = control-ref of="Recent Image"() -> (w84:refnum<vi>)
        n43 = control-ref of="Stored Image"() -> (w85:refnum<vi>)
        n44 = control-ref of="Image"() -> (w87:refnum<vi>)
        n45 = Build Array(w84, w85, w86, w88, w87, w89) -> (w83:refnum<vi>[])
        n46 = Bundle By Name(cluster=w71, "Variable Settings"="Variable Settings", "HSDIO Settings"="HSDIO Settings", "DAQmx Pulse Settings"="DAQmx Pulse Settings", "DDS Settings"="DDS Settings", "Camera settings"="Hamamatsu Setup", "Counter Settings"="Counter Settings", "Filter Cluster"="Filter Cluster", "Analog Output Parameters"="Analog Output Parameters", "Notes"="Notes", "HP83623A Generator Settings Array"="HP83623A Generator Settings Array", "Iteration Graph Settings"="Iteration Graph Settings", "PI Piezo Settings"="PI Piezo Settings", "Andor settings"="Andor setup", "Measurement Chart Settings"="Measurement Chart Settings", "HP8662A Synthesized Signal Generator Array"="HP8662A Synthesized Signal Generator Array", "TTL input"="TTL input", "HP83712B Synthesized CW Generator Array"="HP83712B Synthesized Signal Generator Array") -> (w81:T51)
        n47 = control-ref of="Camera Temperature"() -> (w101:refnum<vi>)
        n48 = control-ref of="Variable Settings"() -> (w82:refnum<vi>)
        n49 = control-ref of="HSDIO Status"() -> (w100:refnum<vi>)
        n50 = control-ref of="Notes"() -> (w91:refnum<vi>)
        n51 = call "run_experiment.vi"("GUI refnum cluster"=w102, "all settings"=w81, "Variable Settings Refnum"=w82, "error in (no error)"=w93, "Image Display Refnum Array"=w83, "Camera Temperature Refnum"=w101, "HSDIO Status Refnum"=w100, "# intervals (mutli-shot)"="# intervals (mutli-shot)", "Notes Refnum"=w91, "Hamamatsu_C9100-13.lvclass"=w94) -> ("Array of ROI sums"=→"Array of ROI sums":dbl[][][][], "Image Array for whole experiment"=→"Image Array for whole experiment":T30[][][], "Histogram of ROI Sum over All Images for last ROI"=→"Histogram of ROI Sum over All Images for last ROI":T32, "Average of All Images from experiment"=→"Average of All Images from experiment":T30, "Camera out"=w96:refnum<class "Hamamatsu_C9100-13.lvclass">, "error out"=w92:errorcluster)  [unwired: 12 in]
      }
      event "Load Settings": Value Change {
        w127 = T51 {"Variable Settings"={"Measurements per Iteration"=0, "Local Data Path"=path "", "Experiment description suffix for filename (no spaces please)"="", "Network Data Path"=path "", "Copy data to network"=FALSE, "Measurement Timeout (ms)"=0, "Independent Variables"=[], "Dependent Variables"=[], "Run Test Mode"=FALSE}, "HSDIO Settings"={"Enable HSDIO Pulses"=FALSE, "Resource Name"="", "Clock Rate"=0.0, "Array of Script Triggers"=[], "Channels Control"=[], "Pulse Generation Script"="", "Start Trigger"={"Wait for start trigger?"=FALSE, "source (PFI 0)"="", "edge (rising)"=0}, "Hardware alignment quantum\n(in samples)"=0, "Inital State"="", "Idle State"="", "Active Channels"="", "Array of Waveforms"=[]}, "DAQmx Pulse Settings"={"Enable DAQmx Pulses"=FALSE, "DAQmx Physical Channels"="", "Clock Rate"=0.0, "units/sec (ms=1000)"=0.0, "Start Trigger"={"Wait for start trigger?"=FALSE, "source"="", "edge"=0}, "Timing Sequence Control"=[]}, "DDS Settings"={"Enable DDS"=FALSE, "Array of DDS Boxes"=[]}, "Camera settings"={"Analog Gain (0-5)"=0, "Exposure Time"=0.0, "EM Gain (0-255)"=0, "Trigger Polarity"="", "External Trigger Mode"="", "Scan Speed"="", "External Trigger Source"="", "Scan Mode"="", "Super Pixel Binning\n(if enabled in Scan Mode)"="", "Camera Sub-array acquisition region\n(if enabled in scan mode)"={"Left"=0, "Top"=0, "Width"=0, "Height"=0}, "Use camera?"=FALSE, "# image buffers"=0, "shots per measurement"=0, "Force images to U16"=FALSE, "Low Light Sensitivity"="", "cooling"="", "fan"="", "Frame Grabber acquisition region"={"Left"=0, "Top"=0, "Right"=0, "Bottom"=0}}, "Counter Settings"={"Enable Counters"=FALSE, "Array of Counter Settings"=[]}, "Filter Cluster"={"Counter Filter thresholds"=[], "Data Filters\nROI Minimum Thresholds"=[]}, "Analog Output Parameters"={"Enable Analog Out?"=FALSE, "Physical Channel"="", "Minimum Value"=0.0, "Maximum Value"=0.0, "Samples per second"=0.0, "Total AO Time (seconds)"=0.0, "Start Trigger"={"Wait for start trigger?"=FALSE, "source"="", "edge"=0}, "Analog Output Waveforms (channel, time)"=[]}, "Notes"="", "HP83623A Generator Settings Array"=[], "Iteration Graph Settings"={"Plot Regions"="", "Plot Shots"=""}, "PI Piezo Settings"={"Enable"=FALSE, "Array of Piezo Controllers"=[]}, "Andor settings"={"Andor Path"=path "", "Copy any Andor files"=FALSE, "Wait time before copying Andor files (ms)"=0}, "Measurement Chart Settings"={"Which regions to plot (comma separated)"="", "Which shot to plot"=0}, "HP8662A Synthesized Signal Generator Array"=[], "HP83712B Synthesized CW Generator Array"=[], "TTL input"={"Enable"=FALSE, "lines"=""}}  # all settings
        n52 = event-data() -> ()  [unwired: 1 in, 5 out]
        n53 = local read "HP83712B Synthesized Signal Generator Array"() -> (w106:T25)
        n54 = local read "HP8662A Synthesized Signal Generator Array"() -> (w108:T25)
        n55 = local read "HP83623A Generator Settings Array"() -> (w114:T27)
        n56 = local read "Analog Output Parameters"() -> (w129:T36)
        n57 = local read "DAQmx Pulse Settings"() -> (w134:T13)
        n58 = local read "Hamamatsu Setup"() -> (w132:T31)
        n59 = local read "Counter Settings"() -> (w131:T34)
        n60 = local read "Variable Settings"() -> (w126:T3)
        n61 = local read "PI Piezo Settings"() -> (w112:T37)
        n62 = local read "HSDIO Settings"() -> (w135:T4)
        n63 = local read "DDS Settings"() -> (w133:T15)
        n64 = local read "Filter Cluster"() -> (w130:T35)
        n65 = local read "Andor setup"() -> (w110:T29)
        n66 = local read "TTL input"() -> (w104:T42)
        n67 = local read "Notes"() -> (w128:string)
        n68 = Bundle By Name(cluster=w127, "Variable Settings"=w126, "HSDIO Settings"=w135, "DAQmx Pulse Settings"=w134, "DDS Settings"=w133, "Camera settings"=w132, "Counter Settings"=w131, "Filter Cluster"=w130, "Analog Output Parameters"=w129, "Notes"=w128, "HP83623A Generator Settings Array"=w114, "PI Piezo Settings"=w112, "Andor settings"=w110, "HP8662A Synthesized Signal Generator Array"=w108, "HP83712B Synthesized CW Generator Array"=w106, "TTL input"=w104) -> (w125:T51)
        n69 = call "load_settings.vi"("error in"=w137, "all settings (in)"=w125) -> ("error out"=w136:errorcluster, "all settings"=w115:T51)  [unwired: 8 in]
        n70 = Unbundle By Name(w115) -> ("Variable Settings"=w124:T3, "HSDIO Settings"=w116:T4, "DAQmx Pulse Settings"=w117:T13, "DDS Settings"=w118:T15, "Camera settings"=w119:T31, "Counter Settings"=w120:T34, "Filter Cluster"=w121:T35, "Analog Output Parameters"=w122:T36, "Notes"=w123:string, "HP83623A Generator Settings Array"=w113:T27, "PI Piezo Settings"=w111:T37, "Andor settings"=w109:T29, "HP8662A Synthesized Signal Generator Array"=w107:T25, "HP83712B Synthesized CW Generator Array"=w105:T25, "TTL input"=w103:T42)
        n71 = local write "Notes"(w123) -> ()
        n72 = local write "Variable Settings"(w124) -> ()
        n73 = local write "HSDIO Settings"(w116) -> ()
        n74 = local write "DAQmx Pulse Settings"(w117) -> ()
        n75 = local write "DDS Settings"(w118) -> ()
        n76 = local write "Counter Settings"(w120) -> ()
        n77 = local write "Filter Cluster"(w121) -> ()
        n78 = local write "Analog Output Parameters"(w122) -> ()
        n79 = local write "HP83623A Generator Settings Array"(w113) -> ()
        n80 = local write "Hamamatsu Setup"(w119) -> ()
        n81 = local write "PI Piezo Settings"(w111) -> ()
        n82 = local write "Andor setup"(w109) -> ()
        n83 = local write "HP8662A Synthesized Signal Generator Array"(w107) -> ()
        n84 = local write "HP83712B Synthesized Signal Generator Array"(w105) -> ()
        n85 = local write "TTL input"(w103) -> ()
      }
      event "Save Settings": Value Change {
        w149 = T51 {"Variable Settings"={"Measurements per Iteration"=0, "Local Data Path"=path "", "Experiment description suffix for filename (no spaces please)"="", "Network Data Path"=path "", "Copy data to network"=FALSE, "Measurement Timeout (ms)"=0, "Independent Variables"=[], "Dependent Variables"=[], "Run Test Mode"=FALSE}, "HSDIO Settings"={"Enable HSDIO Pulses"=FALSE, "Resource Name"="", "Clock Rate"=0.0, "Array of Script Triggers"=[], "Channels Control"=[], "Pulse Generation Script"="", "Start Trigger"={"Wait for start trigger?"=FALSE, "source (PFI 0)"="", "edge (rising)"=0}, "Hardware alignment quantum\n(in samples)"=0, "Inital State"="", "Idle State"="", "Active Channels"="", "Array of Waveforms"=[]}, "DAQmx Pulse Settings"={"Enable DAQmx Pulses"=FALSE, "DAQmx Physical Channels"="", "Clock Rate"=0.0, "units/sec (ms=1000)"=0.0, "Start Trigger"={"Wait for start trigger?"=FALSE, "source"="", "edge"=0}, "Timing Sequence Control"=[]}, "DDS Settings"={"Enable DDS"=FALSE, "Array of DDS Boxes"=[]}, "Camera settings"={"Analog Gain (0-5)"=0, "Exposure Time"=0.0, "EM Gain (0-255)"=0, "Trigger Polarity"="", "External Trigger Mode"="", "Scan Speed"="", "External Trigger Source"="", "Scan Mode"="", "Super Pixel Binning\n(if enabled in Scan Mode)"="", "Camera Sub-array acquisition region\n(if enabled in scan mode)"={"Left"=0, "Top"=0, "Width"=0, "Height"=0}, "Use camera?"=FALSE, "# image buffers"=0, "shots per measurement"=0, "Force images to U16"=FALSE, "Low Light Sensitivity"="", "cooling"="", "fan"="", "Frame Grabber acquisition region"={"Left"=0, "Top"=0, "Right"=0, "Bottom"=0}}, "Counter Settings"={"Enable Counters"=FALSE, "Array of Counter Settings"=[]}, "Filter Cluster"={"Counter Filter thresholds"=[], "Data Filters\nROI Minimum Thresholds"=[]}, "Analog Output Parameters"={"Enable Analog Out?"=FALSE, "Physical Channel"="", "Minimum Value"=0.0, "Maximum Value"=0.0, "Samples per second"=0.0, "Total AO Time (seconds)"=0.0, "Start Trigger"={"Wait for start trigger?"=FALSE, "source"="", "edge"=0}, "Analog Output Waveforms (channel, time)"=[]}, "Notes"="", "HP83623A Generator Settings Array"=[], "Iteration Graph Settings"={"Plot Regions"="", "Plot Shots"=""}, "PI Piezo Settings"={"Enable"=FALSE, "Array of Piezo Controllers"=[]}, "Andor settings"={"Andor Path"=path "", "Copy any Andor files"=FALSE, "Wait time before copying Andor files (ms)"=0}, "Measurement Chart Settings"={"Which regions to plot (comma separated)"="", "Which shot to plot"=0}, "HP8662A Synthesized Signal Generator Array"=[], "HP83712B Synthesized CW Generator Array"=[], "TTL input"={"Enable"=FALSE, "lines"=""}}  # all settings
        n86 = event-data() -> ()  [unwired: 1 in, 5 out]
        n87 = local read "HP83712B Synthesized Signal Generator Array"() -> (w139:T25)
        n88 = local read "HP8662A Synthesized Signal Generator Array"() -> (w141:T25)
        n89 = local read "HP83623A Generator Settings Array"() -> (w144:T27)
        n90 = local read "Analog Output Parameters"() -> (w151:T36)
        n91 = local read "DAQmx Pulse Settings"() -> (w156:T13)
        n92 = local read "Hamamatsu Setup"() -> (w154:T31)
        n93 = local read "Counter Settings"() -> (w153:T34)
        n94 = local read "Variable Settings"() -> (w148:T3)
        n95 = local read "PI Piezo Settings"() -> (w143:T37)
        n96 = local read "HSDIO Settings"() -> (w157:T4)
        n97 = local read "DDS Settings"() -> (w155:T15)
        n98 = local read "Filter Cluster"() -> (w152:T35)
        n99 = local read "Andor setup"() -> (w142:T29)
        n100 = local read "TTL input"() -> (w140:T42)
        n101 = local read "Notes"() -> (w150:string)
        n102 = Bundle By Name(cluster=w149, "Variable Settings"=w148, "HSDIO Settings"=w157, "DAQmx Pulse Settings"=w156, "DDS Settings"=w155, "Camera settings"=w154, "Counter Settings"=w153, "Filter Cluster"=w152, "Analog Output Parameters"=w151, "Notes"=w150, "HP83623A Generator Settings Array"=w144, "PI Piezo Settings"=w143, "Andor settings"=w142, "HP8662A Synthesized Signal Generator Array"=w141, "HP83712B Synthesized CW Generator Array"=w139, "TTL input"=w140) -> (w147:T51)
        n103 = call "manual_save_settings.vi"("error in"=w146, "all settings"=w147) -> ("error out"=w145:errorcluster)  [unwired: 9 in]
      }
      event "DAQmx Pulse Actions.Load Waveform from File": Value Change {
        n104 = event-data() -> ()  [unwired: 1 in, 5 out]
        n105 = property on="Timing Sequence Control" class="Tbl (strict)"(error in=w164) -> (error out=w165:errorcluster, "Value"=w168:string[][])  [unwired: 1 in, 1 out]
        n106 = Delete From Array(array=w168, length=3, index (col)=0 ("disabled index (col)")) -> (deleted portion=w163:string[][])  [unwired: 1 in, 1 out]
        n107 = call-poly <vilib>:"Read From Spreadsheet File.vi"() -> ("all rows"=w161:string[][])  [unwired: 7 in, 4 out]
        n108 = Insert Into Array(array=w163, index (col)=3 ("disabled index (col)"), new element=w161) -> (w160:string[][])  [unwired: 1 in]
        n109 = property on="Timing Sequence Control" class="Tbl (strict)"(error in=w165, "Value"=w160) -> (error out=w169:errorcluster)  [unwired: 1 in, 1 out]
      }
      event "DAQmx Pulse Actions.Save Waveform to File": Value Change {
        n110 = event-data() -> ()  [unwired: 1 in, 5 out]
        n111 = property on="Timing Sequence Control" class="Tbl (strict)"(error in=w172) -> (error out=w171:errorcluster, "Value"=w176:string[][])  [unwired: 1 in, 1 out]
        n112 = Delete From Array(array=w176, length=3, index (col)=0 ("disabled index (col)")) -> (array with subset deleted=w173:string[][])  [unwired: 1 in, 1 out]
        n113 = call-poly <vilib>:"Write To Spreadsheet File.vi"("2D data"=w173) -> ()  [unwired: 7 in, 1 out]
      }
      event "DAQmx Pulse Actions.Load Channels from File": Value Change {
        n114 = event-data() -> ()  [unwired: 1 in, 5 out]
        n115 = property on="Timing Sequence Control" class="Tbl (strict)"(error in=w179) -> (error out=w182:errorcluster, "Value"=w187:string[][])  [unwired: 1 in, 1 out]
        n116 = Delete From Array(array=w187, length=3, index (col)=0 ("disabled index (col)")) -> (array with subset deleted=w181:string[][])  [unwired: 1 in, 1 out]
        n117 = call-poly <vilib>:"Read From Spreadsheet File.vi"() -> ("all rows"=w184:string[][])  [unwired: 7 in, 4 out]
        n118 = Insert Into Array(array=w181, index (col)=0 ("disabled index (col)"), new element=w184) -> (w183:string[][])  [unwired: 1 in]
        n119 = property on="Timing Sequence Control" class="Tbl (strict)"(error in=w182, "Value"=w183) -> (error out=w178:errorcluster)  [unwired: 1 in, 1 out]
      }
      event "DAQmx Pulse Actions.Save Channels to File": Value Change {
        n120 = event-data() -> ()  [unwired: 1 in, 5 out]
        n121 = property on="Timing Sequence Control" class="Tbl (strict)"(error in=w191) -> (error out=w190:errorcluster, "Value"=w194:string[][])  [unwired: 1 in, 1 out]
        n122 = Delete From Array(array=w194, length=3, index (col)=0 ("disabled index (col)")) -> (deleted portion=w189:string[][])  [unwired: 1 in, 1 out]
        n123 = call-poly <vilib>:"Write To Spreadsheet File.vi"("2D data"=w189) -> ()  [unwired: 7 in, 1 out]
      }
      event "DDS Actions.Load DDS": Value Change {
        n124 = event-data() -> ()  [unwired: 1 in, 5 out]
        n125 = local read "Variable Settings"() -> (w203:T3)
        n126 = local read "DDS Settings"() -> (w197:T15)
        n127 = call "get_variable_start_values.vi"("error in (no error)"=w196, "Variable Settings"=w203) -> ("error out"=w195:errorcluster, "all variable names"=w201:string[], "all variable values (min or calculated)"=w202:dbl[])  [unwired: 6 in, 1 out]
        n128 = call "DDS update.vi"("error in (no error)"=w195, 9:w201, 10:w202, "DDS.lvclass (in)"=w197) -> ("error out"=w200:errorcluster)  [unwired: 6 in, 1 out]
        n129 = property on="Load DDS" class="Bool (strict)"(error in=w200, "Value"=FALSE ("Load DDS")) -> (error out=w199:errorcluster)  [unwired: 1 in, 1 out]
      }
      event "Check DDS": Value Change {
        n130 = event-data() -> ()  [unwired: 1 in, 5 out]
        n131 = local read "DDS Settings"() -> (w206:T15)
        n132 = call "DDS_Check_Box.vi"("error in (no error)"=w211, "box #"="box #", "DDS Settings"=w206) -> ("error out"=w210:errorcluster, "CFR3"=→"CFR3":u8[][], "CFR2"=→"CFR2":u8[][], "CFR1"=→"CFR1":u8[][])  [unwired: 5 in]
      }
      event "Image Display Minimum": Value Change {
        n133 = event-data() -> ()  [unwired: 1 in, 5 out]
        n134 = control-ref of="Stored Image"() -> (w214:refnum<vi>)
        n135 = property class="ImageControl"(reference=w214, error in=w216, "16-bit Display Minimum Value"="Image Display Minimum") -> (error out=w215:errorcluster)  [unwired: 1 out]
      }
      event "Recent Image Display Minimum": Value Change {
        n136 = event-data() -> ()  [unwired: 1 in, 5 out]
        n137 = control-ref of="Recent Image"() -> (w220:refnum<vi>)
        n138 = property class="ImageControl"(reference=w220, error in=w222, "16-bit Display Minimum Value"="Recent Image Display Minimum") -> (error out=w221:errorcluster)  [unwired: 1 out]
      }
      event "Background Image Display Minimum": Value Change {
        n139 = event-data() -> ()  [unwired: 1 in, 5 out]
        n140 = control-ref of="Image"() -> (w224:refnum<vi>)
        n141 = property class="ImageControl"(reference=w224, error in=w226, "16-bit Display Minimum Value"="Background Image Display Minimum") -> (error out=w225:errorcluster)  [unwired: 1 out]
      }
      event "Background Image Display Maximum": Value Change {
        n142 = event-data() -> ()  [unwired: 1 in, 5 out]
        n143 = control-ref of="Image"() -> (w229:refnum<vi>)
        n144 = property class="ImageControl"(reference=w229, error in=w230, "16-bit Display Maximum Value"="Background Image Display Maximum") -> (error out=w231:errorcluster)  [unwired: 1 out]
      }
      event "Image Dynamic scaling": Value Change {
        n145 = event-data() -> ()  [unwired: 1 in, 5 out]
        n146 = case shown="False" "Image Dynamic scaling" {
          tunnel: [w245 w247] -> w243
          tunnel: [T48."Enabled" ("Disabled") T48."Disabled and Grayed Out" ("Disabled")] -> w236
          frame False {
            w245 = u32 14 items=["Default"=10, "Most Significant Bits"=11, "Full Dynamic"=12, "Downshift"=13, "Given Range"=14, "90% Dynamic"=15, "Given Percent Range"=16] ("16-bit Display Mapping:Conversion Method")
          }
          frame True {
            w247 = u32 12 items=["Default"=10, "Most Significant Bits"=11, "Full Dynamic"=12, "Downshift"=13, "Given Range"=14, "90% Dynamic"=15, "Given Percent Range"=16] ("16-bit Display Mapping:Conversion Method")
          }
        }
        n147 = control-ref of="Image Display Maximum"() -> (w239:refnum<vi>)
        n148 = control-ref of="Image Display Minimum"() -> (w241:refnum<vi>)
        n149 = property class="DigNum (strict)"(reference=w239, error in=w235, "DisabledEnum"=w236) -> (error out=w238:errorcluster)  [unwired: 1 out]
        n150 = property class="DigNum (strict)"(reference=w241, error in=w238, "DisabledEnum"=w236) -> (error out=w237:errorcluster)  [unwired: 1 out]
        n151 = control-ref of="Stored Image"() -> (w242:refnum<vi>)
        n152 = property class="ImageControl"(reference=w242, error in=w237, "16-bit Display Conversion Method"=w243) -> (error out=w234:errorcluster)  [unwired: 1 out]
      }
      event "Recent Image Dynamic scaling": Value Change {
        n153 = event-data() -> ()  [unwired: 1 in, 5 out]
        n154 = case shown="False" "Recent Image Dynamic scaling" {
          tunnel: [w260 w262] -> w258
          tunnel: [T48."Enabled" ("Disabled") T48."Disabled and Grayed Out" ("Disabled")] -> w253
          frame False {
            w260 = u32 14 items=["Default"=10, "Most Significant Bits"=11, "Full Dynamic"=12, "Downshift"=13, "Given Range"=14, "90% Dynamic"=15, "Given Percent Range"=16] ("16-bit Display Mapping:Conversion Method")
          }
          frame True {
            w262 = u32 12 items=["Default"=10, "Most Significant Bits"=11, "Full Dynamic"=12, "Downshift"=13, "Given Range"=14, "90% Dynamic"=15, "Given Percent Range"=16] ("16-bit Display Mapping:Conversion Method")
          }
        }
        n155 = control-ref of="Recent Image Display Maximum"() -> (w256:refnum<vi>)
        n156 = property class="DigNum (strict)"(reference=w256, error in=w252, "DisabledEnum"=w253) -> (error out=w255:errorcluster)  [unwired: 1 out]
        n157 = control-ref of="Recent Image Display Minimum"() -> (w257:refnum<vi>)
        n158 = property class="DigNum (strict)"(reference=w257, error in=w255, "DisabledEnum"=w253) -> (error out=w254:errorcluster)  [unwired: 1 out]
        n159 = control-ref of="Recent Image"() -> (w248:refnum<vi>)
        n160 = property class="ImageControl"(reference=w248, error in=w254, "16-bit Display Conversion Method"=w258) -> (error out=w251:errorcluster)  [unwired: 1 out]
      }
      event "Background image Dynamic scaling": Value Change {
        n161 = event-data() -> ()  [unwired: 1 in, 5 out]
        n162 = case shown="False" "Background image Dynamic scaling" {
          tunnel: [w275 w277] -> w272
          tunnel: [T48."Enabled" ("Disabled") T48."Disabled and Grayed Out" ("Disabled")] -> w266
          frame False {
            w275 = u32 14 items=["Default"=10, "Most Significant Bits"=11, "Full Dynamic"=12, "Downshift"=13, "Given Range"=14, "90% Dynamic"=15, "Given Percent Range"=16] ("16-bit Display Mapping:Conversion Method")
          }
          frame True {
            w277 = u32 12 items=["Default"=10, "Most Significant Bits"=11, "Full Dynamic"=12, "Downshift"=13, "Given Range"=14, "90% Dynamic"=15, "Given Percent Range"=16] ("16-bit Display Mapping:Conversion Method")
          }
        }
        n163 = control-ref of="Background Image Display Minimum"() -> (w271:refnum<vi>)
        n164 = property class="DigNum (strict)"(reference=w271, error in=w270, "DisabledEnum"=w266) -> (error out=w268:errorcluster)  [unwired: 1 out]
        n165 = control-ref of="Image Display Maximum"() -> (w265:refnum<vi>)
        n166 = property class="DigNum (strict)"(reference=w265, error in=w268, "DisabledEnum"=w266) -> (error out=w267:errorcluster)  [unwired: 1 out]
        n167 = control-ref of="Image"() -> (w264:refnum<vi>)
        n168 = property class="ImageControl"(reference=w264, error in=w267, "16-bit Display Conversion Method"=w272) -> (error out=w269:errorcluster)  [unwired: 1 out]
      }
      event "Image Display Maximum": Value Change {
        n169 = event-data() -> ()  [unwired: 1 in, 5 out]
        n170 = control-ref of="Stored Image"() -> (w279:refnum<vi>)
        n171 = property class="ImageControl"(reference=w279, error in=w281, "16-bit Display Maximum Value"="Image Display Maximum") -> (error out=w280:errorcluster)  [unwired: 1 out]
      }
      event "Recent Image Display Maximum": Value Change {
        n172 = event-data() -> ()  [unwired: 1 in, 5 out]
        n173 = control-ref of="Recent Image"() -> (w285:refnum<vi>)
        n174 = property class="ImageControl"(reference=w285, error in=w287, "16-bit Display Maximum Value"="Recent Image Display Maximum") -> (error out=w286:errorcluster)  [unwired: 1 out]
      }
      event "HSDIO Actions.Load Channels Control": Value Change {
        n175 = event-data() -> ()  [unwired: 1 in, 5 out]
        n176 = call-poly <vilib>:"Read From Spreadsheet File.vi"() -> ("all rows"=w288:string[][])  [unwired: 7 in, 4 out]
        n177 = property on="Pulse Generation Script" class="Str"(error in=w291, "Value"=w288) -> (error out=w290:errorcluster)  [unwired: 1 in, 1 out]
      }
      event "HSDIO Actions.Save Channels Control": Value Change {
        n178 = event-data() -> ()  [unwired: 1 in, 5 out]
        n179 = property on="Pulse Generation Script" class="Str"(error in=w295) -> (error out=w294:errorcluster, "Value"=w293:string)  [unwired: 1 in, 1 out]
        n180 = call-poly <vilib>:"Write To Spreadsheet File.vi"("2D data"=w293) -> ()  [unwired: 7 in, 1 out]
      }
      event "HSDIO Actions.Load Script": Value Change {
        n181 = event-data() -> ()  [unwired: 1 in, 5 out]
        n182 = Read from Text File(error in=w300) -> (text=w299:string, error out=w298:errorcluster)  [unwired: 3 in, 2 out]
        n183 = property on="Start Trigger" class="Clust (strict)"(error in=w298, "Value"=w299) -> (error out=w297:errorcluster)  [unwired: 1 in, 1 out]
      }
      event "HSDIO Actions.Save Script": Value Change {
        n184 = event-data() -> ()  [unwired: 1 in, 5 out]
        n185 = property on="Start Trigger" class="Clust (strict)"(error in=w304) -> (error out=w303:errorcluster, "Value"=w302:T52)  [unwired: 1 in, 1 out]
        n186 = Write to Text File(text=w302, error in=w303) -> (error out=w305:errorcluster)  [unwired: 2 in, 2 out]
      }
      event "HSDIO Actions.Open NI Script Editor": Value Change {
        n187 = event-data() -> ()  [unwired: 1 in, 5 out]
        n188 = local read "HSDIO Settings"() -> (w308:T4)
        n189 = Unbundle By Name(w308) -> ("Directory to look for waveform files"=w307:path)
        n190 = call <vilib>:"System Exec.vi"("wait until completion? (T)"=FALSE, "error in (no error)"=w312, "working directory"=w307, "command line"="\"C:\\Program Files\\National Instruments\\Script Editor\\ScriptEditor.exe\"") -> ("error out"=w311:errorcluster)  [unwired: 4 in, 3 out]
      }
      event "HSDIO Actions.Edit a Waveform": Value Change {
        n191 = event-data() -> ()  [unwired: 1 in, 5 out]
        n192 = property on="Edit a Waveform" class="Bool (strict)"(error in=w318, "Value"=FALSE) -> (error out=w315:errorcluster)  [unwired: 1 in, 1 out]
        n193 = local read "HSDIO Settings"() -> (w316:T4)
        n194 = in-place "Allow waveform dialog to update channels control" {
          in-place-border: w315 -> [w321]
          in-place-border: [w320] -> w314
          n195 = in-place-cluster #1(w316) -> ("Channels Control"=w323:string[][])
          n196 = call "edit_waveform.vi"("error in"=w321, "Channels Control"=w323) -> ("error out"=w320:errorcluster, "Channels out"=w322:string[][])  [unwired: 8 in]
          n197 = in-place-cluster #1("Channels Control"=w322) -> (w313:T4)
        }
        n198 = local write "HSDIO Settings"(w313) -> ()
      }
      event "Variable Actions.Load Independents": Value Change {
        n199 = event-data() -> ()  [unwired: 1 in, 5 out]
        n200 = call-poly <vilib>:"Read From Spreadsheet File.vi"() -> ("all rows"=w324:string[][])  [unwired: 7 in, 4 out]
        n201 = Delete From Array "Remove Header"(array=w324, length=1, index (row)=0 ("index")) -> (array with subset deleted=w325:string[][])  [unwired: 1 in, 1 out]
        n202 = for {
          shift-right: [w343] -> w330
          shift-left: w328 -> [w343]
          tunnel: w325 -> [w349] mode=indexing
          tunnel: [w351] -> w329 mode=indexing
          n203 = Index Array(array=w349, index #1=0 ("index"), index #2=1 ("index"), index #3=2 ("index"), index #4=3 ("index"), index #5=4 ("index")) -> (element #1=w342:string, element #2=w341:string, element #3=w340:string, element #4=w338:string, element #5=w336:string)
          n204 = Fract/Exp String To Number(string=w340) -> (number=w339:dbl)  [unwired: 3 in, 1 out]
          n205 = Fract/Exp String To Number(string=w338) -> (number=w337:dbl)  [unwired: 3 in, 1 out]
          n206 = Decimal String To Number(string=w336) -> (number=w335:i32)  [unwired: 2 in, 1 out]
          n207 = Bundle By Name(cluster=T49 {"Description"="", "Name (a,a0...a9)"="", "min"=0.0, "max"=0.0, "# steps"=0} ("Cluster"), "Description"=w342, "Name (a,a0...a9)"=w341, "min"=w339, "max"=w337, "# steps"=w335) -> (w351:T49)
        }
        n208 = property on="Independent Variables" class="Arr (strict)"(error in=w330, "Value"=w329) -> (error out=w331:errorcluster)  [unwired: 1 in, 1 out]
        n209 = property on="Load Independents" class="Bool (strict)"(error in=w331, "Value"=FALSE) -> (error out=w333:errorcluster)  [unwired: 1 in, 1 out]
      }
      event "Variable Actions.Load Dependents": Value Change {
        n210 = event-data() -> ()  [unwired: 1 in, 5 out]
        n211 = call-poly <vilib>:"Read From Spreadsheet File.vi"() -> ("all rows"=w353:string[][])  [unwired: 7 in, 4 out]
        n212 = Delete From Array "Remove Header"(array=w353, length=1, index (row)=0 ("index")) -> (array with subset deleted=w352:string[][])  [unwired: 1 in, 1 out]
        n213 = for {
          shift-right: [w368] -> w357
          shift-left: w359 -> [w368]
          tunnel: [w375] -> w358 mode=indexing
          tunnel: w352 -> [w373] mode=indexing
          n214 = Index Array(array=w373, index #1=0 ("index"), index #2=1 ("index"), index #3=2 ("index"), index #4=3 ("index")) -> (element #1=w367:string, element #2=w366:string, element #3=w365:string, element #4=w364:string)
          n215 = Fract/Exp String To Number(string=w364) -> (number=w363:dbl)  [unwired: 3 in, 1 out]
          n216 = Bundle By Name(cluster=T50 {"Description"="", "Name (a,a0...a9)"="", "Equation"="", "Result"=0.0} ("Cluster"), "Description"=w367, "Name (a,a0...a9)"=w366, "Equation"=w365, "Result"=w363) -> (w375:T50)
        }
        n217 = property on="Dependent Variables" class="Arr (strict)"(error in=w357, "Value"=w358) -> (error out=w356:errorcluster)  [unwired: 1 in, 1 out]
        n218 = property on="Load Dependents" class="Bool (strict)"(error in=w356, "Value"=FALSE) -> (error out=w361:errorcluster)  [unwired: 1 in, 1 out]
      }
      event "Variable Actions.Save Independents": Value Change {
        n219 = event-data() -> ()  [unwired: 1 in, 5 out]
        n220 = property on="Independent Variables" class="Arr (strict)"(error in=w379) -> (error out=w377:errorcluster, "Value"=w378:T53)  [unwired: 1 in, 1 out]
        n221 = call "save_variables_table.vi"("error in"=w377, "Variable Settings.Variables"=w378) -> ("error out"=w376:errorcluster)  [unwired: 9 in]
        n222 = property on="Return button to the unclicked position" class="Bool (strict)"(error in=w376, "Value"=FALSE) -> (error out=w380:errorcluster)  [unwired: 1 in, 1 out]
      }
      event "Variable Actions.Save Dependents": Value Change {
        n223 = event-data() -> ()  [unwired: 1 in, 5 out]
        n224 = property on="Dependent Variables" class="Arr (strict)"(error in=w386) -> (error out=w384:errorcluster, "Value"=w385:T54)  [unwired: 1 in, 1 out]
        n225 = call "save_parameters_table.vi"("error in"=w384, "Parameters"=w385) -> ("error out"=w383:errorcluster)  [unwired: 9 in]
        n226 = property on="Save Dependents" class="Bool (strict)"(error in=w383, "Value"=FALSE) -> (error out=w388:errorcluster)  [unwired: 1 in, 1 out]
      }
      event "Variable Actions.Clear Log": Value Change {
        n227 = event-data() -> ()  [unwired: 1 in, 5 out]
        n228 = call "clear_log.vi"("error in"=w391) -> ("error out"=w390:errorcluster)  [unwired: 10 in]
        n229 = property on="Clear Log" class="Bool (strict)"(error in=w390, "Value"=FALSE) -> (error out=w392:errorcluster)  [unwired: 1 in, 1 out]
      }
      event "Variable Actions.Evaluate Dependents": Value Change {
        n230 = event-data() -> ()  [unwired: 1 in, 5 out]
        n231 = local read "Variable Settings"() -> (w399:T3)
        n232 = call "get_variable_start_values.vi"("error in (no error)"=w398, "Variable Settings"=w399) -> ("error out"=w395:errorcluster, "dependent variable results"=w397:dbl[])  [unwired: 6 in, 2 out]
        n233 = property on="Dependent Variables" class="Arr (strict)"(error in=w395) -> (error out=w396:errorcluster, "Value"=w402:T54)  [unwired: 1 in, 1 out]
        n234 = for {
          tunnel: w397 -> [w408] mode=indexing
          tunnel: [w407] -> w401 mode=indexing
          tunnel: w402 -> [w406] mode=indexing
          n235 = Bundle By Name(cluster=w406, "Result"=w408) -> (w407:T50)
        }
        n236 = property on="Dependent Variables" class="Arr (strict)"(error in=w396, "Value"=w401) -> (error out=w400:errorcluster)  [unwired: 1 in, 1 out]
        n237 = property on="Evaluate Dependents" class="Bool (strict)"(error in=w400, "Value"=FALSE) -> (error out=w404:errorcluster)  [unwired: 1 in, 1 out]
      }
      event "DDS Actions.Initialize DDS Boxes": Value Change {
        n238 = event-data() -> ()  [unwired: 1 in, 5 out]
        n239 = local read "DDS Settings"() -> (w409:T15)
        n240 = Unbundle By Name(w409) -> ("Enable DDS"=w410:bool)
        n241 = case shown="True" w410 {
          tunnel: w415 -> [w416 w418]
          tunnel: [w416 w424] -> w412
          tunnel: w409 -> [_ w419]
          frame False {
          }
          frame True {
            n242 = local read "Variable Settings"() -> (w420:T3)
            n243 = call "get_variable_start_values.vi"("error in (no error)"=w418, "Variable Settings"=w420) -> ("error out"=w417:errorcluster, "all variable names"=w422:string[], "all variable values (min or calculated)"=w421:dbl[])  [unwired: 6 in, 1 out]
            n244 = call "DDS Startup.vi"("error in (no error)"=w417, "Variable Names"=w422, "Variable Values"=w421, "DDS Settings"=w419) -> ("error out"=w425:errorcluster)  [unwired: 7 in]
            n245 = property on="DDS Initialized" class="Bool (strict)"(error in=w425, "Value"=TRUE ("DDS Initialized")) -> (error out=w424:errorcluster)  [unwired: 1 in, 1 out]
          }
        }
        n246 = property on="Initialize DDS Boxes" class="Bool (strict)"(error in=w412, "Value"=FALSE ("DDS Initialized")) -> (error out=w411:errorcluster)  [unwired: 1 in, 1 out]
      }
      event "Load HP83623A Settings": Value Change {
        n247 = event-data() -> ()  [unwired: 1 in, 5 out]
        n248 = property on="return button to false" class="Bool (strict)"(error in=w429, "Value"=FALSE) -> (error out=w428:errorcluster)  [unwired: 1 in, 1 out]
        n249 = local read "Variable Settings"() -> (w433:T3)
        n250 = local read "HP83623A Generator Settings Array"() -> (w434:T27)
        n251 = call "get_variable_start_values.vi"("error in (no error)"=w428, "Variable Settings"=w433) -> ("error out"=w430:errorcluster, "all variable names"=w432:string[], "all variable values (min or calculated)"=w431:dbl[])  [unwired: 6 in, 1 out]
        n252 = for {
          shift-right: [w441] -> w435
          shift-left: w430 -> [w442]
          tunnel: w434 -> [w440] mode=indexing
          tunnel: w432 -> [w439]
          tunnel: w431 -> [w438]
          tunnel: [w437] -> w426 mode=indexing
          n253 = call "hp83623a Init and Update.vi"("error in (no error)"=w442, 9:w439, 10:w438, "hp83623a Settings (in)"=w440) -> ("error out"=w441:errorcluster, "hp83623a Settings"=w437:T28)  [unwired: 6 in]
        }
        n254 = local write "HP83623A Generator Settings Array"(w426) -> ()
      }
      event "Load HP8662A Settings": Value Change {
        n255 = event-data() -> ()  [unwired: 1 in, 5 out]
        n256 = property on="return button to false" class="Bool (strict)"(error in=w445, "Value"=FALSE) -> (error out=w444:errorcluster)  [unwired: 1 in, 1 out]
        n257 = local read "HP8662A Synthesized Signal Generator Array"() -> (w451:T25)
        n258 = local read "Variable Settings"() -> (w452:T3)
        n259 = call "get_variable_start_values.vi"("error in (no error)"=w444, "Variable Settings"=w452) -> ("error out"=w447:errorcluster, "all variable names"=w449:string[], "all variable values (min or calculated)"=w450:dbl[])  [unwired: 6 in, 1 out]
        n260 = for {
          tunnel: w451 -> [w455] mode=indexing
          tunnel: w450 -> [w457]
          tunnel: w449 -> [w456]
          shift-right: [w454] -> w448
          shift-left: w447 -> [w453]
          n261 = call "set_frequency.vi"("error in"=w453, 9:w456, 10:w457, "RF Generator settings"=w455) -> ("error out"=w454:errorcluster)  [unwired: 7 in]
        }
      }
      event "Load HP83712B Settings": Value Change {
        n262 = event-data() -> ()  [unwired: 1 in, 5 out]
        n263 = property on="Load HP83712B Settings" class="Bool (strict)"(error in=w460, "Value"=FALSE) -> (error out=w459:errorcluster)  [unwired: 1 in, 1 out]
        n264 = local read "HP83712B Synthesized Signal Generator Array"() -> (w466:T25)
        n265 = local read "Variable Settings"() -> (w467:T3)
        n266 = call "get_variable_start_values.vi"("error in (no error)"=w459, "Variable Settings"=w467) -> ("error out"=w462:errorcluster, "all variable names"=w464:string[], "all variable values (min or calculated)"=w465:dbl[])  [unwired: 6 in, 1 out]
        n267 = for {
          tunnel: w466 -> [w470] mode=indexing
          tunnel: w465 -> [w472]
          tunnel: w464 -> [w471]
          shift-right: [w469] -> w463
          shift-left: w462 -> [w468]
          n268 = call "set_frequency.vi"("error in"=w468, 9:w471, 10:w472, "RF Generator settings"=w470) -> ("error out"=w469:errorcluster)  [unwired: 7 in]
        }
      }
      event "Analog Output Actions.Graph Analog Output": Value Change {
        n269 = event-data() -> ()  [unwired: 1 in, 5 out]
        n270 = local read "Analog Output Parameters"() -> (w490:T36)
        n271 = local read "Variable Settings"() -> (w491:T3)
        n272 = Unbundle By Name(w490) -> ("Total AO Time (seconds)"=w487:dbl, "Start Trigger"=w488:T55, "Samples per second"=w478:dbl)
        n273 = call "get_variable_start_values.vi"("Variable Settings"=w491) -> ("error out"=w474:errorcluster, "all variable names"=w477:string[], "all variable values (min or calculated)"=w476:dbl[])  [unwired: 7 in, 1 out]
        n274 = call <vilib>:"Eval Multi-Variable Scalar.vi"("error in (no error)"=w474, "Variables"=w477, "X Values"=w476, "formula"=w478) -> ("error out"=w473:errorcluster, "y value"=w475:dbl)
        n275 = call "AO_equations_to_waveform.vi"("variable/parameter names"=w477, "minimum/current values"=w476, "error in (no error)"=w473, "Samples per second"=w475, "Total AO Time"=w487, "Analog Output Equations for each Channel"=w488) -> ("error out"=w480:errorcluster, "Waveform Graph"=→"Waveform Graph":waveform(dbl)[])  [unwired: 3 in, 1 out]
        n276 = Unbundle By Name(w480) -> ("status"=w484:bool, "code"=w482:i32)
        n277 = Not Equal To 0?(x=w482) -> (x != 0?=w483:bool)
        n278 = Or(x=w484, y=w483) -> (x .or. y?=w481:bool)
        n279 = Not(x=w481) -> (.not. x?=→"AO Equations are valid":bool)
      }
      event "Pi Piezo Actions.Connect": Value Change {
        n280 = event-data() -> ()  [unwired: 1 in, 5 out]
        n281 = local read "PI Piezo Settings"() -> (w493:T37)
        n282 = control-ref of="PI Piezo Status"() -> (w492:refnum<vi>)
        n283 = property on="Connect" class="Bool (strict)"(error in=w496, "Value"=FALSE) -> (error out=w495:errorcluster)  [unwired: 1 in, 1 out]
        n284 = call "connect.vi"("PI Piezo Settings"=w493, "PI Piezo Status"=w492, "error in"=w495) -> ("error out"=w497:errorcluster)  [unwired: 16 in]
      }
      event "Pi Piezo Actions.Set Position": Value Change {
        n285 = event-data() -> ()  [unwired: 1 in, 5 out]
        n286 = property on="Set Position" class="Bool (strict)"(error in=w507, "Value"=FALSE) -> (error out=w501:errorcluster)  [unwired: 1 in, 1 out]
        n287 = local read "Variable Settings"() -> (w505:T3)
        n288 = local read "PI Piezo Settings"() -> (w509:T37)
        n289 = control-ref of="PI Piezo Status"() -> (w502:refnum<vi>)
        n290 = call "get_variable_start_values.vi"("error in (no error)"=w501, "Variable Settings"=w505) -> ("error out"=w500:errorcluster, "all variable names"=w504:string[], "all variable values (min or calculated)"=w503:dbl[])  [unwired: 6 in, 1 out]
        n291 = call "set_position.vi"("PI Piezo Settings"=w509, "PI Piezo Status"=w502, "current variable and parameter values"=w503, "variables and parameter names"=w504, "error in"=w500, "Save positions?"=FALSE) -> ("error out"=w508:errorcluster)  [unwired: 13 in]
      }
      event "Set Current Average Image as Background": Value Change {
        n292 = event-data() -> ()  [unwired: 1 in, 5 out]
        n293 = local read "Average of All Images from experiment"() -> (w519:T30)
        n294 = property on="Set?" class="Bool (strict)"(error in=w517, "Value"=FALSE ("Set?")) -> (error out=w516:errorcluster)  [unwired: 1 in, 1 out]
        n295 = call "IMAQ ImageToArray"("error in (no error)"=w516, "Image"=w519) -> ("Image Pixels (U16)"=→"Background Array":u16[][], "error out"=w514:errorcluster)  [unwired: 2 in, 3 out]
        n296 = property on="Set?" class="Bool (strict)"(error in=w514, "Value"=TRUE ("Set?")) -> (error out=w513:errorcluster)  [unwired: 1 in, 1 out]
      }
      event "Run Background Subtraction": Value Change {
        w533 = T56 7 items=["Grayscale (U8)", "Grayscale (I16)", "Grayscale (SGL)", "Complex (CSG)", "RGB (U32)", "HSL (U32)", "RGB (U64)", "Grayscale (U16)"] ("Image Type")
        w537 = T56 7 items=["Grayscale (U8)", "Grayscale (I16)", "Grayscale (SGL)", "Complex (CSG)", "RGB (U32)", "HSL (U32)", "RGB (U64)", "Grayscale (U16)"] ("Image Type")
        n297 = event-data() -> ()  [unwired: 1 in, 5 out]
        n298 = local read "Background Array"() -> (w523:u16[][])
        n299 = call "IMAQ Create"("Image Name"="Background", "Image Type"=w537, "error in (no error)"=w540) -> ("New Image"=w538:T30, "error out"=w539:errorcluster)  [unwired: 2 in]
        n300 = call "IMAQ ArrayToImage"("Image Pixels (U16)"=w523, "error in (no error)"=w539, "Image"=w538) -> ("error out"=w530:errorcluster, "Image Out"=→"Background Image":T30)  [unwired: 7 in]
        n301 = local read "Average of All Images from experiment"() -> (w528:T30)
        n302 = call "IMAQ Create"("Image Name"="tmp avg-background", "Image Type"=w533, "error in (no error)"=w530) -> ("New Image"=w525:T30, "error out"=w522:errorcluster)  [unwired: 2 in]
        n303 = call "IMAQ ImageToArray"("error in (no error)"=w522, "Image"=w528) -> ("Image Pixels (U16)"=w527:u16[][], "error out"=w521:errorcluster)  [unwired: 2 in, 3 out]
        n304 = Subtract(x=w527, y=w523) -> (x-y=w526:u16[][])
        n305 = local read "Image Array for whole experiment"() -> (w542:T30[][][])
        n306 = call "IMAQ ArrayToImage"("Image Pixels (U16)"=w526, "error in (no error)"=w521, "Image"=w525) -> ("error out"=w520:errorcluster, "Image Out"=→"Backgound Subtracted Average Image":T30)  [unwired: 7 in]
        n307 = local read "Set?"() -> (w535:bool)
        n308 = case shown="True" w535 {
          tunnel: w542 -> [w545 w550]
          tunnel: [w543 w549] -> w531
          tunnel: [w545 w548] -> w541
          tunnel: w520 -> [w544 w547]
          tunnel: w523 -> [_ w546]
          frame False {
            n309 = call "Display Message to User"("error in (no error)"=w544) -> ("error out"=w543:errorcluster)  [unwired: 9 in, 1 out]
          }
          frame True {
            n310 = for {
              tunnel: w550 -> [w556] mode=indexing
              tunnel: w547 -> [w555]
              tunnel: [w553] -> w549
              tunnel: [w552] -> w548 mode=indexing
              tunnel: w546 -> [w551]
              i -> [w554]
              n311 = for {
                tunnel: w556 -> [w563] mode=indexing
                tunnel: w555 -> [w562]
                tunnel: w554 -> [w561]
                tunnel: [w559] -> w553
                tunnel: [w558] -> w552 mode=indexing
                tunnel: w551 -> [w557]
                i -> [w560]
                n312 = for {
                  tunnel: w563 -> [w572] mode=indexing
                  tunnel: w562 -> [w573]
                  tunnel: w561 -> [w576]
                  tunnel: w560 -> [w575]
                  tunnel: [w564] -> w559
                  tunnel: [w567] -> w558 mode=indexing
                  tunnel: w557 -> [w571]
                  i -> [w574]
                  w580 = T56 7 items=["Grayscale (U8)", "Grayscale (I16)", "Grayscale (SGL)", "Complex (CSG)", "RGB (U32)", "HSL (U32)", "RGB (U64)", "Grayscale (U16)"] ("Image Type")
                  n313 = Format Into String(initial string="tmp %d", error in=w573, w576, w575, w574) -> (resulting string=w578:string, error out=w579:errorcluster)  [unwired: 1 in]
                  n314 = call "IMAQ Create"("Image Name"=w578, "Image Type"=w580, "error in (no error)"=w579) -> ("New Image"=w568:T30, "error out"=w566:errorcluster)  [unwired: 2 in]
                  n315 = call "IMAQ ImageToArray"("error in (no error)"=w566, "Image"=w572) -> ("Image Pixels (U16)"=w570:u16[][], "error out"=w565:errorcluster)  [unwired: 2 in, 3 out]
                  n316 = Subtract(x=w570, y=w571) -> (x-y=w569:u16[][])
                  n317 = call "IMAQ ArrayToImage"("Image Pixels (U16)"=w569, "error in (no error)"=w565, "Image"=w568) -> ("error out"=w564:errorcluster, "Image Out"=w567:T30)  [unwired: 7 in]
                }
              }
            }
          }
        }
        "Background Subtracted Image Array" <- w541
      }
      event "Load Notes from File": Value Change {
        n318 = event-data() -> ()  [unwired: 1 in, 5 out]
        n319 = Read from Text File(error in=w582) -> (text=w583:string, error out=w581:errorcluster)  [unwired: 3 in, 2 out]
        n320 = local write "Notes"(w583) -> ()
      }
      event "Save Notes to File": Value Change {
        n321 = event-data() -> ()  [unwired: 1 in, 5 out]
        n322 = local read "Notes"() -> (w585:string)
        n323 = Write to Text File(text=w585, error in=w587) -> (error out=w586:errorcluster)  [unwired: 2 in, 2 out]
      }
      event "Quit Program": Value Change {
        n324 = event-data() -> ()  [unwired: 1 in, 5 out]
        n325 = property on="Set?" class="Bool (strict)"(error in=w592, "Value"=FALSE ("Set?")) -> (error out=w591:errorcluster)  [unwired: 1 in, 1 out]
        n326 = global write "Globals.vi" "Stop"(TRUE ("Stop")) -> ()
      }
    }
    n327 = global read "Globals.vi" "Stop"() -> (w51:bool)
    n328 = call "handle_errors.vi"("error in (no error)"=w53) -> ("error out"=w52:errorcluster)  [unwired: 10 in]
  }
  n329 = local read "HP83623A Generator Settings Array"() -> (w13:T27)
  n330 = local read "PI Piezo Status"() -> (w8:T40)
  n331 = local read "DDS Settings"() -> (w14:T15)
  n332 = call "close_all.vi"("Array of Controller Status"=w8, "error in (no error)"=w10, "Hamamatsu_C9100-13.lvclass"=w12, "HP83623A Generator Settings Array"=w13, "DDS Settings"=w14) -> ("error out"=w11:errorcluster)  [unwired: 6 in]
  n333 = call "setup_gui.vi"("Enum"=T46."quit", "GUI refnum cluster"=w32, "error in (no error)"=w11) -> ("error out"=w49:errorcluster)  [unwired: 12 in]
  n334 = call <vilib>:"Simple Error Handler.vi"("type of dialog (OK msg:1)"=w50, "error in (no error)"=w49) -> ()  [unwired: 3 in, 5 out]
  "Iteration Graph" <- dbl[][] [] ("Iteration Graph")
